vi "COD主界面（列队使用）.vi"() -> (8 "多列列表框":i32(listbox))   [LabVIEW 2016, in "斯坦道CODMn.lvlib"]
uses:
  <vilib>/Analysis/6fits.llb/Curve Fitting Criteria.ctl
  <vilib>/Utility/miscctls.llb/LVPointTypeDef.ctl
  <vilib>/Utility/config.llb/Read Key (I32).vi
  <vilib>/Utility/config.llb/Read Key (Double).vi
  <vilib>/Utility/config.llb/Read Key (Boolean).vi
  <vilib>/Utility/config.llb/Write Key (I32).vi
  <vilib>/Utility/config.llb/Read Key (String).vi
  <vilib>/Utility/config.llb/Write Key (Double).vi
  <vilib>/Utility/config.llb/Write Key (Boolean).vi
  <vilib>/Utility/config.llb/Write Key (String).vi
  <vilib>/Waveform/WDTFileIO.llb/Read Waveform from File.vi
  <vilib>/ptbypt/NI_PtbyPt.lvlib
  <vilib>/Utility/config.llb/NI_LVConfig.lvlib
  <vilib>/Analysis/NI_AALPro.lvlib
panel:
  in  "方程系数 2":cluster{"K":dbl, "b":dbl, "X^2":dbl} {"X^2" format="%#.6g"; "b" format="%#.6g"; "K" format="%#.6g"}
  out "r^2 2":dbl caption="r^2" format="%.8g"
  out "拟合公式 2":string
  in  "跨度值":dbl
  in  "公式切换阈值滴定数(0-9999)":u16
  out "公式系数":dbl[](array[numeric])
  in  "存校准信息":bool
  out "标液校准时间4":timestamp format="%<%Y/%m/%d %H:%M:%S>T"
  out "标液校准时间3":timestamp format="%<%Y/%m/%d %H:%M:%S>T"
  out "标液校准时间2":timestamp format="%<%Y/%m/%d %H:%M:%S>T"
  out "标液校准时间1":timestamp format="%<%Y/%m/%d %H:%M:%S>T"
  out "零点校准时间":timestamp format="%<%Y/%m/%d %H:%M:%S>T"
  in  "远程标样校准":enum16{"标液1", "标液2", "标液3", "标液4"}(ring)
  in  "远程校准量程":enum16{"低量程", "高量程"}(ring)
  in  "温度曲线":bool
  out "温度波形时间":timestamp
  in  "历史波形 2":bool
  out "时间-温度":u16[](array[numeric]) caption="数组"
  in  "关闭 4":bool
  out "时间温度曲线":u16[](graph)
  in  "加标回收量程：":enum32{"H", "L", "AUTO"}(ring)=enum."AUTO"
  in  "定时设置":cluster{"启动":bool, "控制命令":T1, "测量参数":T2}(xcontrol)
  out "氢氧化钠":dbl
  in  "序列号变更":bool
  out "模块版本号":string
  in  "更新程序":bool
  out "进样无液体告警":bool
  out "校准内容显示":string
  out "60分钟超时报警":bool
  in  "仪器参数":bool
  out "CODMn序列号":string
  out "CODMn软件版本：":string
  in  "标样核查量程选择":enum32{"H", "L", "AUTO"}(ring)=enum."AUTO"
  in  "标样浓度":dbl
  in  "零点核查量程选择":enum32{"H", "L", "AUTO"}(ring)=enum."AUTO"
  in  "零点核查浓度":dbl
  out "序列号":string
  in  "采水泵排液时间/s:":i32
  in  "采水泵润洗时间/s:":i32
  in  "采水泵沉淀时间/s:":i32
  in  "采水泵进样时间/s:":i32
  in  "常规版/认证版":enum16{"常规版-酸性", "常规版-碱性", "认证版", "浮台版"}(ring)
  in  "释放串口":bool
  in  "打开串口":bool
  in  "保存参数":dbl[](array[numeric])
  out "报警数字":i16
  out "CODMn工作状态":T3(ring)
  out "ORP-K":string
  out "ORP-B":string
  out "ORP-A":string
  out "x = y?":bool
  out "稀释倍数解释":string
  in  "跨度量程选择":enum32{"H", "L", "AUTO"}(ring)=enum."AUTO"
  in  "跨度液浓度":dbl
  in  "水样：":dbl
  in  "蒸馏水：":dbl
  in  "标液：":dbl
  in  "零点核查样：":dbl
  in  "加标回收样：":dbl
  in  "草酸钠":dbl
  in  "高锰酸钾":dbl
  in  "硫酸":dbl
  out "量程解释说明":string
  in  "高切低阈值:":dbl
  in  "低切高阈值:":dbl
  in  "水样量程选择:":enum16{"L", "H", "自动切换测一次", "自动切换测两次"}(ring)
  in  "氢氧化钠：":dbl
  in  "标准液浓度":dbl
  in  "温度":dbl
  in  "恒温时间":dbl
  in  "当前量程：":enum16{"L", "H"}(ring)
  in  "CODMn零点核查选择":enum16{"零点核查走纯水管", "零点核查走零漂管"}(ring)
  in  "锁定按钮":bool
  in  "低量程稀释倍数:":i8=1
  in  "高量程稀释倍数:":i8=2
  out "基本量程(显示)":string
  out "测量模式(显示)":string
  out "数据时间":string
  out "断电排液标记":bool
  out "COM":string
  in  "启用5":bool
  in  "校准5":bool
  in  "泵滴定数5":dbl
  in  "浓度5":dbl
  in  "启用4":bool
  in  "校准4":bool
  in  "泵滴定数4":dbl
  in  "浓度4":dbl
  out "波形时间":timestamp
  in  "历史波形":bool
  out "滴定数-ORP值":u16[](array[numeric]) caption="数组"
  in  "关闭 3":bool
  in  "滴定曲线":bool
  out "ORP滴定曲线":u16[](graph)
  out "空白测试标记":bool
  out "跨度核查标记":bool
  in  "量程选择":enum16{"低量程", "高量程"}(ring)
  in  "手动控制":bool
  in  "选用水样":enum16{"葡萄糖", "草酸钠"}(ring)
  in  "方程系数":cluster{"K":dbl, "b":dbl, "X^2":dbl} {"X^2" format="%#.6g"; "b" format="%#.6g"; "K" format="%#.6g"}
  out "XY图":cluster{"X Values":dbl[], "Y Values":dbl[]}[](graph)
  in  "模型":enum32{"线性", "多项式", "折线"}(ring)
  out "启动时间":timestamp format="%<%Y/%m/%d %H:%M:%S>T"
  in  "关闭 2":bool
  out "r^2":dbl format="%.8g"
  out "拟合公式":string
  in  "启用3":bool
  in  "启用2":bool
  in  "启用1":bool
  in  "校准3":bool
  in  "校准2":bool
  in  "校准1":bool
  in  "泵滴定数3":dbl
  in  "泵滴定数2":dbl
  in  "泵滴定数1":dbl
  in  "浓度3":dbl
  in  "浓度2":dbl
  in  "浓度1":dbl
  in  "写入":bool
  out "零点核查标记":bool
  out "排液故障":bool
  out "进水样超量程":bool
  out "标样核查标记":bool
  out "平行样测量":bool
  out "加标回收测量":bool
  out "质控样测量":bool
  out "待机":bool
  out "校标错误":bool
  out "校零错误":bool
  out "测量错误":bool
  out "草酸钠报警":bool
  out "高锰酸钾报警":bool
  out "加热故障":bool
  out "温控器故障":bool
  out "ORP故障":bool
  out "排液标记":bool
  out "故障标记":bool
  out "校标标记":bool
  out "校零标记":bool
  out "通讯状态":bool
  out "水样测量":bool
  in  "读取":bool
  in  "返回":bool
  in  "校准配置":bool
  in  "零点泵计量数 2":dbl
  in  "标度泵计量数 2":dbl
  out "标度滴定值":dbl
  out "零点滴定值":dbl
  in  "保存":bool
  in  "关闭":bool
  out "仪器时间":timestamp format="%<%Y/%m/%d %H:%M:%S>T"
  out "秒":u16
  out "分":u16
  out "COD浓度（mg/L)":dbl format="%.2g"
  out "进样管":dbl
  out "高锰酸钾":dbl
  out "草酸钠":dbl
  out "硫酸":dbl
  out "实时ORP":dbl
  out "温度℃":dbl
  out "加热":bool
  out "搅拌":bool
  out "进硫酸":bool
  out "进加标回收样":bool
  out "进零点核查样":bool
  out "进标液":bool
  out "进蒸馏水":bool
  out "进水样":bool
  out "进草酸钠":bool
  out "进高锰酸钾":bool
  in  "启动":bool
  in  "故障清除":bool
  in  "参数配置":bool
  in  "停止":bool
  in  "单步启动":bool
  out "系统时间":timestamp
  in  "时间校准":bool
  out "模式（受控）":u16
  # "测试时长："
  # "注：遇到加热故障和排液故障时仪器不能正常启动，\n必须排查故障并点击报警清除按钮方可运行。"
  # "mg/L"
  # "基本参数设置"
  # "校零校标结果"
  # "泵计量参数设置"
  # "校零结果："
  # "校零滴定值："
  # "高锰酸钾："
  # "加热恒温温度(℃):"
  # "草酸钠："
  # "校标结果："
  # "标度滴定值："
  # "恒温时间(分钟):"
  # "零点泵计量值："
  # "硫酸："
  # "标准液浓度(mg/L):"
  # "标度泵计量值："
  # "跨度核查浓度："
  # "跨度核查量程："
  # "零点核查浓度："
  # "标样浓度："
  # "零点核查量程："
  # "标样核查量程："
  # "跨度值:"
  # "校准配置界面"
  # "测量信号值"
  # "启用"
  # "校准时间"
  # "浓度"
  # "零点"
  # "标液1"
  # "标液2"
  # "标液3"
  # "标液4"
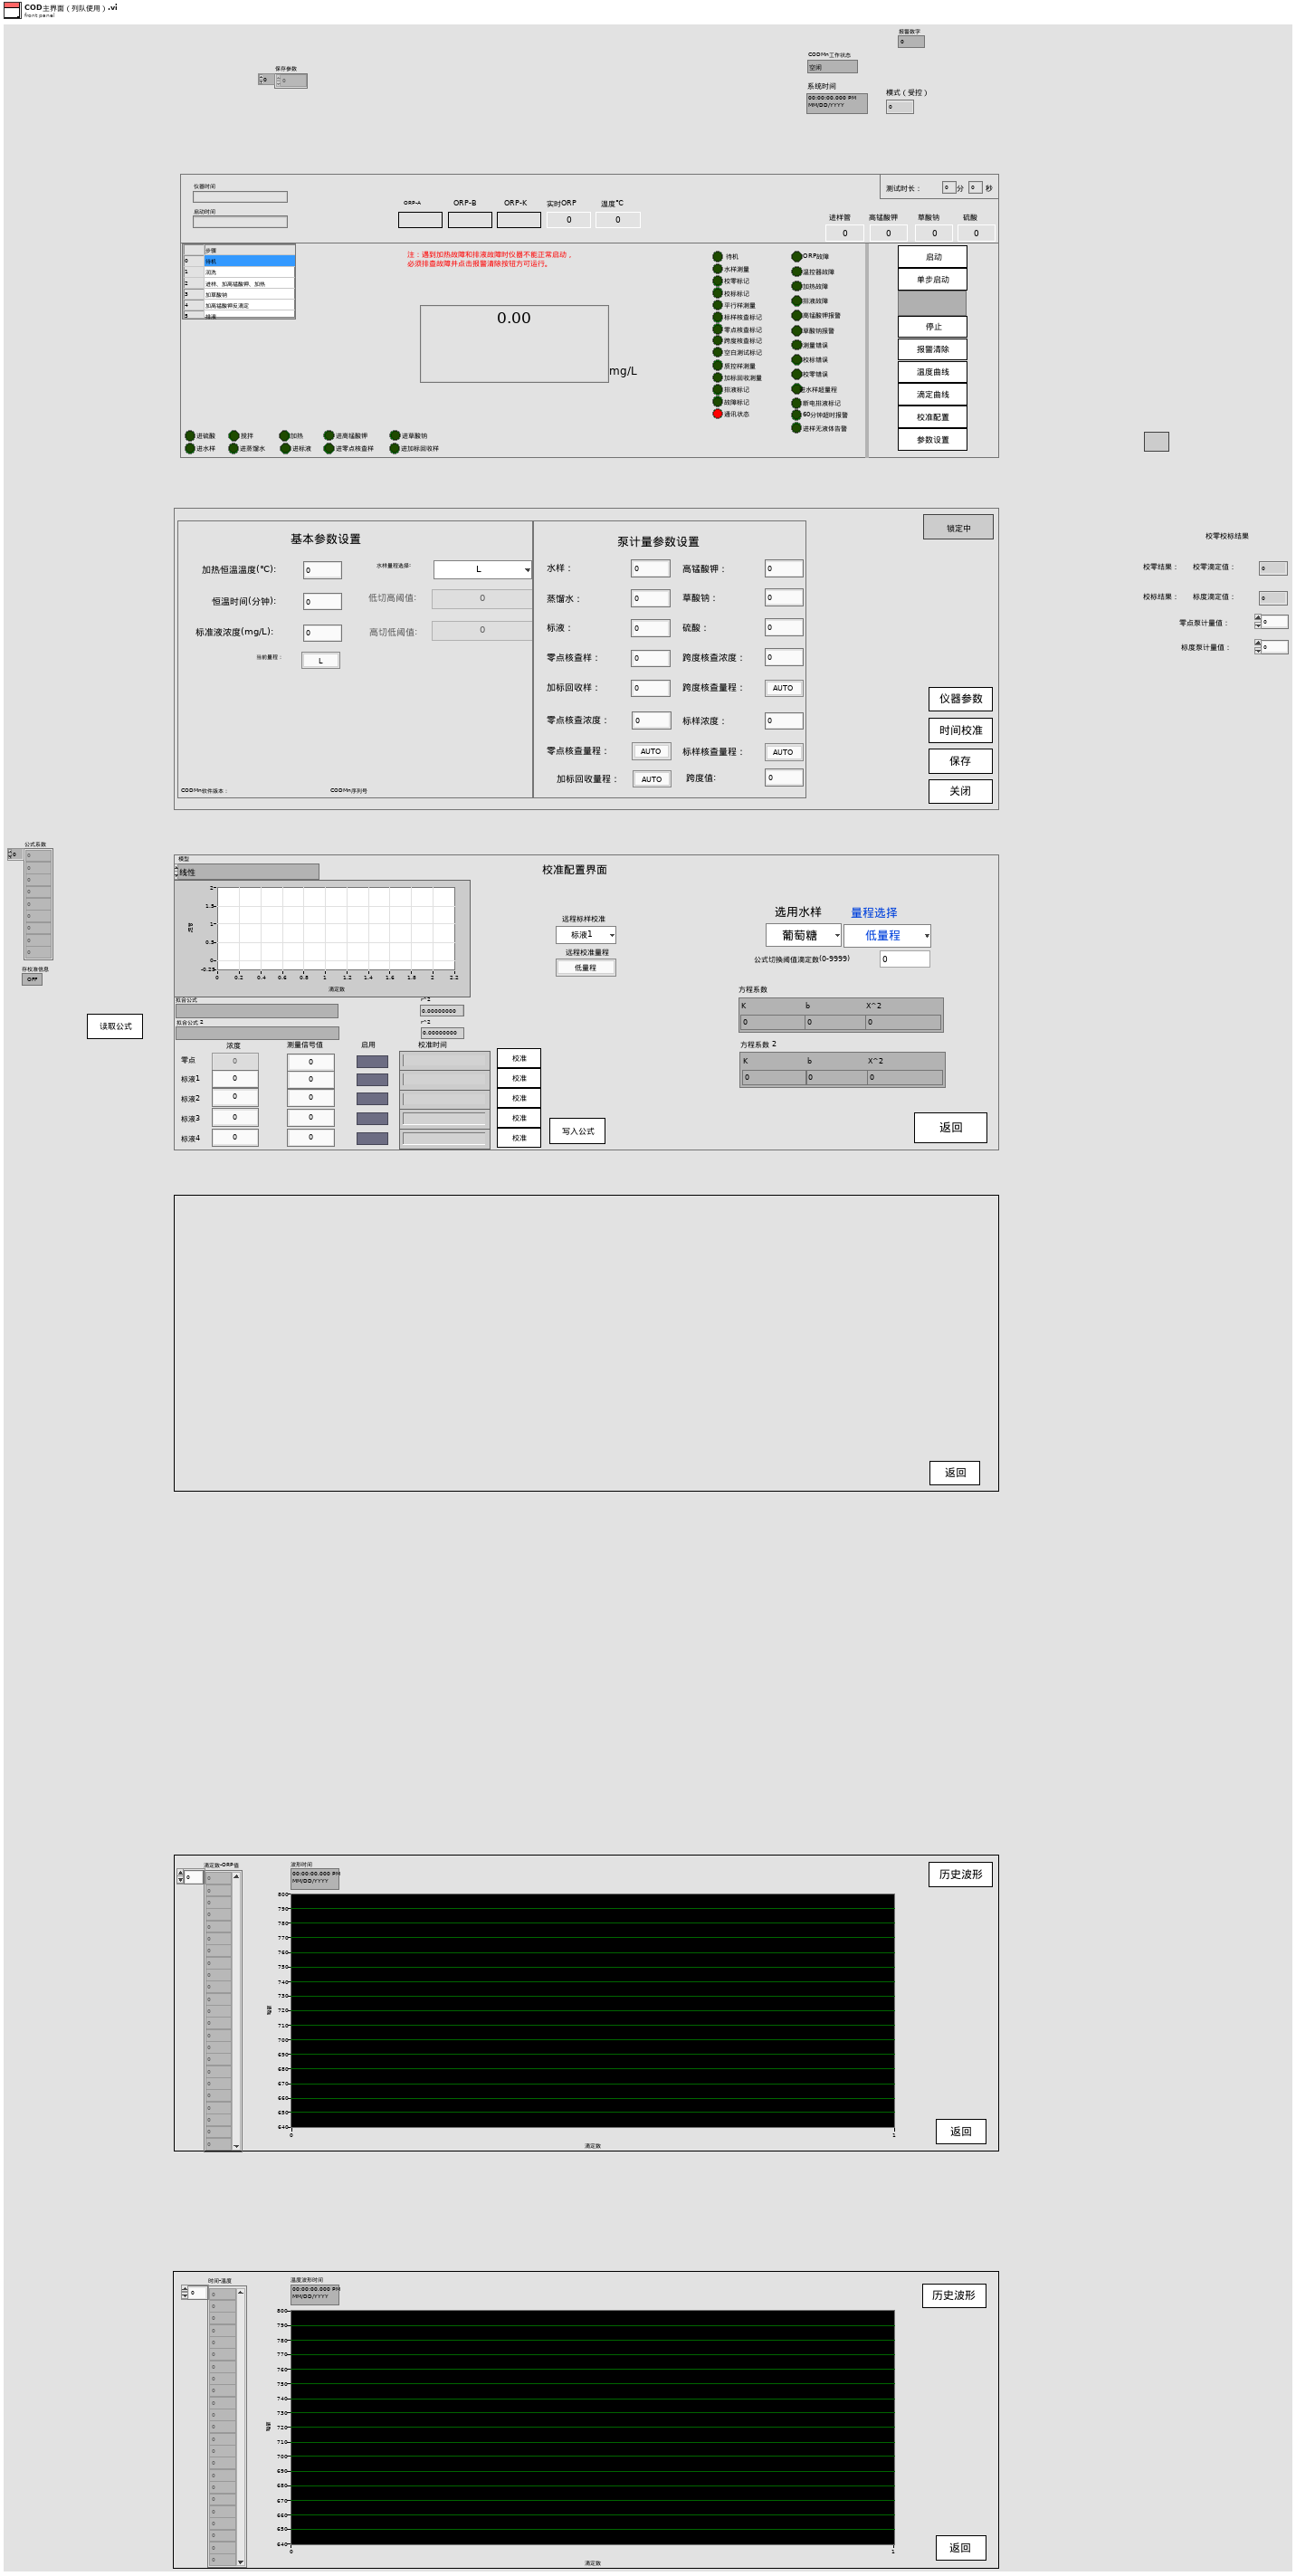
[diagram p1: front panel]
types:
  T1 = typedef "定时设置.xctl/国标控制命令.ctl" = enum16{"启动测量", "标样核查", "零点核查", "跨度核查", "空白测试", "平行样测试", "加标回收", "空白校准", "标样校准", "初始化（清洗）", "停止测试", "仪器重启", "校时", "模式设置", "测量间隔设置"}
  T2 = typedef "定时设置.xctl/测量参数.ctl" = u16
  T3 = enum16{"空闲", "水样测试", "标样核查", "零点核查", "跨度核查", "空白测试", "平行样测试", "质控样", "空白校准", "标样校准", "加标回收"}
  T4 = typedef "LVPointTypeDef.ctl" = cluster{"Horizontal":i16, "Vertical":i16}
  T5 = cluster{"Major":u16, "Minor":u16, "Fix":u16, "Build":u16}
  T6 = typedef "NI_LVConfig.lvlib/Config Data RefNum.ctl" = refnum<k1>
  T7 = cluster{"时间源选择":enum16{"系统时间源", "仪器时间源"}, "外部时间源":timestamp}
  T8 = enum32{"Bad", "Idle", "Run top level", "Running"}
  T9 = enum8{"Enabled", "Disabled", "Disabled and Grayed Out"}
  T10 = cluster{"时间":timestamp, "测量模式":string, "数据类型":string, "检测值":sgl, "单位":string, "数据标识":string, "因子编码":string, "标样参考值":sgl, "ORP-A":sgl, "ORP-B":sgl, "ORP-K":sgl, "COD滴定值":sgl, "高锰酸钾滴定数":sgl, "温度":sgl, "量程":sgl, "LastTime":timestamp, "序列号:":string, "跨度值":sgl}
  T11 = cluster{"因子编码":u32, "单位":u16, "标样参考值":sgl, "水样数据时间":timestamp, "水样实测值":sgl, "水样数据标识":string, "标样数据时间":timestamp, "标样实测值":sgl, "标样数据标识":string, "空白数据时间":timestamp, "空白实测值":sgl, "空白数据标识":string, "零点核查数据时间":timestamp, "零点核查实测值":sgl, "零点核查数据标识":string, "跨度核查数据时间":timestamp, "跨度核查实测值":sgl, "跨度核查数据标识":string, "加标回收数据时间":timestamp, "加标回收实测值":sgl, "加标回收数据标识":string, "平行样数据时间":timestamp, "平行样实测值":sgl, "平行样数据标识":string}
  T12 = cluster{"测量量程":dbl, "测量精度":dbl, "测量间隔":dbl, "消解温度":dbl, "消解时长":dbl, "空白校准时间":timestamp, "曲线截距":dbl, "曲线斜率":dbl, "测量检出限":dbl, "测量信号值":dbl, "线性相关系数":dbl, "二次多项式系数":dbl, "标样校准时间":timestamp, "稀释倍数":dbl, "三项式系数":dbl, "空白标定系数":dbl, "量程系数":dbl, "F0/ORPA":dbl, "F1/ORPB":dbl, "F2/ORPK":dbl, "F3":dbl, "F4":dbl, "F5":dbl, "F6":dbl, "F7":dbl, "X0/滴定数":dbl, "量程":dbl}
  T13 = cluster{"运行模式":enum16{"维护模式", "常规模式", "应急模式", "质控模式"}, "质控频次":enum16{"关闭", "每天", "星期一", "星期二", "星期三", "星期四", "星期五", "星期六", "星期日"}, "空白核查时间":u16, "跨度核查时间":u16, "24H周期设置":bool[]}
  T14 = cluster{"数组 2[0]":sgl, "数组 2[1]":sgl, "数组 2[2]":sgl, "数组 2[3]":sgl, "数组 2[4]":sgl, "数组 2[5]":sgl, "数组 2[6]":sgl, "数组 2[7]":sgl, "数组 2[8]":sgl, "数组 2[9]":sgl, "数组 2[10]":sgl, "数组 2[11]":sgl, "数组 2[12]":sgl, "数组 2[13]":sgl, "数组 2[14]":sgl, "数组 2[15]":sgl, "数组 2[16]":sgl, "数组 2[17]":sgl, "数组 2[18]":sgl, "数组 2[19]":sgl, "数组 2[20]":sgl, "数组 2[21]":sgl, "数组 2[22]":sgl, "数组 2[23]":sgl, "数组 2[24]":sgl, "数组 2[25]":sgl, "数组 2[26]":sgl, "数组 2[27]":sgl, "数组 2[28]":sgl, "数组 2[29]":sgl, "数组 2[30]":sgl, "数组 2[31]":sgl, "数组 2[32]":sgl, "数组 2[33]":sgl, "数组 2[34]":sgl, "数组 2[35]":sgl, "数组 2[36]":sgl, "数组 2[37]":sgl, "数组 2[38]":sgl, "数组 2[39]":sgl, "数组 2[40]":sgl, "数组 2[41]":sgl}
  T15 = typedef "NI_AALPro.lvlib/Curve Fitting Criteria.ctl" = u16
  T16 = cluster{"ORP故障":bool, "温控器故障":bool, "加热故障":bool, "高锰酸钾报警":bool, "草酸钠报警":bool, "测量错误":bool, "校零错误":bool, "校标错误":bool, " 进水样超量程":bool, "排液阀故障":bool, "60分钟超时报警":bool, "进样无液体报警":bool}
  T17 = cluster{"时间标识":timestamp, "参数":string, "日志信息":string, "流程参数":string}
  T18 = cluster{"确定":bool, "测量量程":dbl, "测量精度":dbl, "测量间隔":dbl, "消解温度":dbl, "消解时长":dbl, "空白校准时间":timestamp, "曲线截距":dbl, "曲线斜率":dbl, "测量检出限":dbl, "测量信号值":dbl, "线性相关系数":dbl, "二次多项式系数":dbl, "标样校准时间":timestamp, "稀释倍数":dbl, "三项式系数":dbl, "空白标定系数":dbl, "量程系数":dbl, "F0/ORPA":dbl, "F1/ORPB":dbl, "F2/ORPK":dbl, "F3":dbl, "F4":dbl, "F5":dbl, "F6":dbl, "F7":dbl, "X0/滴定数":dbl, "量程":dbl}
  T19 = cluster{"时间标识":timestamp, "设备":string, "日志信息":string, "流程参数":string}
  T20 = cluster{"[0]":string, "[1]":string, "[2]":string}
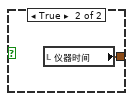
[diagram p3: hidden frame]
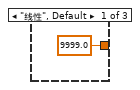
[diagram p9: hidden frame]
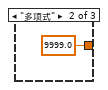
[diagram p10: hidden frame]
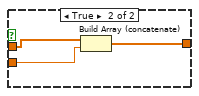
[diagram p11: hidden frame]
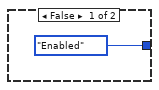
[diagram p12: hidden frame]
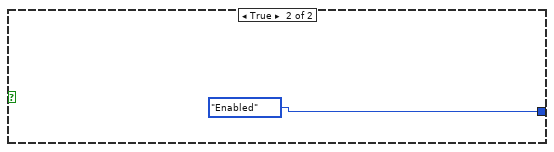
[diagram p13: hidden frame]
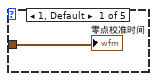
[diagram p18: hidden frame]
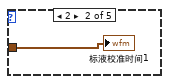
[diagram p19: hidden frame]
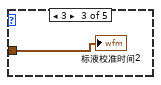
[diagram p20: hidden frame]
diagram:
  n1 = flat-sequence {
    tunnel: w3 -> [_]
    frame #0 {
      n2 = vi-ref "斯坦道CODMn.lvlib:待机状态数据存储写入和切换量程(子VI).vi"() -> (w64:refnum<vi>)
      n3 = vi-ref "斯坦道CODMn.lvlib:日志报警状态存储 (子VI).vi"() -> (w57:refnum<vi>)
      n4 = vi-ref "斯坦道CODMn.lvlib:高锰酸钾-ORP滴定曲线(子VI).vi"() -> (w44:refnum<vi>)
      n5 = property class="VI"(reference=w57, error in=errorcluster {"status"=FALSE, "code"=0, "source"=""} ("错误输出")) -> ("Name"=w56:string)  [unwired: 2 out]
      n6 = property class="VI"(reference=w44, error in=errorcluster {"status"=FALSE, "code"=0, "source"=""} ("错误输出")) -> ("Name"=w45:string)  [unwired: 2 out]
      n7 = property class="VI"(reference=w64, error in=errorcluster {"status"=FALSE, "code"=0, "source"=""} ("错误输出")) -> ("Name"=w63:string)  [unwired: 2 out]
      n8 = Open VI Reference(type specifier VI Refnum (for type only)=refnum<vi> refnum, vi path=w56, options=128 ("选项")) -> (vi reference=w40:refnum<vi>, error out=w54:errorcluster)  [unwired: 3 in]
      n9 = Open VI Reference(type specifier VI Refnum (for type only)=refnum<vi> refnum, vi path=w45, options=128 ("选项")) -> (vi reference=w43:refnum<vi>, error out=w47:errorcluster)  [unwired: 3 in]
      n10 = call-by-ref "?"(reference=w40, error in=w54) -> (reference out=w52:refnum<vi>, error out=w53:errorcluster)  [unwired: 12 in]
      n11 = call-by-ref "?"(reference=w43, error in=w47) -> (reference out=w49:refnum<vi>, error out=w48:errorcluster)  [unwired: 12 in]
      n12 = Open VI Reference(type specifier VI Refnum (for type only)=refnum<vi> refnum, vi path=w63, options=128 ("选项")) -> (vi reference=w38:refnum<vi>, error out=w61:errorcluster)  [unwired: 3 in]
      n13 = Close Reference(reference=w52, error in (no error)=w53) -> ()  [unwired: 1 out]
      n14 = call-by-ref "?"(reference=w38, error in=w61) -> (reference out=w59:refnum<vi>, error out=w60:errorcluster)  [unwired: 12 in]
      n15 = Close Reference(reference=w49, error in (no error)=w48) -> ()  [unwired: 1 out]
      n16 = Close Reference(reference=w59, error in (no error)=w60) -> ()  [unwired: 1 out]
      n17 = vi-ref "斯坦道CODMn.lvlib:时间-温度曲线(子VI).vi"() -> (w26:refnum<vi>)
      n18 = vi-ref "斯坦道CODMn.lvlib:关键参数交互.vi"() -> (w35:refnum<vi>)
      n19 = property class="VI"(reference=w35, error in=errorcluster {"status"=FALSE, "code"=0, "source"=""} ("错误输出")) -> ("Name"=w34:string)  [unwired: 2 out]
      n20 = property class="VI"(reference=w26, error in=errorcluster {"status"=FALSE, "code"=0, "source"=""} ("错误输出")) -> ("Name"=w25:string)  [unwired: 2 out]
      n21 = Open VI Reference(type specifier VI Refnum (for type only)=refnum<vi> refnum, vi path=w34, options=128 ("选项")) -> (vi reference=w36:refnum<vi>, error out=w32:errorcluster)  [unwired: 3 in]
      n22 = call-by-ref "?"(reference=w36, error in=w32, "量程选择"=enum16{"低量程", "高量程"}."低量程", "模型"=enum32{"线性", "多项式", "折线"}."线性") -> (reference out=w30:refnum<vi>, error out=w31:errorcluster)  [unwired: 10 in]
      n23 = Open VI Reference(type specifier VI Refnum (for type only)=refnum<vi> refnum, vi path=w25, options=128 ("选项")) -> (vi reference=w27:refnum<vi>, error out=w23:errorcluster)  [unwired: 3 in]
      n24 = call-by-ref "?"(reference=w27, error in=w23) -> (reference out=w21:refnum<vi>, error out=w22:errorcluster)  [unwired: 12 in]
      n25 = Close Reference(reference=w30, error in (no error)=w31) -> ()  [unwired: 1 out]
      n26 = Close Reference(reference=w21, error in (no error)=w22) -> ()  [unwired: 1 out]
    }
  }
  n27 = property on="定时设置" class="定时设置 (严格)"("引用参数"="CODMn") -> (error out=w1:errorcluster)  [unwired: 2 in, 1 out]
  n28 = flat-sequence {
    tunnel: [w68] -> w5
    tunnel: [errorcluster {"status"=FALSE, "code"=0, "source"=""} ("错误输出")] -> w3
    tunnel: [w70] -> w4
    frame #0 {
      w92 = "192.168.1.100" ("名称")
      n29 = global write "COD内部交互全局.vi" "量程切换次数"(u8 0 ("量程切换次数")) -> ()
      n30 = global write "COD内部交互全局.vi" "切换量程连续测两次"(FALSE ("切换量程连续测两次")) -> ()
      n31 = global read "COD内部交互全局.vi" "序列号:"() -> (w99:string)
      n32 = property on="窗格" class="Pane"("Origin"=T4 {"Horizontal"=0, "Vertical"=0} ("原点")) -> ()  [unwired: 2 in, 2 out]
      n33 = Empty String/Path?(string/path=w99) -> (empty?=w67:bool)
      n34 = case shown="真" w67 {
        tunnel: w99 -> [w113 _]
        tunnel: [w112 "data\\CODMnSet.ini" ("名称或相对路径")] -> w80
        frame False {
          # "与生产用上位机交互"
          n35 = Concatenate Strings("data\\" ("字符串"), "序列号" ("字符串"), w113, "Set.ini" ("名称或相对路径")) -> (w112:string)
        }
        frame True {
        }
      }
      n36 = String To IP(1:w92) -> (0:w85:u32)
      n37 = IP To String(2:w85) -> (0:w88:string)  [unwired: 1 in]
      n38 = Not Equal?(x=w92, y=w88) -> (x != y?=w93:bool)
      n39 = Concatenate Strings("\\\\" ("字符串"), w88) -> (w87:string)
      n40 = global write "CODMN外部API.vi" "ping"(w93) -> ()
      n41 = String To Path(string=w87) -> (path=w94:path)
      n42 = Build Path(base path=w94, name or relative path=w80) -> (appended path=w89:path)
      n43 = local write "量程选择"(enum16{"低量程", "高量程"}."低量程" ("量程选择")) -> ()
      n44 = local write "选用水样"(enum16{"葡萄糖", "草酸钠"}."葡萄糖" ("选用水样")) -> ()
      n45 = global write "COD内部交互全局.vi" "配置文件ini"(w80) -> ()
      n46 = case shown="真" w93 {
        tunnel: w89 -> [w103 w107]
        tunnel: [w103 w106] -> w90
        tunnel: [FALSE w105] -> w91
        frame False {
        }
        frame True {
          n47 = call <vilib>:"Check if File or Folder Exists.vi"("path"=w107) -> ("file or folder exists?"=w105:bool, "dup path"=w106:path)  [unwired: 8 in, 1 out]
        }
      }
      n48 = control-ref of="本VI"() -> (w79:refnum<vi>)
      n49 = case shown="假" w91 {
        tunnel: w90 -> [_ w111]
        tunnel: [w109 w111] -> w71
        tunnel: w80 -> [w108 _]
        frame False {
          # "本地文件地址"
          n50 = call <vilib>:"Application Directory.vi"() -> ("Application Directory"=w110:path)
          n51 = Build Path(base path=w110, name or relative path=w108) -> (appended path=w109:path)
        }
        frame True {
          # "网络共享地址"
        }
      }
      n52 = property class="VI"(reference=w79) -> ("Library.Version"=w78:T5)  [unwired: 1 in, 2 out]
      n53 = Unbundle By Name(w78) -> ("Major"=w76:u16, "Minor"=w75:u16, "Fix"=w74:u16, "Build"=w73:u16)
      n54 = Format Into String(format string="模块版本号：%d.%d.%d.%d" ("格式字符串"), w76, w75, w74, w73) -> (resulting string=→"模块版本号":string)  [unwired: 2 in, 1 out]
      n55 = global write "CODMN外部API.vi" "配置文件 path"(w71) -> ()
      n56 = call <vilib>:"Open Config Data.vi"("configuration file path"=w71) -> ("error out"=w81:errorcluster, "refnum"=w82:T6)  [unwired: 8 in, 1 out]
      n57 = vi-ref "斯坦道CODMn.lvlib:CODMn断电保存全局变量.vi"() -> (w95:refnum<vi>)
      n58 = call <userlib>:"Read Panel from INI__ogtk.vi"("error in (no error)"=w81, "VI ref"=w95, "refnum"=w82) -> ("error out"=w83:errorcluster, "refnum out"=w84:T6)  [unwired: 7 in]
      n59 = call <vilib>:"Close Config Data.vi"("error in (no error)"=w83, "refnum"=w84) -> ("error out"=w69:errorcluster)  [unwired: 8 in, 1 out]
      n60 = call <vilib>:"Clear Errors.vi"("error in (no error)"=w69) -> ("error out"=w66:errorcluster)  [unwired: 5 in, 1 out]
      n61 = Read from Text File(file (use dialog)=w71, error in=w66) -> (text=w70:string, error out=w68:errorcluster)  [unwired: 2 in, 2 out]
      "稀释倍数解释" <- "稀释倍数解释：\n稀释倍数选择1，表示不稀释\n默认低量程系数倍数1，高量程系数倍数2\n则低量程为0~8，高量程为0~16" ("稀释倍数解释")
    }
  }
  n62 = while {
    tunnel: w1 -> [_]
    stop <- FALSE stop-if-true
    n63 = Wait (ms)(milliseconds to wait=u32 500 ("等待时间（毫秒）")) -> ()  [unwired: 1 out]
    n64 = global read "COD测量模式全局.vi" "CODMn工作状态"() -> (w124:T3)
    n65 = local read "通讯状态"() -> (w118:bool)
    n66 = case shown="假" w118 {
      tunnel: [w134 w135] -> w122
      frame False {
        n67 = Get Date/Time In Seconds() -> (seconds since 1Jan1904=w134:timestamp)
      }
      frame True {
        n68 = local read "仪器时间"() -> (w135:timestamp)
      }
    }
    n69 = vi-ref "斯坦道CODMn.lvlib:CODMn测量流程.vi"() -> (w131:refnum<vi>)
    n70 = Bundle By Name(cluster=T7 {"时间源选择"=enum."系统时间源", "外部时间源"=timestamp(0 s since 1904-01-01)} ("时间源"), "时间源选择"=enum16{"系统时间源", "仪器时间源"}."仪器时间源", "外部时间源"=w122) -> (w120:T7)
    n71 = property class="VI"(reference=w131) -> ("Exec.State"=w129:T8, "Name"=w130:string)  [unwired: 1 in, 2 out]
    n72 = Not Equal?(x=w124, y=T3."空闲") -> (x != y?=w119:bool)
    n73 = property on="定时设置" class="定时设置 (严格)"("仪器状态"=w119, "时间源"=w120) -> ()  [unwired: 2 in, 2 out]
    n74 = Unbundle By Name("定时设置") -> ("启动"=w127:bool, "控制命令"=w128:T1)
    n75 = case shown="真" w127 {
      tunnel: w130 -> [_ w138]
      tunnel: w128 -> [_ w137]
      tunnel: w129 -> [_ w136]
      frame False {
      }
      frame True {
        n76 = case shown="\"Idle\"" w136 {
          tunnel: w138 -> [_ w142]
          tunnel: w137 -> [_ w139]
          frame "Bad", Default {
          }
          frame "Idle" {
            n77 = Open VI Reference(type specifier VI Refnum (for type only)=refnum<vi> refnum, vi path=w142, options=128 ("选项")) -> (vi reference=w143:refnum<vi>, error out=w144:errorcluster)  [unwired: 3 in]
            n78 = call-by-ref "开始异步调用"(reference=w143, error in=w144, "控制命令"=w139) -> (reference out=w145:refnum<vi>, error out=w146:errorcluster)  [unwired: 11 in]
            n79 = Close Reference(reference=w145, error in (no error)=w146) -> ()  [unwired: 1 out]
          }
        }
      }
    }
  }
  n80 = Obtain Queue(name (unnamed)="CODMn" ("名称（未命名）"), element data type=cluster{"命令":string} {"命令"="启用模块"} ("元素")) -> (queue out=w15:refnum<queue>, error out=w14:errorcluster)  [unwired: 3 in, 1 out]
  n81 = while {
    tunnel: [w153] -> _
    shift-right: [w151] -> _
    shift-left: w4 -> [w150]
    tunnel: w5 -> [_]
    stop <- FALSE stop-if-true
    n82 = global read "CODMN外部API.vi" "配置文件 path"() -> (w147:path)
    n83 = Wait (ms)(milliseconds to wait=u32 1000 ("等待时间（毫秒）")) -> ()  [unwired: 1 out]
    n84 = Read from Text File(file (use dialog)=w147) -> (text=w151:string, error out=w148:errorcluster)  [unwired: 3 in, 2 out]
    n85 = Not Equal?(x=w151, y=w150) -> (x != y?=w149:bool)
    n86 = case shown="真" w149 {
      tunnel: [w155 w162] -> w153
      tunnel: w147 -> [_ w156]
      tunnel: w148 -> [w155 _]
      frame False {
      }
      frame True {
        # "文件发生改变进行更新，远端和本地都更新"
        n87 = vi-ref "斯坦道CODMn.lvlib:CODMn断电保存全局变量.vi"() -> (w157:refnum<vi>)
        n88 = call <vilib>:"Open Config Data.vi"("configuration file path"=w156) -> ("error out"=w161:errorcluster, "refnum"=w160:T6)  [unwired: 8 in, 1 out]
        n89 = call <userlib>:"Read Panel from INI__ogtk.vi"("error in (no error)"=w161, "VI ref"=w157, "refnum"=w160) -> ("error out"=w159:errorcluster, "refnum out"=w158:T6)  [unwired: 7 in]
        n90 = call <vilib>:"Close Config Data.vi"("error in (no error)"=w159, "refnum"=w158) -> ("error out"=w162:errorcluster)  [unwired: 8 in, 1 out]
      }
    }
  }
  n91 = vi-ref "CODMn通讯.vi"() -> (w6:refnum<vi>)
  n92 = while {
    stop <- FALSE stop-if-true
    n93 = global read "COD内部交互全局.vi" "待机"() -> (w164:bool)
    n94 = Wait (ms)(milliseconds to wait=u32 1000 ("等待时间（毫秒）")) -> ()  [unwired: 1 out]
    n95 = case shown="假" w164 {
      tunnel: [w181 T9."Enabled" ("禁用")] -> w166
      tunnel: [w180 _] -> w165
      frame False {
        # "运行中"
        n96 = local read "校标标记"() -> (w179:bool)
        n97 = local read "校零标记"() -> (w178:bool)
        n98 = Or(x=w179, y=w178) -> (x .or. y?=w182:bool)
        n99 = case shown="真" w182 {
          tunnel: [T9."Enabled" ("禁用") T9."Disabled and Grayed Out" ("禁用")] -> w181
          tunnel: [_ TRUE] -> w180
          frame False {
          }
          frame True {
          }
        }
      }
      frame True {
      }
    }
    n100 = control-ref of="量程选择"() -> (w172:refnum<vi>)
    n101 = property on="校准内容显示" class="Str"("Visible"=w165) -> ()  [unwired: 2 in, 2 out]
    n102 = control-ref of="选用水样"() -> (w173:refnum<vi>)
    n103 = control-ref of="校准5"() -> (w167:refnum<vi>)
    n104 = control-ref of="校准4"() -> (w168:refnum<vi>)
    n105 = control-ref of="校准3"() -> (w169:refnum<vi>)
    n106 = control-ref of="校准2"() -> (w170:refnum<vi>)
    n107 = control-ref of="校准1"() -> (w171:refnum<vi>)
    n108 = Build Array(w167, w168, w169, w170, w171, w173, w172) -> (w174:refnum<vi>[])
    n109 = for {
      tunnel: w174 -> [w177] mode=indexing
      tunnel: w166 -> [w176]
      n110 = property class="Ctl"(reference=w177, "DisabledEnum"=w176) -> ()  [unwired: 1 in, 2 out]
    }
  }
  n111 = while {
    tunnel: w5 -> [_]
    stop <- FALSE stop-if-true
    # "赋值循环"
    n112 = flat-sequence {
      frame #0 {
        # "测量数据区"
        n113 = global read "COD内部交互全局.vi" "data"() -> (w326:T10)
        n114 = global read "COD测量模式全局.vi" "测量模式文字实时"() -> (w312:string)
        "测量模式(显示)" <- w312
        n115 = global read "CODMn断电保存全局变量.vi" "测量数据区"() -> (w321:T11)
        n116 = Unbundle By Name(w326) -> ("时间"=w325:timestamp, "检测值"=w324:sgl, "数据标识"=w323:string)
        n117 = case shown="\"水样测试\"" w312 {
          tunnel: w321 -> [w327 w332 w337 w342 w347 w352 w357 w362 w367 w372]
          tunnel: [w327 w331 w336 w338 w346 w351 w356 w361 w363 w371] -> w322
          tunnel: w325 -> [_ w330 w335 w341 w345 w350 w355 w360 w366 w370]
          tunnel: w324 -> [_ w329 w334 w340 w344 w349 w354 w359 w365 w369]
          tunnel: w323 -> [_ w328 w333 w339 w343 w348 w353 w358 w364 w368]
          frame "", Default {
          }
          frame "水样测试" {
            n118 = Bundle By Name(cluster=w332, "水样数据时间"=w330, "水样实测值"=w329, "水样数据标识"=w328) -> (w331:T11)
          }
          frame "标样核查" {
            n119 = Bundle By Name(cluster=w337, "标样数据时间"=w335, "标样实测值"=w334, "标样数据标识"=w333) -> (w336:T11)
          }
          frame "跨度核查" {
            n120 = Bundle By Name(cluster=w342, "跨度核查数据时间"=w341, "跨度核查实测值"=w340, "跨度核查数据标识"=w339) -> (w338:T11)
          }
          frame "零点核查" {
            n121 = Bundle By Name(cluster=w347, "零点核查数据时间"=w345, "零点核查实测值"=w344, "零点核查数据标识"=w343) -> (w346:T11)
          }
          frame "空白测试" {
            n122 = Bundle By Name(cluster=w352, "空白数据时间"=w350, "空白实测值"=w349, "空白数据标识"=w348) -> (w351:T11)
          }
          frame "加标回收" {
            n123 = Bundle By Name(cluster=w357, "加标回收数据时间"=w355, "加标回收实测值"=w354, "加标回收数据标识"=w353) -> (w356:T11)
          }
          frame "平行样" {
            n124 = Bundle By Name(cluster=w362, "平行样数据时间"=w360, "平行样实测值"=w359, "平行样数据标识"=w358) -> (w361:T11)
          }
          frame "校零" {
            n125 = Bundle By Name(cluster=w367, "空白数据时间"=w366, "空白实测值"=w365, "空白数据标识"=w364) -> (w363:T11)
          }
          frame "校标" {
            n126 = Bundle By Name(cluster=w372, "标样数据时间"=w370, "标样实测值"=w369, "标样数据标识"=w368) -> (w371:T11)
          }
        }
        n127 = Unbundle By Name(w321) -> ("水样实测值"=w318:sgl)
        n128 = feedback-in #1(w321) -> ()
        n129 = feedback #1(w321) -> (w320:T11)
        n130 = global read "CODMn断电保存全局变量.vi" "水样测试量程"() -> (w314:enum16{"L", "H"})
        n131 = Unbundle By Name(w320) -> ("水样实测值"=w319:sgl)
        n132 = feedback #2(w314) -> (w315:enum16{"L", "H"})
        n133 = feedback-in #2(w314) -> ()
        n134 = Not Equal?(x=w315, y=w314) -> (x != y?=w313:bool)
        n135 = Not Equal?(x=w318, y=w319) -> (x != y?=w317:bool)
        n136 = global write "CODMn断电保存全局变量.vi" "测量数据区"(w322) -> ()
        n137 = Or(x=w317, y=w313) -> (x .or. y?=w316:bool)
        n138 = case shown="真" w316 {
          frame False {
          }
          frame True {
            # "水样值发送改变存储本地"
            n139 = call "配置文件保存.vi"() -> ()  [unwired: 12 in]
          }
        }
      }
    }
    n140 = flat-sequence {
      frame #0 {
        # "局部变量给内部交互用全局变量"
        n141 = local read "COD浓度（mg/L)"() -> (w219:dbl)
        n142 = local read "CODMn工作状态"() -> (w222:T3)
        n143 = local read "多列列表框"() -> (w220:i32)
        n144 = local read "标准液浓度"() -> (w218:dbl)
        n145 = local read "温度℃"() -> (w213:dbl)
        n146 = local read "高锰酸钾报警"() -> (w216:bool)
        n147 = local read "断电排液标记"() -> (w215:bool)
        n148 = local read "实时ORP"() -> (w212:dbl)
        n149 = local read "故障标记"() -> (w221:bool)
        n150 = local read "高锰酸钾"() -> (w214:dbl)
        n151 = local read "待机"() -> (w217:bool)
        n152 = global write "COD内部交互全局.vi" "实时温度"(w213) -> ()
        n153 = global write "运行时序全局变量.vi" "多列列表框"(w220) -> ()
        n154 = global write "COD内部交互全局.vi" "故障标记"(w221) -> ()
        n155 = global write "COD内部交互全局.vi" "ORP显示"(w212) -> ()
        n156 = global write "COD浓度全局变量.vi" "标准液浓度"(w218) -> ()
        n157 = global write "COD内部交互全局.vi" "高锰酸钾"(w214) -> ()
        n158 = global write "COD内部交互全局.vi" "待机"(w217) -> ()
        n159 = global write "COD测量模式全局.vi" "CODMn工作状态"(w222) -> ()
        n160 = global write "COD内部交互全局.vi" "高锰酸钾报警"(w216) -> ()
        n161 = global write "COD内部交互全局.vi" "断电排液标记"(w215) -> ()
        n162 = global write "COD浓度全局变量.vi" "COD浓度（mg/L)"(w219) -> ()
      }
    }
    n163 = flat-sequence {
      frame #0 {
        # "断电保存全局给局部变量"
        n164 = global read "CODMn断电保存全局变量.vi" "高切低阈值:"() -> (w392:dbl)
        n165 = global read "CODMn断电保存全局变量.vi" "低切高阈值:"() -> (w391:dbl)
        n166 = global read "CODMn断电保存全局变量.vi" "跨度液浓度"() -> (w389:dbl)
        n167 = global read "COD内部交互全局.vi" "波形时间"() -> (→"波形时间":timestamp)
        n168 = global read "CODMn断电保存全局变量.vi" "启动时间"() -> (→"启动时间":timestamp)
        n169 = global read "CODMn断电保存全局变量.vi" "标样浓度"() -> (w387:dbl)
        n170 = global read "CODMn断电保存全局变量.vi" "CODMn跨度量程选择"() -> (w393:enum32{"H", "L", "AUTO"})
        n171 = global read "CODMn断电保存全局变量.vi" "标样核查量程选择"() -> (w384:enum32{"H", "L", "AUTO"})
        n172 = global read "CODMn断电保存全局变量.vi" "零点核查量程选择"() -> (w386:enum32{"H", "L", "AUTO"})
        n173 = global read "CODMn断电保存全局变量.vi" "加标回收量程选择"() -> (w379:enum32{"H", "L", "AUTO"})
        n174 = global read "COD内部交互全局.vi" "滴定数-ORP值"() -> (→"滴定数-ORP值":u16[])
        n175 = global read "CODMn断电保存全局变量.vi" "常规版/认证版"() -> (w388:enum16{"常规版-酸性", "常规版-碱性", "认证版", "浮台版"})
        n176 = global read "CODMn断电保存全局变量.vi" "自动切换量程:"() -> (w390:enum16{"L", "H", "自动切换测一次", "自动切换测两次"})
        n177 = global read "CODMn断电保存全局变量.vi" "零点核查浓度"() -> (w385:dbl)
        n178 = local write "高切低阈值:"(w392) -> ()
        n179 = global read "CODMn断电保存全局变量.vi" "跨度值"() -> (w373:dbl)
        n180 = local write "跨度液浓度"(w389) -> ()
        n181 = local write "低切高阈值:"(w391) -> ()
        n182 = global read "COD内部交互全局.vi" "ORP滴定曲线"() -> (→"ORP滴定曲线":u16[])
        n183 = local write "标样浓度"(w387) -> ()
        n184 = local write "标样核查量程选择"(w384) -> ()
        n185 = local write "水样量程选择:"(w390) -> ()
        n186 = local write "常规版/认证版"(w388) -> ()
        n187 = local write "零点核查浓度"(w385) -> ()
        n188 = local write "零点核查量程选择"(w386) -> ()
        n189 = local write "加标回收量程："(w379) -> ()
        n190 = local write "跨度量程选择"(w393) -> ()
        n191 = local write "跨度值"(w373) -> ()
        n192 = global read "CODMn断电保存全局变量.vi" "远程校准量程"() -> (w374:enum16{"低量程", "高量程"})
        n193 = global read "CODMn断电保存全局变量.vi" "远程标样校准"() -> (w375:enum16{"标液1", "标液2", "标液3", "标液4"})
        n194 = global read "COD内部交互全局.vi" "温度波形时间"() -> (→"温度波形时间":timestamp)
        n195 = global read "COD内部交互全局.vi" "时间温度曲线"() -> (→"时间温度曲线":u16[])
        n196 = global read "COD内部交互全局.vi" "时间-温度"() -> (→"时间-温度":u16[])
        n197 = local write "远程标样校准"(w375) -> ()
        n198 = local write "远程校准量程"(w374) -> ()
      }
    }
    n199 = flat-sequence {
      frame #0 {
        # "保存参数赋值"
        n200 = Multiply(x="温度", y=10.0) -> (x*y=w197:dbl)
        n201 = Multiply(x="标准液浓度", y=100.0) -> (x*y=w194:dbl)
        n202 = Build Array(w197, "恒温时间", w194, "氢氧化钠：", "当前量程：", "水样：", "蒸馏水：", "标液：", "零点核查样：", "加标回收样：", "高锰酸钾", "草酸钠", "硫酸", "零点泵计量数 2", "标度泵计量数 2", "高量程稀释倍数:", "低量程稀释倍数:", "CODMn零点核查选择") -> (w191:dbl[])
        n203 = local write "保存参数"(w191) -> ()
      }
    }
    n204 = flat-sequence {
      frame #0 {
        # "显示量程说明"
        n205 = global read "COD内部交互全局.vi" "通讯状态"() -> (→"通讯状态":bool)
        n206 = global read "CODMn断电保存全局变量.vi" "MB通信方式选择"() -> (w397:enum16{"串口", "TCP"})
        n207 = local read "低量程稀释倍数:"() -> (w410:i8)
        n208 = local read "高量程稀释倍数:"() -> (w400:i8)
        n209 = case shown="\"TCP\"" w397 {
          tunnel: [w413 w414] -> w401
          frame "串口", Default {
            n210 = global read "CODMn断电保存全局变量.vi" "VISA resource name"() -> (w413:refnum<visa-resource-name>)
          }
          frame "TCP" {
            n211 = global read "CODMn断电保存全局变量.vi" "IP"() -> (w414:string)
          }
        }
        "COM" <- w401
        n212 = Multiply(x=w410, y=i8 8) -> (x*y=w402:i8)
        n213 = Multiply(x=w400, y=i8 8) -> (x*y=w394:i8)
        n214 = Number To Decimal String(number=w402) -> (decimal integer string=w407:string)  [unwired: 1 in]
        n215 = Number To Decimal String(number=w394) -> (decimal integer string=w405:string)  [unwired: 1 in]
        n216 = global read "CODMn断电保存全局变量.vi" "CODMn仪器参数"() -> (w396:T12)
        n217 = Concatenate Strings("L低量程范围:0~" ("量程解释说明"), w407, "(mg/L)\n\nH高量程范围:" ("量程解释说明"), "0" ("字符串"), "~" ("量程解释说明"), w405, "(mg/L)" ("量程解释说明")) -> (→"量程解释说明":string)
        n218 = Bundle By Name(cluster=w396, "测量量程"=w394) -> (w395:T12)
        n219 = global write "CODMn断电保存全局变量.vi" "CODMn仪器参数"(w395) -> ()
      }
    }
    n220 = flat-sequence {
      frame #0 {
        # "参数赋值（只在读取参数时候改变一次）"
        n221 = global read "COD内部交互全局.vi" "读取浮台参数显示"() -> (w224:bool)
        n222 = global read "COD内部交互全局.vi" "读取浮台参数"() -> (w223:u16[])
        n223 = global read "COD内部交互全局.vi" "读取参数显示"() -> (w225:bool)
        n224 = global read "COD内部交互全局.vi" "读取参数"() -> (w226:u16[])
        n225 = case shown="真" w224 {
          tunnel: w223 -> [_ w232]
          frame False {
          }
          frame True {
            n226 = Index Array(array=w232) -> (element #1=w231:u16, element #2=w230:u16, element #3=w229:u16, element #4=w228:u16)  [unwired: 4 in]
            n227 = global write "COD内部交互全局.vi" "读取浮台参数显示"(FALSE ("读取参数显示")) -> ()
            n228 = local write "采水泵进样时间/s:"(w231) -> ()
            n229 = local write "采水泵润洗时间/s:"(w230) -> ()
            n230 = local write "采水泵沉淀时间/s:"(w229) -> ()
            n231 = local write "采水泵排液时间/s:"(w228) -> ()
          }
        }
        n232 = case shown="真" w225 {
          tunnel: w226 -> [_ w254]
          frame False {
          }
          frame True {
            n233 = Index Array(array=w254) -> (element #1=w263:u16, element #2=w233:u16, element #3=w259:u16, element #4=w237:u16, element #5=w262:u16, element #6=w261:u16, element #7=w273:u16, element #8=w272:u16, element #9=w271:u16, element #10=w270:u16, element #11=w269:u16, element #12=w268:u16, element #13=w267:u16, element #14=w266:u16, element #15=w265:u16, element #16=w257:u16, element #17=w256:u16, element #18=w255:u16, element #19=w252:u16, element #20=w251:u16, element #21=w250:u16, element #22=w249:u16, element #23=w248:u16, element #27=w244:u16, element #28=w243:u16, element #29=w242:u16, element #30=w241:u16, element #31=w240:u16)  [unwired: 31 in, 3 out]
            n234 = global write "COD内部交互全局.vi" "读取参数显示"(FALSE ("读取参数显示")) -> ()
            n235 = local write "水样："(w261) -> ()
            n236 = local write "标液："(w272) -> ()
            n237 = local write "硫酸"(w267) -> ()
            n238 = global read "CODMn断电保存全局变量.vi" "CODMn仪器参数"() -> (w236:T12)
            n239 = local write "零点核查样："(w271) -> ()
            n240 = local write "加标回收样："(w270) -> ()
            n241 = local write "当前量程："(w262) -> ()
            n242 = local write "蒸馏水："(w273) -> ()
            n243 = local write "恒温时间"(w233) -> ()
            n244 = local write "高锰酸钾"(w269) -> ()
            n245 = local write "草酸钠"(w268) -> ()
            n246 = local write "零点泵计量数 2"(w266) -> ()
            n247 = local write "标度泵计量数 2"(w265) -> ()
            n248 = local write "高量程稀释倍数:"(w257) -> ()
            n249 = local write "低量程稀释倍数:"(w256) -> ()
            n250 = local write "CODMn零点核查选择"(w255) -> ()
            n251 = Build Array(w252, w251, w250, w249, w248) -> (w247:u16[])
            n252 = Build Array(w244, w243, w242, w241, w240) -> (w239:u16[])
            n253 = Divide(x=w263, y=u16 10) -> (x/y=w234:dbl)
            n254 = Divide(x=w259, y=u16 100) -> (x/y=w258:dbl)
            n255 = local write "氢氧化钠："(w237) -> ()
            n256 = local write "温度"(w234) -> ()
            n257 = local write "标准液浓度"(w258) -> ()
            n258 = call "HexToString.vi"("数组"=w239) -> ("字符串"=w238:string)  [unwired: 10 in]
            "CODMn序列号" <- w238
            "序列号" <- w238
            n259 = call "FATEK_HexToString.vi"("数组"=w247) -> ("STRING"=w246:string[])  [unwired: 10 in]
            n260 = Bundle By Name(cluster=w236, "消解温度"=w234, "消解时长"=w233) -> (w235:T12)
            n261 = Index Array(array=w246) -> (element=→"CODMn软件版本：":string)  [unwired: 1 in]
            n262 = global write "CODMn断电保存全局变量.vi" "CODMn仪器参数"(w235) -> ()
            n263 = global write "COD内部交互全局.vi" "序列号:"(w238) -> ()
          }
        }
      }
    }
    n264 = flat-sequence {
      frame #0 {
        # "权限隐藏和显示功能"
        n265 = local read "x = y?"() -> (w420:bool)
        n266 = global read "CODMn断电保存全局变量.vi" "CODMn系统周期测试?"() -> (w417:bool)
        n267 = global read "CODMn断电保存全局变量.vi" "运行周期"() -> (w418:T13)
        n268 = property on="更新程序" class="Bool (严格)"("Visible"=w420) -> ()  [unwired: 2 in, 2 out]
        n269 = property on="释放串口" class="Bool"("Visible"=w420) -> ()  [unwired: 2 in, 2 out]
        n270 = property on="打开串口" class="Bool"("Visible"=w420) -> ()  [unwired: 2 in, 2 out]
        n271 = case shown="假" w417 {
          tunnel: w418 -> [_ w441]
          tunnel: [T9."Enabled" ("禁用") w439] -> w416
          frame False {
          }
          frame True {
            n272 = Unbundle By Name(w441) -> ("运行模式"=w440:enum16{"维护模式", "常规模式", "应急模式", "质控模式"})
            n273 = case shown="\"维护模式\", 默认" w440 {
              tunnel: [T9."Enabled" ("禁用") T9."Disabled and Grayed Out" ("禁用") T9."Disabled and Grayed Out" ("禁用") T9."Disabled and Grayed Out" ("禁用")] -> w439
              frame "维护模式", Default {
              }
              frame "常规模式" {
              }
              frame "应急模式" {
              }
              frame "质控模式" {
              }
            }
          }
        }
        n274 = property on="序列号变更" class="Bool"("Visible"=w420) -> ()  [unwired: 2 in, 2 out]
        n275 = property on="常规版/认证版" class="Enum (严格)"("Visible"=w420) -> ()  [unwired: 2 in, 2 out]
        n276 = property on="CODMn零点核查选择" class="Enum (严格)"("Visible"=w420) -> ()  [unwired: 2 in, 2 out]
        n277 = property on="低量程稀释倍数:" class="DigNum (严格)"("Visible"=w420) -> ()  [unwired: 2 in, 2 out]
        n278 = property on="稀释倍数解释" class="Str"("Visible"=w420) -> ()  [unwired: 2 in, 2 out]
        n279 = property on="高量程稀释倍数:" class="DigNum (严格)"("Visible"=w420) -> ()  [unwired: 2 in, 2 out]
        n280 = control-ref of="水样："() -> (w430:refnum<vi>)
        n281 = control-ref of="蒸馏水："() -> (w429:refnum<vi>)
        n282 = control-ref of="标液："() -> (w428:refnum<vi>)
        n283 = control-ref of="零点核查样："() -> (w427:refnum<vi>)
        n284 = control-ref of="加标回收样："() -> (w426:refnum<vi>)
        n285 = local read "水样量程选择:"() -> (w434:enum16{"L", "H", "自动切换测一次", "自动切换测两次"})
        n286 = control-ref of="量程解释说明"() -> (w424:refnum<vi>)
        n287 = control-ref of="氢氧化钠："() -> (w425:refnum<vi>)
        n288 = property on="定时设置" class="定时设置 (严格)"("DisabledEnum"=w416) -> ()  [unwired: 2 in, 2 out]
        n289 = local read "常规版/认证版"() -> (w432:enum16{"常规版-酸性", "常规版-碱性", "认证版", "浮台版"})
        n290 = Not Equal To 0?(x=w434) -> (x != 0?=w433:bool)
        n291 = control-ref of="进样管"() -> (w422:refnum<vi>)
        n292 = case shown="\"认证版\"" w432 {
          tunnel: [T9."Enabled" ("禁用") T9."Enabled" ("禁用") T9."Disabled and Grayed Out" ("禁用") T9."Enabled" ("禁用")] -> _
          tunnel: [i32[] [2] ("禁用项[]") i32[] [2] ("禁用项[]") i32[] [] ("禁用项[]") i32[] [2] ("禁用项[]")] -> _
          tunnel: [w449 w454 T9."Disabled and Grayed Out" ("禁用") w465] -> _
          tunnel: [w448 FALSE FALSE TRUE] -> w431
          tunnel: [w449 w454 T9."Disabled and Grayed Out" ("禁用") w465] -> w421
          tunnel: [w448 TRUE FALSE FALSE] -> w419
          frame "常规版-酸性", Default {
            w448 = FALSE
            w449 = T9."Enabled" ("禁用")
          }
          frame "常规版-碱性" {
            w454 = T9."Enabled" ("禁用")
          }
          frame "认证版" {
            w460 = u16 1 items=["水样测试"=1, "标样核查"=2, "零点核查"=3, "跨度核查"=4, "空白测试"=5, "平行样"=6, "加标回收"=7] ("测量模式(公式)")
            n293 = global write "CODMn断电保存全局变量.vi" "测量模式(公式)"(w460) -> ()
          }
          frame "浮台版" {
            w465 = T9."Enabled" ("禁用")
          }
        }
        n294 = Build Array(w430, w429, w428, w427, w426, w424, w425, w422) -> (w423:refnum<vi>[])
        n295 = Select(t=T9."Enabled" ("禁用"), s=w433, f=T9."Disabled and Grayed Out" ("禁用")) -> (s? t:f=w435:T9)
        n296 = for {
          tunnel: w423 -> [w447] mode=indexing
          tunnel: w421 -> [w446]
          n297 = property class="Ctl"(reference=w447, "DisabledEnum"=w446) -> ()  [unwired: 1 in, 2 out]
        }
        n298 = property on="低切高阈值:" class="DigNum (严格)"("DisabledEnum"=w435) -> ()  [unwired: 2 in, 2 out]
        n299 = property on="高切低阈值:" class="DigNum (严格)"("DisabledEnum"=w435) -> ()  [unwired: 2 in, 2 out]
        n300 = property on="采水泵润洗时间/s:" class="DigNum (严格)"("Visible"=w431) -> ()  [unwired: 2 in, 2 out]
        n301 = property on="采水泵沉淀时间/s:" class="DigNum (严格)"("Visible"=w431) -> ()  [unwired: 2 in, 2 out]
        n302 = property on="采水泵排液时间/s:" class="DigNum (严格)"("Visible"=w431) -> ()  [unwired: 2 in, 2 out]
        n303 = property on="采水泵进样时间/s:" class="DigNum (严格)"("Visible"=w431) -> ()  [unwired: 2 in, 2 out]
        n304 = property on="氢氧化钠：" class="DigNum (严格)"("Visible"=w419) -> ()  [unwired: 2 in, 2 out]
        n305 = property on="氢氧化钠" class="DigNum (严格)"("Visible"=w419) -> ()  [unwired: 2 in, 2 out]
        n306 = property on="公式切换阈值滴定数(0-9999)" class="DigNum (严格)"("Visible"=TRUE) -> ()  [unwired: 2 in, 2 out]
      }
    }
    n307 = flat-sequence {
      frame #0 {
        # "公式读取显示（只在读取公式的时候改变一次）"
        n308 = global read "COD内部交互全局.vi" "读取公式显示"() -> (w274:bool)
        n309 = case shown="真" w274 {
          frame False {
          }
          frame True {
            n310 = global write "COD内部交互全局.vi" "读取公式显示"(FALSE ("读取参数显示")) -> ()
            n311 = global read "COD内部交互全局.vi" "读取公式"() -> (w295:u16[])
            n312 = Array Subset(array=w295, index=10 ("索引"), length=84 ("长度")) -> (w283:u16[])
            n313 = Index Array(array=w283, index #1=24 ("索引")) -> (element #1=w281:u16, element #2=w280:u16)  [unwired: 1 in]
            n314 = call "浮点CDAB转换COD.vi"("数组"=w283) -> ("数组 2"=w292:sgl[])  [unwired: 10 in]
            n315 = Array To Cluster(array=w292) -> (cluster=w294:T14)
            n316 = local read "量程选择"() -> (w285:enum16{"低量程", "高量程"})
            n317 = case shown="\"高量程\"" w285 {
              tunnel: w294 -> [w303 w311]
              tunnel: [w302 w310] -> w288
              tunnel: [w301 w309] -> w287
              tunnel: [w300 w308] -> w286
              tunnel: w281 -> [w299 _]
              tunnel: w280 -> [_ w307]
              tunnel: [w298 w306] -> w277
              tunnel: [w297 w304] -> w276
              tunnel: [w296 w305] -> w275
              frame "低量程", Default {
                n318 = local write "公式切换阈值滴定数(0-9999)"(w299) -> ()
                n319 = Unbundle By Name(w303) -> ("数组 2[0]"=w302:sgl, "数组 2[1]"=w301:sgl, "数组 2[2]"=w300:sgl, "数组 2[3]"=w298:sgl, "数组 2[4]"=w297:sgl, "数组 2[5]"=w296:sgl)
              }
              frame "高量程" {
                n320 = local write "公式切换阈值滴定数(0-9999)"(w307) -> ()
                n321 = Unbundle By Name(w311) -> ("数组 2[6]"=w310:sgl, "数组 2[7]"=w309:sgl, "数组 2[8]"=w308:sgl, "数组 2[9]"=w306:sgl, "数组 2[10]"=w304:sgl, "数组 2[11]"=w305:sgl)
              }
            }
            n322 = Bundle By Name(cluster=cluster{"X":dbl, "b":dbl, "X^2":dbl} {"X"=0.0, "b"=0.0, "X^2"=0.0} ("方程系数"), "X"=w288, "b"=w287, "X^2"=w286) -> (w293:cluster{"X":dbl, "b":dbl, "X^2":dbl})
            n323 = Bundle By Name(cluster=cluster{"X":dbl, "b":dbl, "X^2":dbl} {"X"=0.0, "b"=0.0, "X^2"=0.0} ("方程系数"), "X"=w277, "b"=w276, "X^2"=w275) -> (w278:cluster{"X":dbl, "b":dbl, "X^2":dbl})
            n324 = local write "方程系数 2"(w278) -> ()
            n325 = local write "方程系数"(w293) -> ()
          }
        }
      }
    }
    n326 = Wait (ms)(milliseconds to wait=u32 1000 ("等待时间（毫秒）")) -> ()  [unwired: 1 out]
  }
  n327 = while {
    stop <- FALSE stop-if-true
    w503 = T15 0 items=["最小二乘", "最小绝对残差", "Bisquare"] ("method")
    # "计算线性、多项式公式、远程校准"
    n328 = local read "浓度1"() -> (w485:dbl)
    n329 = local read "浓度2"() -> (w504:dbl)
    n330 = local read "浓度3"() -> (w505:dbl)
    n331 = local read "浓度4"() -> (w499:dbl)
    n332 = local read "浓度5"() -> (w498:dbl)
    n333 = Build Array("泵滴定数1", "泵滴定数2", "泵滴定数3", "泵滴定数4", "泵滴定数5") -> (w469:dbl[])
    n334 = Build Array(w485, w504, w505, w499, w498) -> (w482:dbl[])
    n335 = Build Array("启用1", "启用2", "启用3", "启用4", "启用5") -> (w470:bool[])
    n336 = call "将启用的浓度作为新的浓度数组.vi"("启用布尔数组"=w470, "输入浓度数组"=w482) -> ("启用的浓度数组"=w484:dbl[])  [unwired: 13 in]
    n337 = global read "CODMN外部API.vi" "远程反控校准CODMn"() -> (w483:bool)
    n338 = call "CODMn线性公式.vi"("标液浓度"=w482, "监测浓度"=w469, "启用"=w470, "method"=w503, "模型"="模型", "精度"=6) -> ("Polynomial Coefficients 2"=w473:dbl[], "拟合方程"=w491:string, "r^2"=w472:dbl, "拟合方程 2"=w478:string, "r^2 2"=→"r^2 2":dbl, "XY图"=→"XY图":cluster{"X Values":dbl[], "Y Values":dbl[]}[], "Polynomial Coefficients"=w500:dbl[])  [unwired: 7 in]
    "拟合公式" <- w491
    "r^2" <- w472
    "拟合公式 2" <- w478
    n339 = global write "COD内部交互全局.vi" "启用的浓度数组"(w484) -> ()
    n340 = feedback #3(w478) -> (w479:string)
    n341 = feedback-in #3(w478) -> ()
    n342 = feedback #4(w491) -> (w492:string)
    n343 = feedback-in #4(w491) -> ()
    n344 = Not Equal?(x=w478, y=w479) -> (x != y?=w476:bool)
    n345 = call <vilib>:"Boolean Crossing PtByPt.vi"("direction"=enum16{"either", "false-true", "true-false"}."false-true", "input"=w483) -> ("crossing"=w481:bool)  [unwired: 1 in]
    n346 = Not Equal?(x=w491, y=w492) -> (x != y?=w477:bool)
    n347 = Or(x=w477, y=w476) -> (x .or. y?=w475:bool)
    n348 = case shown="真" w475 {
      tunnel: w500 -> [_ w524]
      tunnel: w473 -> [_ w520]
      tunnel: w472 -> [_ w516]
      tunnel: "模型" -> [_ w514]
      tunnel: w470 -> [_ w513]
      tunnel: w469 -> [_ w512]
      frame False {
      }
      frame True {
        # "当公式发生改变时赋值到右侧公式"
        n349 = case shown="\"折线\"" w514 {
          tunnel: [9999.0 ("泵滴定数5") 9999.0 ("泵滴定数5") w531] -> w515
          tunnel: w512 -> [_ _ w530]
          tunnel: w513 -> [_ _ w529]
          frame "线性", Default {
          }
          frame "多项式" {
          }
          frame "折线" {
            n350 = for {
              tunnel: w530 -> [w538] mode=indexing
              tunnel: w529 -> [w539] mode=indexing
              shift-right: [w537] -> w534
              shift-left: dbl[] [] -> [w536]
              n351 = case shown="假" w539 {
                tunnel: w538 -> [_ w543]
                tunnel: w536 -> [w540 w542]
                tunnel: [w540 w541] -> w537
                frame False {
                }
                frame True {
                  n352 = Build Array (concatenate)(w542, w543) -> (w541:dbl[])
                }
              }
            }
            n353 = Sort 1D Array(array=w534) -> (sorted array=w533:dbl[])
            n354 = Index Array(array=w533, index=1 ("索引")) -> (element=w531:dbl)
          }
        }
        n355 = Rotate 1D Array(1:w524, 2:-1 ("n")) -> (0:w525:dbl[])
        n356 = Rotate 1D Array(1:w520, 2:-1 ("n")) -> (0:w522:dbl[])
        n357 = global read "CODMn断电保存全局变量.vi" "CODMn仪器参数"() -> (w518:T12)
        n358 = Array To Cluster(array=w525) -> (cluster=w523:cluster{"[0]":dbl, "[1]":dbl, "[2]":dbl})
        n359 = Array To Cluster(array=w522) -> (cluster=w519:cluster{"[0]":dbl, "[1]":dbl, "[2]":dbl})
        n360 = Bundle By Name(cluster=w518, "线性相关系数"=w516) -> (w517:T12)
        n361 = global write "CODMn断电保存全局变量.vi" "CODMn仪器参数"(w517) -> ()
        n362 = local write "公式切换阈值滴定数(0-9999)"(w515) -> ()
        n363 = local write "方程系数"(w523) -> ()
        n364 = local write "方程系数 2"(w519) -> ()
      }
    }
    n365 = case shown="真" w481 {
      tunnel: w482 -> [_ _]
      frame False {
      }
      frame True {
        n366 = global read "CODMn断电保存全局变量.vi" "远程标样校准"() -> (w510:enum16{"标液1", "标液2", "标液3", "标液4"})
        n367 = local read "远程校准量程"() -> (w508:enum16{"低量程", "高量程"})
        n368 = Increment(x=w510) -> (x+1=w509:enum16{"标液1", "标液2", "标液3", "标液4"})
        n369 = property on="量程选择" class="Enum (严格)"("Val(Sgnl)"=w508) -> ()  [unwired: 2 in, 2 out]
        n370 = Increment(x=w509) -> (x+1=w511:enum16{"标液1", "标液2", "标液3", "标液4"})
        n371 = global write "COD内部交互全局.vi" "当前校准"(w511) -> ()
      }
    }
    n372 = Wait (ms)(milliseconds to wait=u32 1000 ("等待时间（毫秒）")) -> ()  [unwired: 1 out]
  }
  n373 = while {
    tunnel: w15 -> [w553]
    tunnel: w14 -> [w552]
    tunnel: w5 -> [_]
    stop <- FALSE stop-if-true
    # "主循环界面显示"
    n374 = flat-sequence {
      frame #0 {
        # "A，B，K"
        # "CODMn读取状态"
        n375 = global read "COD内部交互全局.vi" "ORP、时间"() -> (w688:u16[])
        n376 = To Word Integer(number=w688) -> (16bit integer=w709:i16[])
        n377 = Split 1D Array(array=w709, index=3 ("索引")) -> (first subarray=w690:i16[], second subarray=w708:i16[])
        n378 = Index Array(array=w690) -> (element #1=w694:i16, element #2=w693:i16, element #3=w692:i16)  [unwired: 3 in]
        n379 = Index Array(array=w708) -> (element #1=w703:i16, element #2=w707:i16, element #3=w706:i16, element #4=w705:i16)  [unwired: 4 in]
        n380 = To Single Precision Float(number=w705) -> (single precision float=w696:sgl)
        n381 = Build Array(w694, w693, w692) -> (w691:i16[])
        n382 = To Single Precision Float(number=w703) -> (single precision float=w702:sgl)
        n383 = To Single Precision Float(number=w707) -> (single precision float=w701:sgl)
        n384 = To Single Precision Float(number=w706) -> (single precision float=w697:sgl)
        n385 = call "HexToDate.vi"("数组"=w691) -> ("DATE"=w695:timestamp[])  [unwired: 10 in]
        n386 = Number To Decimal String(number=w701) -> (decimal integer string=→"ORP-A":string)  [unwired: 1 in]
        n387 = Number To Decimal String(number=w697) -> (decimal integer string=→"ORP-B":string)  [unwired: 1 in]
        n388 = Number To Decimal String(number=w696) -> (decimal integer string=→"ORP-K":string)  [unwired: 1 in]
        n389 = Divide(x=w702, y=sgl 100.0) -> (x/y=→"COD浓度（mg/L)":sgl)
        n390 = Index Array(array=w695) -> (element=w689:timestamp)  [unwired: 1 in]
        n391 = Format Date/Time String(seconds (now)=w689) -> (date/time string=→"数据时间":string)  [unwired: 2 in]
      }
    }
    n392 = flat-sequence {
      frame #0 {
        # "测量状态显示"
        n393 = global read "COD内部交互全局.vi" "测量状态"() -> (w602:u16[])
        n394 = To Word Integer(number=w602) -> (16bit integer=w612:i16[])
        n395 = Index Array(array=w612, index #1=0 ("索引"), index #4=3 ("索引"), index #14=13 ("索引"), index #15=14 ("索引"), index #21=20 ("索引"), index #32=31 ("索引")) -> (element #1=w616:i16, element #2=w615:i16, element #3=w614:i16, element #4=w598:i16, element #5=→"模式（受控）":i16, element #6=→"进样管":i16, element #7=→"高锰酸钾":i16, element #8=→"草酸钠":i16, element #9=→"硫酸":i16, element #10=w611:i16, element #11=w631:i16, element #12=w607:i16, element #13=→"报警数字":i16, element #14=w637:i16, element #15=w622:i16, element #16=→"多列列表框":i16, element #20=→"氢氧化钠":i16, element #21=w595:i16, element #33=→"分":i16, element #34=→"秒":i16)  [unwired: 28 in, 14 out]
        "CODMn工作状态" <- w598
        n396 = global write "COD内部交互全局.vi" "基本量程实时读取"(w595) -> ()
        n397 = Build Array(w616, w615, w614) -> (w617:i16[])
        n398 = To Single Precision Float(number=w611) -> (single precision float=→"实时ORP":sgl)
        n399 = Number To Decimal String(number=w595) -> (decimal integer string=→"基本量程(显示)":string)  [unwired: 1 in]
        n400 = Equal?(x=w607, y=u16 1) -> (x = y?=→"排液标记":bool)
        n401 = Equal?(x=w607, y=u16 2) -> (x = y?=→"断电排液标记":bool)
        n402 = Divide(x=w631, y=u16 10) -> (x/y=→"温度℃":dbl)
        n403 = Divide(x=w637, y=u16 1000) -> (x/y=→"零点滴定值":dbl)
        n404 = Divide(x=w622, y=u16 1000) -> (x/y=→"标度滴定值":dbl)
        n405 = Equal?(x=w598, y=T3."水样测试" ("CODMn工作状态")) -> (x = y?=w596:bool)
        n406 = call "HexToDate.vi"("数组"=w617) -> ("DATE"=w613:timestamp[])  [unwired: 10 in]
        n407 = case shown="真" w596 {
          tunnel: w595 -> [_ w640]
          frame False {
          }
          frame True {
            n408 = global write "CODMn断电保存全局变量.vi" "水样测试量程"(w640) -> ()
          }
        }
        n409 = Index Array(array=w613) -> (element=→"仪器时间":timestamp)  [unwired: 1 in]
      }
    }
    n410 = flat-sequence {
      frame #0 {
        # "报警状态显示"
        n411 = global read "COD内部交互全局.vi" "报警点位"() -> (w655:bool[])
        n412 = Index Array(array=w655, index #1=0 ("索引")) -> (element #1=w652:bool, element #2=w651:bool, element #3=w650:bool, element #4=w649:bool, element #5=w648:bool, element #6=w647:bool, element #7=w646:bool, element #8=w645:bool, element #9=w644:bool, element #11=w643:bool, element #13=w642:bool, element #14=w641:bool)  [unwired: 13 in, 2 out]
        "ORP故障" <- w652
        "温控器故障" <- w651
        "加热故障" <- w644
        "高锰酸钾报警" <- w646
        "草酸钠报警" <- w645
        "测量错误" <- w650
        "校零错误" <- w649
        "校标错误" <- w648
        "进水样超量程" <- w647
        "排液故障" <- w643
        "60分钟超时报警" <- w642
        "进样无液体告警" <- w641
        n413 = Compound Arithmetic op=OR ("复合运算")(w652, w651, w644, w646, w645, w650, w648, w649, w647, w643, w642) -> (→"故障标记":bool)
        n414 = Bundle By Name(cluster=T16 {"ORP故障"=FALSE, "温控器故障"=FALSE, "加热故障"=FALSE, "高锰酸钾报警"=FALSE, "草酸钠报警"=FALSE, "测量错误"=FALSE, "校零错误"=FALSE, "校标错误"=FALSE, " 进水样超量程"=FALSE, "排液阀故障"=FALSE, "60分钟超时报警"=FALSE, "进样无液体报警"=FALSE} ("报警簇"), "ORP故障"=w652, "温控器故障"=w651, "加热故障"=w644, "高锰酸钾报警"=w646, "草酸钠报警"=w645, "测量错误"=w650, "校零错误"=w649, "校标错误"=w648, "进水样超量程"=w647, "排液阀故障"=w643, "60分钟超时报警"=w642, "进样无液体报警"=w641) -> (w653:T16)
        n415 = global write "COD内部交互全局.vi" "报警簇"(w653) -> ()
      }
    }
    n416 = flat-sequence {
      frame #0 {
        # "CODMn读取状态"
        n417 = global read "COD内部交互全局.vi" "温度"() -> (w685:bool[])
        n418 = global read "COD内部交互全局.vi" "M输出点"() -> (w684:bool[])
        n419 = Index Array(array=w685) -> (element=→"加热":bool)  [unwired: 1 in]
        n420 = Index Array(array=w684) -> (element #1=→"搅拌":bool, element #4=→"进水样":bool, element #5=→"进蒸馏水":bool, element #6=→"进标液":bool, element #7=→"进零点核查样":bool, element #8=→"进加标回收样":bool, element #9=→"进高锰酸钾":bool, element #10=→"进草酸钠":bool, element #11=→"进硫酸":bool)  [unwired: 11 in, 2 out]
      }
    }
    n421 = flat-sequence {
      frame #0 {
        # "工作状态显示"
        n422 = local read "CODMn工作状态"() -> (w563:T3)
        n423 = case shown="\"标样校准\"" w563 {
          tunnel: [_ u16 0 ("y") u16 1 ("y") u16 2 ("y") u16 3 ("y") u16 4 ("y") u16 6 ("y") _ u16 7 ("y") u16 8 ("y") u16 5 ("y")] -> w562
          frame "空闲", Default {
          }
          frame "水样测试" {
          }
          frame "标样核查" {
          }
          frame "零点核查" {
          }
          frame "跨度核查" {
          }
          frame "空白测试" {
          }
          frame "平行样测试" {
          }
          frame "质控样" {
          }
          frame "空白校准" {
          }
          frame "标样校准" {
          }
          frame "加标回收" {
          }
        }
        n424 = Equal?(x=w563, y=u16 8) -> (x = y?=→"校零标记":bool)
        n425 = Equal?(x=w563, y=u16 4) -> (x = y?=→"跨度核查标记":bool)
        n426 = Equal?(x=w563, y=u16 0) -> (x = y?=→"待机":bool)
        n427 = Equal?(x=w563, y=u16 3) -> (x = y?=→"零点核查标记":bool)
        n428 = Equal?(x=w563, y=u16 7) -> (x = y?=→"质控样测量":bool)
        n429 = Equal?(x=w563, y=u16 1) -> (x = y?=→"水样测量":bool)
        n430 = Equal?(x=w563, y=u16 2) -> (x = y?=→"标样核查标记":bool)
        n431 = Equal?(x=w563, y=u16 6) -> (x = y?=→"平行样测量":bool)
        n432 = Equal?(x=w563, y=u16 9) -> (x = y?=→"校标标记":bool)
        n433 = Equal?(x=w563, y=u16 5) -> (x = y?=→"空白测试标记":bool)
        n434 = Equal?(x=w563, y=u16 10) -> (x = y?=→"加标回收测量":bool)
        n435 = global write "COD内部交互全局.vi" "测量模式数字"(w562) -> ()
      }
    }
    n436 = Get Date/Time In Seconds() -> (seconds since 1Jan1904=→"系统时间":timestamp)
    n437 = First Call?() -> (First Call?: T/F=w551:bool)
    n438 = Wait (ms)(milliseconds to wait=u32 1000 ("等待时间（毫秒）")) -> ()  [unwired: 1 out]
    n439 = case shown="真" w551 {
      tunnel: w553 -> [w659 w670]
      tunnel: w552 -> [w658 w669]
      tunnel: [w659 w661] -> w549
      tunnel: [w658 w660] -> w548
      frame False {
      }
      frame True {
        n440 = Bundle By Name(cluster=cluster{"命令":string} {"命令"=""} ("元素"), "命令"="CODMn读取参数" ("名称（未命名）")) -> (w673:cluster{"命令":string})
        n441 = Enqueue Element(queue=w670, element=w673, timeout in ms (-1)=1000 ("超时毫秒(-1)"), error in (no error)=w669) -> (queue out=w663:refnum<queue>, error out=w662:errorcluster)  [unwired: 1 out]
        n442 = Bundle By Name(cluster=cluster{"命令":string} {"命令"=""} ("元素"), "命令"="CODMn读取公式" ("名称（未命名）")) -> (w664:cluster{"命令":string})
        n443 = Enqueue Element(queue=w663, element=w664, timeout in ms (-1)=1000 ("超时毫秒(-1)"), error in (no error)=w662) -> (queue out=w661:refnum<queue>, error out=w660:errorcluster)  [unwired: 1 out]
      }
    }
    n444 = Get Queue Status(queue=w549, error in (no error)=w548) -> (queue out=w545:refnum<queue>, error out=w544:errorcluster, # elements in queue=w547:i32)  [unwired: 1 in, 5 out]
    n445 = Equal To 0?(x=w547) -> (x = 0?=w546:bool)
    n446 = case shown="真" w546 {
      tunnel: w545 -> [_ w557]
      tunnel: w544 -> [_ w556]
      frame False {
      }
      frame True {
        n447 = Bundle By Name(cluster=cluster{"命令":string} {"命令"=""} ("元素"), "命令"="CODMn读取" ("名称（未命名）")) -> (w559:cluster{"命令":string})
        n448 = Enqueue Element(queue=w557, element=w559, timeout in ms (-1)=1000 ("超时毫秒(-1)"), error in (no error)=w556) -> ()  [unwired: 3 out]
      }
    }
  }
  n449 = while {
    tunnel: w15 -> [w712]
    tunnel: w14 -> [w711]
    stop <- FALSE stop-if-true
    # "主线事件"
    n450 = event shown="[21] \"浓度1\", \"浓度2\", \"浓度3\", \"泵滴定数1\", \"泵滴定数2\", \"泵滴定数3\", \"启用1\", \"启用2\", \"启用3\", \"浓度4\", \"浓度5\", \"泵滴定数4\", \"泵滴定数5\", \"启用4\", \"启用5\", \"标液校准时间1\", \"标液校准时间2\", \"标液校准时间3\", \"标液校准时间4\", \"零点校准时间\": 值改变" {
      selector: _ -> [_ _ _ _ _ _ _ _ _ _ _ _ _ _ _ _ _ _ _ _ _ _ _ _ _ _ _ _ _ _ _]
      dyn-events: _ -> [_ _ _ _ _ _ _ _ _ _ _ _ _ _ _ _ _ _ _ _ _ _ _ _ _ _ _ _ _ _ _]
      timeout: _ -> [_ _ _ _ _ _ _ _ _ _ _ _ _ _ _ _ _ _ _ _ _ _ _ _ _ _ _ _ _ _ _]
      tunnel: w712 -> [_ _ _ _ _ w803 _ _ w836 w974 w1100 _ _ _ _ _ _ _ w1313 _ _ _ w1576 _ _ _ w1640 w1647 w1669 w1712 _]
      tunnel: w711 -> [_ _ _ _ _ w802 _ _ w835 w973 w1099 _ _ _ _ _ _ _ w1310 _ _ _ w1575 _ _ _ w1639 w1646 w1668 w1711 _]
      event "单步启动": Value Change {
        n451 = event-data() -> ()  [unwired: 1 in, 6 out]
        n452 = call "CODMn手动控制框.vi"() -> ()  [unwired: 12 in]
      }
      event "启动": Mouse Down {
        n453 = event-data() -> ()  [unwired: 1 in, 8 out]
        n454 = global read "COD内部交互全局.vi" "基本量程实时读取"() -> (w716:enum16{"L", "H", "AUTO"})
        n455 = call "启动测量模式选择对话框.vi"("量程选择"=w716) -> ("标样浓度输出"=w714:dbl, "量程选择输出"=w715:enum16{"L", "H", "AUTO"}, "启动选择输出"=w720:u16)  [unwired: 8 in]
        n456 = Not Equal?(x=w720, y=u16 8) -> (x != y?=w717:bool)
        n457 = Not Equal?(x=w720, y=u16 7) -> (x != y?=w718:bool)
        n458 = And(x=w718, y=w717) -> (x .and. y?=w722:bool)
        n459 = case shown="真" w722 {
          tunnel: w720 -> [_ w737]
          tunnel: w715 -> [_ w728]
          tunnel: w714 -> [_ w727]
          frame False {
            n460 = One Button Dialog(message="请到校准配置里面进行校准操作！" ("消息")) -> ()  [unwired: 1 in, 1 out]
          }
          frame True {
            n461 = Not Equal?(x=w737, y=u16 9) -> (x != y?=w732:bool)
            n462 = case shown="\"H\"" w728 {
              tunnel: [w738 w742 errorcluster {"status"=FALSE, "code"=0, "source"=""} ("error out")] -> w726
              frame "L", Default {
                n463 = call "CODMnMB_api.vi"("STEP"=enum16{"open", "read", "write", "close"}."write", "values"=u16[] [0], "starting address"=u16 4276) -> ("error out"=w738:errorcluster)  [unwired: 6 in, 2 out]
              }
              frame "H" {
                n464 = call "CODMnMB_api.vi"("STEP"=enum16{"open", "read", "write", "close"}."write", "values"=u16[] [1], "starting address"=u16 4276) -> ("error out"=w742:errorcluster)  [unwired: 6 in, 2 out]
              }
              frame "AUTO" {
              }
            }
            n465 = global write "CODMN外部API.vi" "手动启动CODMn"(w732) -> ()
            n466 = call "单步测试一键复位.vi"("Error in"=w726) -> ("error out"=w725:errorcluster)  [unwired: 10 in]
            n467 = call <vilib>:"Clear Errors.vi"("error in (no error)"=w725) -> ("error out"=w724:errorcluster)  [unwired: 5 in, 1 out]
            n468 = case shown="0" w737 {
              tunnel: [u16 4608 ("address") u16 4608 ("address") u16 4608 ("address") u16 4608 ("address") u16 4608 ("address") u16 4608 ("address") u16 4608 ("address") u16 4608 ("address") u16 4608 ("address") u16 4608 ("address")] -> w730
              tunnel: [u16 1 ("address") u16 2 ("address") u16 3 ("address") u16 4 ("address") u16 5 ("address") u16 7 ("address") u16 6 ("address") u16 8 ("address") u16 9 ("address") u16 0 ("address")] -> w734
              tunnel: w727 -> [_ w750 _ _ _ _ _ _ _ _]
              frame 0 {
              }
              frame 1 {
                n469 = property on="标样浓度" class="DigNum (严格)"("Val(Sgnl)"=w750) -> ()  [unwired: 2 in, 2 out]
              }
              frame 2 {
              }
              frame 3 {
              }
              frame 4 {
              }
              frame 5 {
              }
              frame 6 {
              }
              frame 7 {
              }
              frame 8 {
              }
              frame 9, Default {
              }
            }
            n470 = Insert Into Array(array=u16[] [] ("values"), index=0 ("索引"), new element=w734) -> (w729:u16[])
            n471 = call "CODMnMB_api.vi"("STEP"=enum16{"open", "read", "write", "close"}."write", "Error in"=w724, "values"=w729, "starting address"=w730) -> ()  [unwired: 5 in, 3 out]
          }
        }
      }
      event "停止": Value Change {
        n472 = event-data() -> ()  [unwired: 1 in, 6 out]
        n473 = Two Button Dialog(message="确认是否停止？" ("消息"), 1:"否" ("F按钮名称（“取消”）"), 2:"是" ("T按钮名称（“确定”）")) -> (T button?=w770:bool)
        n474 = case shown="真" w770 {
          frame False {
          }
          frame True {
            n475 = Obtain Notifier(name (unnamed)="CODMn" ("名称（未命名）"), notification data type=FALSE) -> (notifier out=w776:refnum<notifier>, error out=w774:errorcluster)  [unwired: 2 in, 1 out]
            n476 = Send Notification(notification=TRUE ("通知"), notifier=w776, error in (no error)=w774) -> (notifier out=w773:refnum<notifier>, error out=w772:errorcluster)
            n477 = Release Notifier(notifier=w773, error in (no error)=w772) -> ()  [unwired: 1 in, 3 out]
            n478 = call "CODMnMB_api.vi"("STEP"=enum16{"open", "read", "write", "close"}."write", "values"=u16[] [11], "starting address"=u16 4608) -> ()  [unwired: 6 in, 3 out]
          }
        }
      }
      event "手动控制": Value Change {
        n479 = event-data() -> ()  [unwired: 1 in, 6 out]
        n480 = call "数字密码键盘.vi"() -> ("NewNumber"=w782:sgl)  [unwired: 1 in]
        n481 = Equal?(x=w782, y=8.0) -> (x = y?=w783:bool)
        n482 = case shown="假" w783 {
          frame False {
            n483 = call "窗口弹出对话框(子VI).vi"("消息"="密码错误") -> ()  [unwired: 10 in, 1 out]
          }
          frame True {
          }
        }
      }
      event "锁定按钮": Mouse Down {
        n484 = event-data() -> ("CtlRef"=w788:refnum<vi>)  [unwired: 1 in, 7 out]
        n485 = property class="Bool (严格)"(reference=w788) -> ("Value"=w787:bool)  [unwired: 1 in, 2 out]
        n486 = case shown="真" w787 {
          selector: w787 -> [w789 _]
          tunnel: [w789 w793] -> w786
          frame False {
          }
          frame True {
            n487 = call "数字密码键盘.vi"() -> ("NewNumber"=w790:sgl)  [unwired: 1 in]
            n488 = Equal?(x=w790, y=23506.0) -> (x = y?=w794:bool)
            n489 = Equal?(x=w790, y=8.0) -> (x = y?=w791:bool)
            n490 = Or(x=w794, y=w791) -> (x .or. y?=w793:bool)
            n491 = case shown="假" w793 {
              selector: w793 -> [w797 _]
              frame False {
                n492 = local write "锁定按钮"(w797) -> ()
                n493 = One Button Dialog(message="密码错误!" ("消息")) -> ()  [unwired: 1 in, 1 out]
              }
              frame True {
                n494 = One Button Dialog(message="解锁成功!" ("消息")) -> ()  [unwired: 1 in, 1 out]
              }
            }
          }
        }
        "x = y?" <- w786
      }
      event "参数配置": Value Change {
        (unwired) u16 20 ("number of holding registers")
        (unwired) u16 4272 ("starting address")
        n495 = event-data() -> ()  [unwired: 1 in, 6 out]
        n496 = global read "CODMN外部API.vi" "ping"() -> (w801:bool)
        n497 = property on="窗格" class="Pane"("Origin"=T4 {"Horizontal"=0, "Vertical"=650} ("原点")) -> ()  [unwired: 2 in, 2 out]
        n498 = case shown="假" w801 {
          tunnel: [w813 w816] -> w800
          frame False {
            n499 = global read "COD内部交互全局.vi" "配置文件ini"() -> (w815:string)
            n500 = call <vilib>:"Application Directory.vi"() -> ("Application Directory"=w814:path)
            n501 = Build Path(base path=w814, name or relative path=w815) -> (appended path=w813:path)
          }
          frame True {
            n502 = global read "CODMN外部API.vi" "配置文件 path"() -> (w816:path)
          }
        }
        n503 = Bundle By Name(cluster=cluster{"命令":string} {"命令"=""} ("元素"), "命令"="CODMn读取参数" ("名称（未命名）")) -> (w804:cluster{"命令":string})
        n504 = call <vilib>:"Open Config Data.vi"("configuration file path"=w800) -> ("error out"=w810:errorcluster, "refnum"=w807:T6)  [unwired: 8 in, 1 out]
        n505 = Enqueue Element(queue=w803, element=w804, error in (no error)=w802) -> ()  [unwired: 1 in, 3 out]
        n506 = vi-ref "斯坦道CODMn.lvlib:CODMn断电保存全局变量.vi"() -> (w808:refnum<vi>)
        n507 = call <userlib>:"Read Panel from INI__ogtk.vi"("error in (no error)"=w810, "VI ref"=w808, "refnum"=w807) -> ("error out"=w811:errorcluster, "refnum out"=w809:T6)  [unwired: 7 in]
        n508 = call <vilib>:"Close Config Data.vi"("error in (no error)"=w811, "refnum"=w809) -> ("error out"=w799:errorcluster)  [unwired: 8 in, 1 out]
        n509 = call <vilib>:"Clear Errors.vi"("error in (no error)"=w799) -> ()  [unwired: 5 in, 2 out]
      }
      event "保存": Mouse Down {
        n510 = event-data() -> ()  [unwired: 1 in, 8 out]
        n511 = local read "通讯状态"() -> (w817:bool)
        n512 = Two Button Dialog(message="确定保存参数，保存参数将会替换原有参数！" ("消息")) -> (T button?=w819:bool)  [unwired: 2 in]
        n513 = case shown="真" w819 {
          tunnel: w817 -> [_ w820]
          frame False {
          }
          frame True {
            n514 = case shown="真" w820 {
              frame False {
                n515 = One Button Dialog(message="保存失败，当前无通讯！" ("消息")) -> ()  [unwired: 1 in, 1 out]
              }
              frame True {
                n516 = One Button Dialog(message="参数保存成功！" ("消息")) -> ()  [unwired: 1 in, 1 out]
                n517 = Build Array("采水泵进样时间/s:", "采水泵润洗时间/s:", "采水泵沉淀时间/s:", "采水泵排液时间/s:") -> (w823:i32[])
                n518 = call "CODMnMB_api.vi"("STEP"=enum16{"open", "read", "write", "close"}."write", "values"="保存参数", "starting address"=u16 4272) -> ("error out"=w829:errorcluster)  [unwired: 6 in, 2 out]
                n519 = call "CODMnMB_api.vi"("STEP"=enum16{"open", "read", "write", "close"}."write", "Error in"=w829, "values"=w823, "starting address"=u16 5596) -> ()  [unwired: 5 in, 3 out]
              }
            }
          }
        }
      }
      event "常规版/认证版": Value Change {
        n520 = event-data() -> ()  [unwired: 1 in, 6 out]
        n521 = flat-sequence {
          frame #0 {
            n522 = global write "CODMn断电保存全局变量.vi" "常规版/认证版"("常规版/认证版") -> ()
          }
          frame #1 {
            n523 = call "配置文件保存.vi"() -> ()  [unwired: 12 in]
          }
        }
      }
      event "校准配置": Value Change {
        w849 = "量程选择" ("section")
        n524 = event-data() -> ()  [unwired: 1 in, 6 out]
        n525 = global read "CODMN外部API.vi" "ping"() -> (w853:bool)
        n526 = property on="窗格" class="Pane"("Origin"=T4 {"Horizontal"=0, "Vertical"=1300} ("原点")) -> ()  [unwired: 2 in, 2 out]
        n527 = case shown="假" w853 {
          tunnel: [w931 w934] -> w852
          frame False {
            n528 = global read "COD内部交互全局.vi" "配置文件ini"() -> (w933:string)
            n529 = call <vilib>:"Application Directory.vi"() -> ("Application Directory"=w932:path)
            n530 = Build Path(base path=w932, name or relative path=w933) -> (appended path=w931:path)
          }
          frame True {
            n531 = global read "CODMN外部API.vi" "配置文件 path"() -> (w934:path)
          }
        }
        n532 = Bundle By Name(cluster=cluster{"命令":string} {"命令"=""} ("元素"), "命令"="CODMn读取公式" ("名称（未命名）")) -> (w837:cluster{"命令":string})
        n533 = Enqueue Element(queue=w836, element=w837, error in (no error)=w835) -> ()  [unwired: 1 in, 3 out]
        n534 = call <vilib>:"Open Config Data.vi"("configuration file path"=w852) -> ("error out"=w870:errorcluster, "refnum"=w871:T6)  [unwired: 8 in, 1 out]
        n535 = call-poly <vilib>:"Read Key.vi"("section"="CODMn模型选择" ("key"), "error in (no error)"=w870, "key"="线性和多项式", "refnum"=w871) -> ("error out"=w867:errorcluster, "value"=w869:i32, "refnum out"=w868:T6)  [unwired: 4 in, 1 out]
        n536 = local write "模型"(w869) -> ()
        n537 = call-poly <vilib>:"Read Key.vi"("section"="标线选择", "error in (no error)"=w867, "key"="选用水样", "refnum"=w868) -> ("error out"=w850:errorcluster, "value"=w854:i32, "refnum out"=w851:T6)  [unwired: 4 in, 1 out]
        n538 = local write "选用水样"(w854) -> ()
        n539 = case shown="0, 默认" w854 {
          tunnel: ["葡萄糖标线" ("section") "草酸钠标线" ("section")] -> w876
          frame 0, Default {
          }
          frame 1 {
          }
        }
        n540 = call-poly <vilib>:"Read Key.vi"("section"=w849, "error in (no error)"=w850, "key"=w849, "refnum"=w851) -> ("error out"=w847:errorcluster, "value"=w846:i32, "refnum out"=w848:T6)  [unwired: 4 in, 1 out]
        n541 = local write "量程选择"(w846) -> ()
        n542 = case shown="2" w846 {
          tunnel: ["低量程" "高量程" "0-2量程"] -> w875
          frame 0, Default {
          }
          frame 1 {
          }
          frame 2 {
          }
        }
        n543 = Concatenate Strings(w876, w875) -> (w874:string)
        n544 = call-poly <vilib>:"Read Key.vi"("section"=w874, "error in (no error)"=w847, "key"="浓度1", "refnum"=w848) -> ("error out"=w901:errorcluster, "value"=w899:dbl, "refnum out"=w900:T6)  [unwired: 4 in, 1 out]
        n545 = local write "浓度1"(w899) -> ()
        n546 = call-poly <vilib>:"Read Key.vi"("section"=w874, "error in (no error)"=w901, "key"="浓度2", "refnum"=w900) -> ("error out"=w915:errorcluster, "value"=w902:dbl, "refnum out"=w914:T6)  [unwired: 4 in, 1 out]
        n547 = local write "浓度2"(w902) -> ()
        n548 = call-poly <vilib>:"Read Key.vi"("section"=w874, "error in (no error)"=w915, "key"="浓度3", "refnum"=w914) -> ("error out"=w916:errorcluster, "value"=w904:dbl, "refnum out"=w913:T6)  [unwired: 4 in, 1 out]
        n549 = local write "浓度3"(w904) -> ()
        n550 = call-poly <vilib>:"Read Key.vi"("section"=w874, "error in (no error)"=w916, "key"="泵滴定数1", "refnum"=w913) -> ("error out"=w917:errorcluster, "value"=w906:dbl, "refnum out"=w912:T6)  [unwired: 4 in, 1 out]
        n551 = local write "泵滴定数1"(w906) -> ()
        n552 = call-poly <vilib>:"Read Key.vi"("section"=w874, "error in (no error)"=w917, "key"="泵滴定数2", "refnum"=w912) -> ("error out"=w911:errorcluster, "value"=w909:dbl, "refnum out"=w918:T6)  [unwired: 4 in, 1 out]
        n553 = local write "泵滴定数2"(w909) -> ()
        n554 = call-poly <vilib>:"Read Key.vi"("section"=w874, "error in (no error)"=w911, "key"="泵滴定数3", "refnum"=w918) -> ("error out"=w923:errorcluster, "value"=w922:dbl, "refnum out"=w919:T6)  [unwired: 4 in, 1 out]
        n555 = local write "泵滴定数3"(w922) -> ()
        n556 = call-poly <vilib>:"Read Key.vi"("section"=w874, "error in (no error)"=w923, "key"="浓度4", "refnum"=w919) -> ("error out"=w924:errorcluster, "value"=w860:dbl, "refnum out"=w920:T6)  [unwired: 4 in, 1 out]
        n557 = local write "浓度4"(w860) -> ()
        n558 = call-poly <vilib>:"Read Key.vi"("section"=w874, "error in (no error)"=w924, "key"="浓度5", "refnum"=w920) -> ("error out"=w865:errorcluster, "value"=w859:dbl, "refnum out"=w866:T6)  [unwired: 4 in, 1 out]
        n559 = local write "浓度5"(w859) -> ()
        n560 = call-poly <vilib>:"Read Key.vi"("section"=w874, "error in (no error)"=w865, "key"="泵滴定数4", "refnum"=w866) -> ("error out"=w925:errorcluster, "value"=w858:dbl, "refnum out"=w921:T6)  [unwired: 4 in, 1 out]
        n561 = local write "泵滴定数4"(w858) -> ()
        n562 = call-poly <vilib>:"Read Key.vi"("section"=w874, "error in (no error)"=w925, "key"="泵滴定数5", "refnum"=w921) -> ("error out"=w863:errorcluster, "value"=w857:dbl, "refnum out"=w864:T6)  [unwired: 4 in, 1 out]
        n563 = local write "泵滴定数5"(w857) -> ()
        n564 = call-poly <vilib>:"Read Key.vi"("section"=w874, "error in (no error)"=w863, "key"="当前选用的校准", "refnum"=w864) -> ("error out"=w895:errorcluster, "refnum out"=w896:T6)  [unwired: 4 in, 2 out]
        n565 = call-poly <vilib>:"Read Key.vi"("section"=w874, "error in (no error)"=w895, "key"="启用1", "refnum"=w896) -> ("error out"=w892:errorcluster, "value"=w881:bool, "refnum out"=w893:T6)  [unwired: 4 in, 1 out]
        n566 = local write "启用1"(w881) -> ()
        n567 = call-poly <vilib>:"Read Key.vi"("section"=w874, "error in (no error)"=w892, "key"="启用2", "refnum"=w893) -> ("error out"=w890:errorcluster, "value"=w880:bool, "refnum out"=w891:T6)  [unwired: 4 in, 1 out]
        n568 = local write "启用2"(w880) -> ()
        n569 = call-poly <vilib>:"Read Key.vi"("section"=w874, "error in (no error)"=w890, "key"="启用3", "refnum"=w891) -> ("error out"=w888:errorcluster, "value"=w879:bool, "refnum out"=w889:T6)  [unwired: 4 in, 1 out]
        n570 = local write "启用3"(w879) -> ()
        n571 = call-poly <vilib>:"Read Key.vi"("section"=w874, "error in (no error)"=w888, "key"="启用4", "refnum"=w889) -> ("error out"=w886:errorcluster, "value"=w856:bool, "refnum out"=w887:T6)  [unwired: 4 in, 1 out]
        n572 = local write "启用4"(w856) -> ()
        n573 = call-poly <vilib>:"Read Key.vi"("section"=w874, "error in (no error)"=w886, "key"="启用5", "refnum"=w887) -> ("error out"=w861:errorcluster, "value"=w855:bool, "refnum out"=w862:T6)  [unwired: 4 in, 1 out]
        n574 = local write "启用5"(w855) -> ()
        n575 = call <vilib>:"Close Config Data.vi"("error in (no error)"=w861, "refnum"=w862) -> ("error out"=w840:errorcluster, "file path"=w841:path)  [unwired: 8 in]
        n576 = Open/Create/Replace File(file path (use dialog)=w841, error in=w840) -> (refnum out=w843:refnum<file>, error out=w842:errorcluster)  [unwired: 4 in, 1 out]
        n577 = Flush File(refnum=w843, error in=w842) -> (refnum out=w844:refnum<file>, error out=w845:errorcluster)
        n578 = Close File(refnum=w844, error in=w845) -> ()  [unwired: 2 out]
      }
      event "选用水样": Value Change {
        (unwired) "浓度6" ("key")
        n579 = event-data() -> ()  [unwired: 1 in, 6 out]
        n580 = local read "量程选择"() -> (w1003:enum16{"低量程", "高量程"})
        n581 = property on="窗格" class="Pane"("Origin"=T4 {"Horizontal"=0, "Vertical"=1300} ("原点")) -> ()  [unwired: 2 in, 2 out]
        n582 = case shown="\"葡萄糖\", 默认" "选用水样" {
          tunnel: ["葡萄糖标线" ("section") "草酸钠标线" ("section")] -> w1005
          frame "葡萄糖", Default {
          }
          frame "草酸钠" {
          }
        }
        n583 = global read "CODMN外部API.vi" "ping"() -> (w992:bool)
        n584 = case shown="\"高量程\"" w1003 {
          tunnel: ["低量程" "高量程"] -> w1004
          frame "低量程", Default {
          }
          frame "高量程" {
          }
        }
        n585 = case shown="假" w992 {
          tunnel: [w1058 w1061] -> w991
          frame False {
            n586 = global read "COD内部交互全局.vi" "配置文件ini"() -> (w1060:string)
            n587 = call <vilib>:"Application Directory.vi"() -> ("Application Directory"=w1059:path)
            n588 = Build Path(base path=w1059, name or relative path=w1060) -> (appended path=w1058:path)
          }
          frame True {
            n589 = global read "CODMN外部API.vi" "配置文件 path"() -> (w1061:path)
          }
        }
        n590 = Concatenate Strings(w1005, w1004) -> (w958:string)
        n591 = call <vilib>:"Open Config Data.vi"("configuration file path"=w991) -> ("error out"=w987:errorcluster, "refnum"=w988:T6)  [unwired: 8 in, 1 out]
        n592 = Bundle By Name(cluster=cluster{"命令":string} {"命令"=""} ("元素"), "命令"="CODMn读取公式" ("名称（未命名）")) -> (w975:cluster{"命令":string})
        n593 = call-poly <vilib>:"Write Key.vi"("section"="标线选择", "error in (no error)"=w987, "value"="选用水样", "key"="选用水样", "refnum"=w988) -> ("error out"=w984:errorcluster, "refnum out"=w985:T6)  [unwired: 4 in, 1 out]
        n594 = call-poly <vilib>:"Read Key.vi"("section"=w958, "error in (no error)"=w984, "key"="浓度1", "refnum"=w985) -> ("error out"=w1028:errorcluster, "value"=w1026:dbl, "refnum out"=w1027:T6)  [unwired: 4 in, 1 out]
        n595 = Enqueue Element(queue=w974, element=w975, error in (no error)=w973) -> ()  [unwired: 1 in, 3 out]
        n596 = local write "浓度1"(w1026) -> ()
        n597 = call-poly <vilib>:"Read Key.vi"("section"=w958, "error in (no error)"=w1028, "key"="浓度2", "refnum"=w1027) -> ("error out"=w1042:errorcluster, "value"=w1029:dbl, "refnum out"=w1041:T6)  [unwired: 4 in, 1 out]
        n598 = local write "浓度2"(w1029) -> ()
        n599 = call-poly <vilib>:"Read Key.vi"("section"=w958, "error in (no error)"=w1042, "key"="浓度3", "refnum"=w1041) -> ("error out"=w1043:errorcluster, "value"=w1031:dbl, "refnum out"=w1040:T6)  [unwired: 4 in, 1 out]
        n600 = local write "浓度3"(w1031) -> ()
        n601 = call-poly <vilib>:"Read Key.vi"("section"=w958, "error in (no error)"=w1043, "key"="泵滴定数1", "refnum"=w1040) -> ("error out"=w1044:errorcluster, "value"=w1033:dbl, "refnum out"=w1039:T6)  [unwired: 4 in, 1 out]
        n602 = local write "泵滴定数1"(w1033) -> ()
        n603 = call-poly <vilib>:"Read Key.vi"("section"=w958, "error in (no error)"=w1044, "key"="泵滴定数2", "refnum"=w1039) -> ("error out"=w1038:errorcluster, "value"=w1036:dbl, "refnum out"=w1045:T6)  [unwired: 4 in, 1 out]
        n604 = local write "泵滴定数2"(w1036) -> ()
        n605 = call-poly <vilib>:"Read Key.vi"("section"=w958, "error in (no error)"=w1038, "key"="泵滴定数3", "refnum"=w1045) -> ("error out"=w1050:errorcluster, "value"=w1049:dbl, "refnum out"=w1046:T6)  [unwired: 4 in, 1 out]
        n606 = local write "泵滴定数3"(w1049) -> ()
        n607 = call-poly <vilib>:"Read Key.vi"("section"=w958, "error in (no error)"=w1050, "key"="浓度4", "refnum"=w1046) -> ("error out"=w1051:errorcluster, "value"=w998:dbl, "refnum out"=w1047:T6)  [unwired: 4 in, 1 out]
        n608 = local write "浓度4"(w998) -> ()
        n609 = call-poly <vilib>:"Read Key.vi"("section"=w958, "error in (no error)"=w1051, "key"="浓度5", "refnum"=w1047) -> ("error out"=w1001:errorcluster, "value"=w997:dbl, "refnum out"=w1002:T6)  [unwired: 4 in, 1 out]
        n610 = local write "浓度5"(w997) -> ()
        n611 = call-poly <vilib>:"Read Key.vi"("section"=w958, "error in (no error)"=w1001, "key"="泵滴定数4", "refnum"=w1002) -> ("error out"=w1052:errorcluster, "value"=w996:dbl, "refnum out"=w1048:T6)  [unwired: 4 in, 1 out]
        n612 = local write "泵滴定数4"(w996) -> ()
        n613 = call-poly <vilib>:"Read Key.vi"("section"=w958, "error in (no error)"=w1052, "key"="泵滴定数5", "refnum"=w1048) -> ("error out"=w999:errorcluster, "value"=w995:dbl, "refnum out"=w1000:T6)  [unwired: 4 in, 1 out]
        n614 = local write "泵滴定数5"(w995) -> ()
        n615 = call-poly <vilib>:"Read Key.vi"("section"=w958, "error in (no error)"=w999, "key"="当前选用的校准", "refnum"=w1000) -> ("error out"=w1022:errorcluster, "refnum out"=w1023:T6)  [unwired: 4 in, 2 out]
        n616 = call-poly <vilib>:"Read Key.vi"("section"=w958, "error in (no error)"=w1022, "key"="启用1", "refnum"=w1023) -> ("error out"=w1019:errorcluster, "value"=w1008:bool, "refnum out"=w1020:T6)  [unwired: 4 in, 1 out]
        n617 = local write "启用1"(w1008) -> ()
        n618 = call-poly <vilib>:"Read Key.vi"("section"=w958, "error in (no error)"=w1019, "key"="启用2", "refnum"=w1020) -> ("error out"=w1017:errorcluster, "value"=w1007:bool, "refnum out"=w1018:T6)  [unwired: 4 in, 1 out]
        n619 = local write "启用2"(w1007) -> ()
        n620 = call-poly <vilib>:"Read Key.vi"("section"=w958, "error in (no error)"=w1017, "key"="启用3", "refnum"=w1018) -> ("error out"=w1015:errorcluster, "value"=w1006:bool, "refnum out"=w1016:T6)  [unwired: 4 in, 1 out]
        n621 = local write "启用3"(w1006) -> ()
        n622 = call-poly <vilib>:"Read Key.vi"("section"=w958, "error in (no error)"=w1015, "key"="启用4", "refnum"=w1016) -> ("error out"=w1013:errorcluster, "value"=w994:bool, "refnum out"=w1014:T6)  [unwired: 4 in, 1 out]
        n623 = local write "启用4"(w994) -> ()
        n624 = call-poly <vilib>:"Read Key.vi"("section"=w958, "error in (no error)"=w1013, "key"="启用5", "refnum"=w1014) -> ("error out"=w955:errorcluster, "value"=w993:bool, "refnum out"=w959:T6)  [unwired: 4 in, 1 out]
        n625 = call-poly <vilib>:"Read Key.vi"("section"=w958, "error in (no error)"=w955, "key"="零点校准时间", "refnum"=w959) -> ("error out"=w971:errorcluster, "value"=w940:string, "refnum out"=w970:T6)  [unwired: 4 in, 1 out]
        n626 = Unflatten From String(type=timestamp(0 s since 1904-01-01), binary string=w940) -> (value=w941:timestamp)  [unwired: 3 in, 2 out]
        n627 = call-poly <vilib>:"Read Key.vi"("section"=w958, "error in (no error)"=w971, "key"="标液1校准时间", "refnum"=w970) -> ("error out"=w966:errorcluster, "value"=w943:string, "refnum out"=w963:T6)  [unwired: 4 in, 1 out]
        n628 = local write "零点校准时间"(w941) -> ()
        n629 = Unflatten From String(type=timestamp(0 s since 1904-01-01), binary string=w943) -> (value=w942:timestamp)  [unwired: 3 in, 2 out]
        n630 = call-poly <vilib>:"Read Key.vi"("section"=w958, "error in (no error)"=w966, "key"="标液2校准时间", "refnum"=w963) -> ("error out"=w967:errorcluster, "value"=w946:string, "refnum out"=w961:T6)  [unwired: 4 in, 1 out]
        n631 = local write "标液校准时间1"(w942) -> ()
        n632 = local write "启用5"(w993) -> ()
        n633 = Unflatten From String(type=timestamp(0 s since 1904-01-01), binary string=w946) -> (value=w945:timestamp)  [unwired: 3 in, 2 out]
        n634 = call-poly <vilib>:"Read Key.vi"("section"=w958, "error in (no error)"=w967, "key"="标液3校准时间", "refnum"=w961) -> ("error out"=w968:errorcluster, "value"=w949:string, "refnum out"=w969:T6)  [unwired: 4 in, 1 out]
        n635 = local write "标液校准时间2"(w945) -> ()
        n636 = Unflatten From String(type=timestamp(0 s since 1904-01-01), binary string=w949) -> (value=w948:timestamp)  [unwired: 3 in, 2 out]
        n637 = call-poly <vilib>:"Read Key.vi"("section"=w958, "error in (no error)"=w968, "key"="标液4校准时间", "refnum"=w969) -> ("error out"=w956:errorcluster, "value"=w952:string, "refnum out"=w957:T6)  [unwired: 4 in, 1 out]
        n638 = call <vilib>:"Close Config Data.vi"("error in (no error)"=w956, "refnum"=w957) -> ("error out"=w978:errorcluster, "file path"=w979:path)  [unwired: 8 in]
        n639 = Open/Create/Replace File(file path (use dialog)=w979, error in=w978) -> (refnum out=w981:refnum<file>, error out=w980:errorcluster)  [unwired: 4 in, 1 out]
        n640 = Flush File(refnum=w981, error in=w980) -> (refnum out=w982:refnum<file>, error out=w983:errorcluster)
        n641 = Close File(refnum=w982, error in=w983) -> ()  [unwired: 2 out]
        n642 = local write "标液校准时间3"(w948) -> ()
        n643 = Unflatten From String(type=timestamp(0 s since 1904-01-01), binary string=w952) -> (value=w951:timestamp)  [unwired: 3 in, 2 out]
        n644 = local write "标液校准时间4"(w951) -> ()
      }
      event "量程选择": Value Change {
        w1115 = "量程选择" ("section")
        n645 = event-data() -> ()  [unwired: 1 in, 6 out]
        n646 = local read "选用水样"() -> (w1130:enum16{"葡萄糖", "草酸钠"})
        n647 = property on="窗格" class="Pane"("Origin"=T4 {"Horizontal"=0, "Vertical"=1300} ("原点")) -> ()  [unwired: 2 in, 2 out]
        n648 = Bundle By Name(cluster=cluster{"命令":string} {"命令"=""} ("元素"), "命令"="CODMn读取公式" ("名称（未命名）")) -> (w1101:cluster{"命令":string})
        n649 = case shown="\"葡萄糖\", 默认" w1130 {
          tunnel: ["葡萄糖标线" ("section") "草酸钠标线" ("section")] -> w1129
          frame "葡萄糖", Default {
          }
          frame "草酸钠" {
          }
        }
        n650 = global read "CODMN外部API.vi" "ping"() -> (w1117:bool)
        n651 = case shown="\"高量程\"" "量程选择" {
          tunnel: ["低量程" "高量程"] -> w1128
          frame "低量程", Default {
          }
          frame "高量程" {
          }
        }
        n652 = Enqueue Element(queue=w1100, element=w1101, error in (no error)=w1099) -> ()  [unwired: 1 in, 3 out]
        n653 = case shown="假" w1117 {
          tunnel: [w1183 w1186] -> w1116
          frame False {
            n654 = global read "COD内部交互全局.vi" "配置文件ini"() -> (w1185:string)
            n655 = call <vilib>:"Application Directory.vi"() -> ("Application Directory"=w1184:path)
            n656 = Build Path(base path=w1184, name or relative path=w1185) -> (appended path=w1183:path)
          }
          frame True {
            n657 = global read "CODMN外部API.vi" "配置文件 path"() -> (w1186:path)
          }
        }
        n658 = Concatenate Strings(w1129, w1128) -> (w1066:string)
        n659 = call <vilib>:"Open Config Data.vi"("configuration file path"=w1116) -> ("error out"=w1114:errorcluster, "refnum"=w1113:T6)  [unwired: 8 in, 1 out]
        n660 = call-poly <vilib>:"Write Key.vi"("section"=w1115, "error in (no error)"=w1114, "value"="量程选择", "key"=w1115, "refnum"=w1113) -> ("error out"=w1110:errorcluster, "refnum out"=w1112:T6)  [unwired: 4 in, 1 out]
        n661 = call-poly <vilib>:"Read Key.vi"("section"=w1066, "error in (no error)"=w1110, "key"="浓度1", "refnum"=w1112) -> ("error out"=w1153:errorcluster, "value"=w1151:dbl, "refnum out"=w1152:T6)  [unwired: 4 in, 1 out]
        n662 = local write "浓度1"(w1151) -> ()
        n663 = call-poly <vilib>:"Read Key.vi"("section"=w1066, "error in (no error)"=w1153, "key"="浓度2", "refnum"=w1152) -> ("error out"=w1167:errorcluster, "value"=w1154:dbl, "refnum out"=w1166:T6)  [unwired: 4 in, 1 out]
        n664 = local write "浓度2"(w1154) -> ()
        n665 = call-poly <vilib>:"Read Key.vi"("section"=w1066, "error in (no error)"=w1167, "key"="浓度3", "refnum"=w1166) -> ("error out"=w1168:errorcluster, "value"=w1156:dbl, "refnum out"=w1165:T6)  [unwired: 4 in, 1 out]
        n666 = local write "浓度3"(w1156) -> ()
        n667 = call-poly <vilib>:"Read Key.vi"("section"=w1066, "error in (no error)"=w1168, "key"="泵滴定数1", "refnum"=w1165) -> ("error out"=w1169:errorcluster, "value"=w1158:dbl, "refnum out"=w1164:T6)  [unwired: 4 in, 1 out]
        n668 = local write "泵滴定数1"(w1158) -> ()
        n669 = call-poly <vilib>:"Read Key.vi"("section"=w1066, "error in (no error)"=w1169, "key"="泵滴定数2", "refnum"=w1164) -> ("error out"=w1163:errorcluster, "value"=w1161:dbl, "refnum out"=w1170:T6)  [unwired: 4 in, 1 out]
        n670 = local write "泵滴定数2"(w1161) -> ()
        n671 = call-poly <vilib>:"Read Key.vi"("section"=w1066, "error in (no error)"=w1163, "key"="泵滴定数3", "refnum"=w1170) -> ("error out"=w1175:errorcluster, "value"=w1174:dbl, "refnum out"=w1171:T6)  [unwired: 4 in, 1 out]
        n672 = local write "泵滴定数3"(w1174) -> ()
        n673 = call-poly <vilib>:"Read Key.vi"("section"=w1066, "error in (no error)"=w1175, "key"="浓度4", "refnum"=w1171) -> ("error out"=w1176:errorcluster, "value"=w1121:dbl, "refnum out"=w1172:T6)  [unwired: 4 in, 1 out]
        n674 = local write "浓度4"(w1121) -> ()
        n675 = call-poly <vilib>:"Read Key.vi"("section"=w1066, "error in (no error)"=w1176, "key"="浓度5", "refnum"=w1172) -> ("error out"=w1126:errorcluster, "value"=w1120:dbl, "refnum out"=w1127:T6)  [unwired: 4 in, 1 out]
        n676 = local write "浓度5"(w1120) -> ()
        n677 = call-poly <vilib>:"Read Key.vi"("section"=w1066, "error in (no error)"=w1126, "key"="泵滴定数4", "refnum"=w1127) -> ("error out"=w1177:errorcluster, "value"=w1119:dbl, "refnum out"=w1173:T6)  [unwired: 4 in, 1 out]
        n678 = local write "泵滴定数4"(w1119) -> ()
        n679 = call-poly <vilib>:"Read Key.vi"("section"=w1066, "error in (no error)"=w1177, "key"="泵滴定数5", "refnum"=w1173) -> ("error out"=w1124:errorcluster, "value"=w1118:dbl, "refnum out"=w1125:T6)  [unwired: 4 in, 1 out]
        n680 = local write "泵滴定数5"(w1118) -> ()
        n681 = call-poly <vilib>:"Read Key.vi"("section"=w1066, "error in (no error)"=w1124, "key"="当前选用的校准", "refnum"=w1125) -> ("error out"=w1147:errorcluster, "refnum out"=w1148:T6)  [unwired: 4 in, 2 out]
        n682 = call-poly <vilib>:"Read Key.vi"("section"=w1066, "error in (no error)"=w1147, "key"="启用1", "refnum"=w1148) -> ("error out"=w1144:errorcluster, "value"=w1133:bool, "refnum out"=w1145:T6)  [unwired: 4 in, 1 out]
        n683 = local write "启用1"(w1133) -> ()
        n684 = call-poly <vilib>:"Read Key.vi"("section"=w1066, "error in (no error)"=w1144, "key"="启用2", "refnum"=w1145) -> ("error out"=w1142:errorcluster, "value"=w1132:bool, "refnum out"=w1143:T6)  [unwired: 4 in, 1 out]
        n685 = local write "启用2"(w1132) -> ()
        n686 = call-poly <vilib>:"Read Key.vi"("section"=w1066, "error in (no error)"=w1142, "key"="启用3", "refnum"=w1143) -> ("error out"=w1140:errorcluster, "value"=w1131:bool, "refnum out"=w1141:T6)  [unwired: 4 in, 1 out]
        n687 = local write "启用3"(w1131) -> ()
        n688 = call-poly <vilib>:"Read Key.vi"("section"=w1066, "error in (no error)"=w1140, "key"="启用4", "refnum"=w1141) -> ("error out"=w1138:errorcluster, "value"=w1123:bool, "refnum out"=w1139:T6)  [unwired: 4 in, 1 out]
        n689 = local write "启用4"(w1123) -> ()
        n690 = call-poly <vilib>:"Read Key.vi"("section"=w1066, "error in (no error)"=w1138, "key"="启用5", "refnum"=w1139) -> ("error out"=w1068:errorcluster, "value"=w1122:bool, "refnum out"=w1067:T6)  [unwired: 4 in, 1 out]
        n691 = call-poly <vilib>:"Read Key.vi"("section"=w1066, "error in (no error)"=w1068, "key"="零点校准时间", "refnum"=w1067) -> ("error out"=w1097:errorcluster, "value"=w1071:string, "refnum out"=w1096:T6)  [unwired: 4 in, 1 out]
        n692 = Unflatten From String(type=timestamp(0 s since 1904-01-01), binary string=w1071) -> (value=w1072:timestamp)  [unwired: 3 in, 2 out]
        n693 = call-poly <vilib>:"Read Key.vi"("section"=w1066, "error in (no error)"=w1097, "key"="标液1校准时间", "refnum"=w1096) -> ("error out"=w1092:errorcluster, "value"=w1074:string, "refnum out"=w1089:T6)  [unwired: 4 in, 1 out]
        n694 = local write "零点校准时间"(w1072) -> ()
        n695 = Unflatten From String(type=timestamp(0 s since 1904-01-01), binary string=w1074) -> (value=w1073:timestamp)  [unwired: 3 in, 2 out]
        n696 = call-poly <vilib>:"Read Key.vi"("section"=w1066, "error in (no error)"=w1092, "key"="标液2校准时间", "refnum"=w1089) -> ("error out"=w1093:errorcluster, "value"=w1077:string, "refnum out"=w1087:T6)  [unwired: 4 in, 1 out]
        n697 = local write "标液校准时间1"(w1073) -> ()
        n698 = local write "启用5"(w1122) -> ()
        n699 = Unflatten From String(type=timestamp(0 s since 1904-01-01), binary string=w1077) -> (value=w1076:timestamp)  [unwired: 3 in, 2 out]
        n700 = call-poly <vilib>:"Read Key.vi"("section"=w1066, "error in (no error)"=w1093, "key"="标液3校准时间", "refnum"=w1087) -> ("error out"=w1094:errorcluster, "value"=w1080:string, "refnum out"=w1095:T6)  [unwired: 4 in, 1 out]
        n701 = local write "标液校准时间2"(w1076) -> ()
        n702 = Unflatten From String(type=timestamp(0 s since 1904-01-01), binary string=w1080) -> (value=w1079:timestamp)  [unwired: 3 in, 2 out]
        n703 = call-poly <vilib>:"Read Key.vi"("section"=w1066, "error in (no error)"=w1094, "key"="标液4校准时间", "refnum"=w1095) -> ("error out"=w1069:errorcluster, "value"=w1083:string, "refnum out"=w1070:T6)  [unwired: 4 in, 1 out]
        n704 = call <vilib>:"Close Config Data.vi"("error in (no error)"=w1069, "refnum"=w1070) -> ("error out"=w1104:errorcluster, "file path"=w1105:path)  [unwired: 8 in]
        n705 = Open/Create/Replace File(file path (use dialog)=w1105, error in=w1104) -> (refnum out=w1107:refnum<file>, error out=w1106:errorcluster)  [unwired: 4 in, 1 out]
        n706 = Flush File(refnum=w1107, error in=w1106) -> (refnum out=w1108:refnum<file>, error out=w1109:errorcluster)
        n707 = Close File(refnum=w1108, error in=w1109) -> ()  [unwired: 2 out]
        n708 = local write "标液校准时间3"(w1079) -> ()
        n709 = Unflatten From String(type=timestamp(0 s since 1904-01-01), binary string=w1083) -> (value=w1082:timestamp)  [unwired: 3 in, 2 out]
        n710 = local write "标液校准时间4"(w1082) -> ()
      }
      event "返回": Value Change {
        w1212 = "CODMn" ("section")
        n711 = event-data() -> ()  [unwired: 1 in, 6 out]
        n712 = property on="窗格" class="Pane"("Origin"=T4 {"Horizontal"=0, "Vertical"=0} ("原点")) -> ()  [unwired: 2 in, 2 out]
        n713 = global read "CODMN外部API.vi" "ping"() -> (w1198:bool)
        n714 = case shown="假" w1198 {
          tunnel: [w1263 w1266] -> w1197
          frame False {
            n715 = global read "COD内部交互全局.vi" "配置文件ini"() -> (w1265:string)
            n716 = call <vilib>:"Application Directory.vi"() -> ("Application Directory"=w1264:path)
            n717 = Build Path(base path=w1264, name or relative path=w1265) -> (appended path=w1263:path)
          }
          frame True {
            n718 = global read "CODMN外部API.vi" "配置文件 path"() -> (w1266:path)
          }
        }
        n719 = call <vilib>:"Open Config Data.vi"("configuration file path"=w1197) -> ("error out"=w1261:errorcluster, "refnum"=w1262:T6)  [unwired: 8 in, 1 out]
        n720 = local read "浓度1"() -> (w1259:dbl)
        n721 = call-poly <vilib>:"Write Key.vi"("section"=w1212, "error in (no error)"=w1261, "value"=w1259, "key"="浓度1", "refnum"=w1262) -> ("error out"=w1258:errorcluster, "refnum out"=w1257:T6)  [unwired: 4 in, 1 out]
        n722 = local read "浓度2"() -> (w1243:dbl)
        n723 = call-poly <vilib>:"Write Key.vi"("section"=w1212, "error in (no error)"=w1258, "value"=w1243, "key"="浓度2", "refnum"=w1257) -> ("error out"=w1256:errorcluster, "refnum out"=w1255:T6)  [unwired: 4 in, 1 out]
        n724 = local read "浓度3"() -> (w1239:dbl)
        n725 = local read "泵滴定数1"() -> (w1237:dbl)
        n726 = call-poly <vilib>:"Write Key.vi"("section"=w1212, "error in (no error)"=w1256, "value"=w1239, "key"="浓度3", "refnum"=w1255) -> ("error out"=w1254:errorcluster, "refnum out"=w1253:T6)  [unwired: 4 in, 1 out]
        n727 = local read "泵滴定数2"() -> (w1235:dbl)
        n728 = call-poly <vilib>:"Write Key.vi"("section"=w1212, "error in (no error)"=w1254, "value"=w1237, "key"="泵滴定数1", "refnum"=w1253) -> ("error out"=w1252:errorcluster, "refnum out"=w1251:T6)  [unwired: 4 in, 1 out]
        n729 = local read "泵滴定数3"() -> (w1233:dbl)
        n730 = call-poly <vilib>:"Write Key.vi"("section"=w1212, "error in (no error)"=w1252, "value"=w1235, "key"="泵滴定数2", "refnum"=w1251) -> ("error out"=w1250:errorcluster, "refnum out"=w1249:T6)  [unwired: 4 in, 1 out]
        n731 = call-poly <vilib>:"Write Key.vi"("section"=w1212, "error in (no error)"=w1250, "value"=w1233, "key"="泵滴定数3", "refnum"=w1249) -> ("error out"=w1248:errorcluster, "refnum out"=w1247:T6)  [unwired: 4 in, 1 out]
        n732 = local read "浓度4"() -> (w1200:dbl)
        n733 = call-poly <vilib>:"Write Key.vi"("section"=w1212, "error in (no error)"=w1248, "value"=w1200, "key"="浓度4", "refnum"=w1247) -> ("error out"=w1241:errorcluster, "refnum out"=w1242:T6)  [unwired: 4 in, 1 out]
        n734 = local read "浓度5"() -> (w1199:dbl)
        n735 = local read "泵滴定数4"() -> (w1201:dbl)
        n736 = call-poly <vilib>:"Write Key.vi"("section"=w1212, "error in (no error)"=w1241, "value"=w1199, "key"="浓度5", "refnum"=w1242) -> ("error out"=w1209:errorcluster, "refnum out"=w1210:T6)  [unwired: 4 in, 1 out]
        n737 = local read "泵滴定数5"() -> (w1202:dbl)
        n738 = call-poly <vilib>:"Write Key.vi"("section"=w1212, "error in (no error)"=w1209, "value"=w1201, "key"="泵滴定数4", "refnum"=w1210) -> ("error out"=w1246:errorcluster, "refnum out"=w1245:T6)  [unwired: 4 in, 1 out]
        n739 = call-poly <vilib>:"Write Key.vi"("section"=w1212, "error in (no error)"=w1246, "value"=w1202, "key"="泵滴定数5", "refnum"=w1245) -> ("error out"=w1207:errorcluster, "refnum out"=w1208:T6)  [unwired: 4 in, 1 out]
        n740 = local read "启用1"() -> (w1221:bool)
        n741 = call-poly <vilib>:"Write Key.vi"("section"=w1212, "error in (no error)"=w1207, "value"=w1221, "key"="启用1", "refnum"=w1208) -> ("error out"=w1217:errorcluster, "refnum out"=w1220:T6)  [unwired: 4 in, 1 out]
        n742 = local read "启用2"() -> (w1218:bool)
        n743 = call-poly <vilib>:"Write Key.vi"("section"=w1212, "error in (no error)"=w1217, "value"=w1218, "key"="启用2", "refnum"=w1220) -> ("error out"=w1228:errorcluster, "refnum out"=w1227:T6)  [unwired: 4 in, 1 out]
        n744 = local read "启用3"() -> (w1216:bool)
        n745 = call-poly <vilib>:"Write Key.vi"("section"=w1212, "error in (no error)"=w1228, "value"=w1216, "key"="启用3", "refnum"=w1227) -> ("error out"=w1226:errorcluster, "refnum out"=w1225:T6)  [unwired: 4 in, 1 out]
        n746 = local read "启用4"() -> (w1204:bool)
        n747 = call-poly <vilib>:"Write Key.vi"("section"=w1212, "error in (no error)"=w1226, "value"=w1204, "key"="启用4", "refnum"=w1225) -> ("error out"=w1224:errorcluster, "refnum out"=w1223:T6)  [unwired: 4 in, 1 out]
        n748 = local read "启用5"() -> (w1203:bool)
        n749 = call-poly <vilib>:"Write Key.vi"("section"=w1212, "error in (no error)"=w1224, "value"=w1203, "key"="启用5", "refnum"=w1223) -> ("error out"=w1205:errorcluster, "refnum out"=w1206:T6)  [unwired: 4 in, 1 out]
        n750 = call <vilib>:"Close Config Data.vi"("error in (no error)"=w1205, "refnum"=w1206) -> ("error out"=w1191:errorcluster, "file path"=w1192:path)  [unwired: 8 in]
        n751 = Open/Create/Replace File(file path (use dialog)=w1192, error in=w1191) -> (refnum out=w1194:refnum<file>, error out=w1193:errorcluster)  [unwired: 4 in, 1 out]
        n752 = Flush File(refnum=w1194, error in=w1193) -> (refnum out=w1195:refnum<file>, error out=w1196:errorcluster)
        n753 = Close File(refnum=w1195, error in=w1196) -> ()  [unwired: 2 out]
      }
      event "关闭", "关闭 2", "关闭 3", "关闭 4": Value Change {
        n754 = event-data() -> ()  [unwired: 1 in, 6 out]
        n755 = property on="窗格" class="Pane"("Origin"=T4 {"Horizontal"=0, "Vertical"=0} ("原点")) -> ()  [unwired: 2 in, 2 out]
      }
      event Application Instance Close {
        n756 = event-data() -> ()  [unwired: 1 in, 4 out]
      }
      event "时间校准": Value Change {
        n757 = event-data() -> ()  [unwired: 1 in, 6 out]
        n758 = Get Date/Time In Seconds() -> (seconds since 1Jan1904=w1276:timestamp)
        n759 = Build Array(w1276) -> (w1275:timestamp[])
        n760 = call "DateToHex.vi"("DATE"=w1275) -> ("数组"=w1273:u16[])  [unwired: 10 in]
        n761 = Insert Into Array(array=u16[] [1] ("values"), index=1 ("索引"), new element=w1273) -> (w1269:u16[])
        n762 = call "CODMnMB_api.vi"("STEP"=enum16{"open", "read", "write", "close"}."write", "values"=w1269, "starting address"=u16 4612) -> ("error out"=w1268:errorcluster)  [unwired: 6 in, 2 out]
        n763 = call <vilib>:"Clear Errors.vi"("error in (no error)"=w1268) -> ()  [unwired: 5 in, 2 out]
      }
      event "故障清除": Value Change {
        n764 = event-data() -> ()  [unwired: 1 in, 6 out]
        n765 = call "CODMnMB_api.vi"("STEP"=enum16{"open", "read", "write", "close"}."write", "values"=u16[] [1], "starting address"=u16 4611) -> ()  [unwired: 6 in, 3 out]
      }
      event "仪器参数": Value Change {
        n766 = event-data() -> ()  [unwired: 1 in, 6 out]
        n767 = global read "CODMn断电保存全局变量.vi" "CODMn仪器参数"() -> (w1280:T12)
        n768 = call "仪器参数设置.vi"("氨氮仪器参数"=w1280) -> ("仪器参数设置输出"=w1281:T18)  [unwired: 10 in]
        n769 = Unbundle By Name(w1281) -> ("确定"=w1282:bool)
        n770 = case shown="真" w1282 {
          tunnel: w1281 -> [_ w1284]
          tunnel: w1280 -> [_ w1283]
          frame False {
          }
          frame True {
            n771 = flat-sequence {
              tunnel: w1284 -> [w1301]
              tunnel: w1283 -> [w1300]
              frame #0 {
                n772 = Unbundle By Name(w1301) -> ("测量量程"=w1299:dbl, "测量精度"=w1298:dbl, "测量间隔"=w1297:dbl, "消解温度"=w1296:dbl, "消解时长"=w1295:dbl, "空白校准时间"=w1294:timestamp, "曲线截距"=w1293:dbl, "曲线斜率"=w1292:dbl, "测量检出限"=w1291:dbl, "测量信号值"=w1290:dbl, "线性相关系数"=w1289:dbl, "二次多项式系数"=w1288:dbl, "标样校准时间"=w1287:timestamp, "稀释倍数"=w1286:dbl)
                n773 = Bundle By Name(cluster=w1300, "测量量程"=w1299, "测量精度"=w1298, "测量间隔"=w1297, "消解温度"=w1296, "消解时长"=w1295, "空白校准时间"=w1294, "曲线截距"=w1293, "曲线斜率"=w1292, "测量检出限"=w1291, "测量信号值"=w1290, "线性相关系数"=w1289, "二次多项式系数"=w1288, "标样校准时间"=w1287, "稀释倍数"=w1286) -> (w1285:T12)
                n774 = global write "CODMn断电保存全局变量.vi" "CODMn仪器参数"(w1285) -> ()
              }
              frame #1 {
                n775 = call "配置文件保存.vi"() -> ()  [unwired: 12 in]
              }
            }
          }
        }
      }
      event "跨度量程选择", "跨度液浓度", "零点核查量程选择", "零点核查浓度", "标样浓度", "标样核查量程选择", "加标回收量程：", "跨度值": Value Change {
        n776 = event-data() -> ()  [unwired: 1 in, 6 out]
        n777 = flat-sequence {
          frame #0 {
            n778 = global write "CODMn断电保存全局变量.vi" "标样浓度"("标样浓度") -> ()
            n779 = global write "CODMn断电保存全局变量.vi" "零点核查浓度"("零点核查浓度") -> ()
            n780 = global write "CODMn断电保存全局变量.vi" "跨度液浓度"("跨度液浓度") -> ()
            n781 = global write "CODMn断电保存全局变量.vi" "CODMn跨度量程选择"("跨度量程选择") -> ()
            n782 = global write "CODMn断电保存全局变量.vi" "加标回收量程选择"("加标回收量程：") -> ()
            n783 = global write "CODMn断电保存全局变量.vi" "跨度值"("跨度值") -> ()
            n784 = global write "CODMn断电保存全局变量.vi" "标样核查量程选择"("标样核查量程选择") -> ()
            n785 = global write "CODMn断电保存全局变量.vi" "零点核查量程选择"("零点核查量程选择") -> ()
          }
          frame #1 {
            n786 = call "配置文件保存.vi"() -> ()  [unwired: 12 in]
          }
        }
      }
      event "校准1", "校准2", "校准3", "校准4", "校准5": Value Change {
        n787 = event-data() -> ()  [unwired: 1 in, 6 out]
        n788 = flat-sequence {
          tunnel: w1313 -> [w1322]
          tunnel: [w1322] -> w1315
          tunnel: w1310 -> [w1321]
          tunnel: [w1321] -> w1312
          tunnel: w1315 -> [w1357]
          tunnel: [w1357] -> w1314
          tunnel: w1312 -> [w1356]
          tunnel: [w1356] -> w1311
          tunnel: w1314 -> [w1384]
          tunnel: w1311 -> [w1383]
          frame #0 {
            n789 = Build Array("校准1", "校准2", "校准3", "校准4", "校准5") -> (w1325:bool[])
            n790 = for {
              tunnel: w1325 -> [w1339] mode=indexing
              tunnel: [w1331] -> w1316
              i -> [w1332]
              n791 = case shown="4" w1332 {
                tunnel: ["浓度1" "浓度2" "浓度3" "浓度4" "浓度5"] -> w1335
                frame 0, Default {
                }
                frame 1 {
                }
                frame 2 {
                }
                frame 3 {
                }
                frame 4 {
                }
              }
              n792 = Multiply(x=w1335, y=100.0) -> (x*y=w1333:dbl)
              n793 = Insert Into Array(array=u16[] [] ("values"), index=0 ("索引"), new element=w1333) -> (w1336:u16[])
              n794 = case shown="真" w1339 {
                tunnel: w1336 -> [_ w1348]
                tunnel: w1332 -> [_ w1350]
                tunnel: [_ w1345] -> w1331
                frame False {
                }
                frame True {
                  n795 = Increment(x=w1350) -> (x+1=w1346:i32)
                  n796 = global write "COD内部交互全局.vi" "当前校准"(w1346) -> ()
                  n797 = call "CODMnMB_api.vi"("STEP"=enum16{"open", "read", "write", "close"}."write", "values"=w1348, "starting address"=u16 4274) -> ("error out"=w1345:errorcluster)  [unwired: 6 in, 2 out]
                }
              }
            }
            n798 = local read "量程选择"() -> (w1318:enum16{"低量程", "高量程"})
            n799 = case shown="\"高量程\"" w1318 {
              tunnel: [u16[] [0] ("values") u16[] [1] ("values")] -> w1317
              frame "低量程", Default {
              }
              frame "高量程" {
              }
            }
            n800 = call "CODMnMB_api.vi"("STEP"=enum16{"open", "read", "write", "close"}."write", "Error in"=w1316, "values"=w1317, "starting address"=u16 4276) -> ()  [unwired: 5 in, 3 out]
          }
          frame #1 {
            n801 = global read "COD内部交互全局.vi" "当前校准"() -> (w1358:i32)
            n802 = case shown="5" w1358 {
              tunnel: [w1366 w1367 w1368 w1369 w1370] -> w1354
              frame 1, Default {
                n803 = local read "浓度1"() -> (w1366:dbl)
              }
              frame 2 {
                n804 = local read "浓度2"() -> (w1367:dbl)
              }
              frame 3 {
                n805 = local read "浓度3"() -> (w1368:dbl)
              }
              frame 4 {
                n806 = local read "浓度4"() -> (w1369:dbl)
              }
              frame 5 {
                n807 = local read "浓度5"() -> (w1370:dbl)
              }
            }
            n808 = Number To Decimal String(number=w1354) -> (decimal integer string=w1353:string)  [unwired: 1 in]
            n809 = Concatenate Strings("仪器校准中!\n当前校准浓度为:", w1353, "mg/L" ("字符串")) -> (w1351:string)
            n810 = Not Equal To 0?(x=w1354) -> (x != 0?=w1362:bool)
            n811 = global write "COD内部交互全局.vi" "校准内容显示"(w1351) -> ()
            n812 = case shown="真" w1362 {
              tunnel: [u16 8 ("address") u16 9 ("address")] -> w1365
              tunnel: ["校零" ("测量模式") "校标" ("测量模式")] -> _
              frame False {
              }
              frame True {
              }
            }
            n813 = Insert Into Array(array=u16[] [] ("values"), index=0 ("索引"), new element=w1365) -> (w1359:u16[])
            n814 = call "CODMnMB_api.vi"("STEP"=enum16{"open", "read", "write", "close"}."write", "values"=w1359, "starting address"=u16 4608 ("address")) -> ()  [unwired: 6 in, 3 out]
          }
          frame #2 {
            n815 = local read "选用水样"() -> (w1392:enum16{"葡萄糖", "草酸钠"})
            n816 = global read "CODMN外部API.vi" "ping"() -> (w1382:bool)
            n817 = case shown="假" w1382 {
              tunnel: [w1400 w1403] -> w1381
              frame False {
                n818 = global read "COD内部交互全局.vi" "配置文件ini"() -> (w1402:string)
                n819 = call <vilib>:"Application Directory.vi"() -> ("Application Directory"=w1401:path)
                n820 = Build Path(base path=w1401, name or relative path=w1402) -> (appended path=w1400:path)
              }
              frame True {
                n821 = global read "CODMN外部API.vi" "配置文件 path"() -> (w1403:path)
              }
            }
            n822 = local read "量程选择"() -> (w1391:enum16{"低量程", "高量程"})
            n823 = case shown="\"葡萄糖\", 默认" w1392 {
              tunnel: ["葡萄糖标线" ("section") "草酸钠标线" ("section")] -> w1393
              frame "葡萄糖", Default {
              }
              frame "草酸钠" {
              }
            }
            n824 = Bundle By Name(cluster=cluster{"命令":string} {"命令"=""} ("元素"), "命令"="CODMn读取参数" ("名称（未命名）")) -> (w1388:cluster{"命令":string})
            n825 = case shown="\"低量程\", 默认" w1391 {
              tunnel: ["低量程" "高量程"] -> w1394
              frame "低量程", Default {
              }
              frame "高量程" {
              }
            }
            n826 = global read "COD内部交互全局.vi" "当前校准"() -> (w1389:i32)
            n827 = Enqueue Element(queue=w1384, element=w1388, timeout in ms (-1)=1000 ("超时毫秒(-1)"), error in (no error)=w1383) -> ()  [unwired: 3 out]
            n828 = Concatenate Strings(w1393, w1394) -> (w1390:string)
            n829 = call <vilib>:"Open Config Data.vi"("configuration file path"=w1381) -> ("error out"=w1398:errorcluster, "refnum"=w1399:T6)  [unwired: 8 in, 1 out]
            n830 = call-poly <vilib>:"Write Key.vi"("section"=w1390, "error in (no error)"=w1398, "value"=w1389, "key"="当前选用的校准" ("section"), "refnum"=w1399) -> ("error out"=w1395:errorcluster, "refnum out"=w1396:T6)  [unwired: 4 in, 1 out]
            n831 = call <vilib>:"Close Config Data.vi"("error in (no error)"=w1395, "refnum"=w1396) -> ("error out"=w1375:errorcluster, "file path"=w1376:path)  [unwired: 8 in]
            n832 = Open/Create/Replace File(file path (use dialog)=w1376, error in=w1375) -> (refnum out=w1378:refnum<file>, error out=w1377:errorcluster)  [unwired: 4 in, 1 out]
            n833 = Flush File(refnum=w1378, error in=w1377) -> (refnum out=w1379:refnum<file>, error out=w1380:errorcluster)
            n834 = Close File(refnum=w1379, error in=w1380) -> ()  [unwired: 2 out]
          }
        }
      }
      event "水样量程选择:", "低切高阈值:", "高切低阈值:": Value Change {
        n835 = event-data() -> ()  [unwired: 1 in, 6 out]
        n836 = flat-sequence {
          frame #0 {
            n837 = global write "CODMn断电保存全局变量.vi" "高切低阈值:"("高切低阈值:") -> ()
            n838 = global write "CODMn断电保存全局变量.vi" "自动切换量程:"("水样量程选择:") -> ()
            n839 = global write "CODMn断电保存全局变量.vi" "低切高阈值:"("低切高阈值:") -> ()
          }
          frame #1 {
            n840 = call "配置文件保存.vi"() -> ()  [unwired: 12 in]
          }
        }
      }
      event "模型": Value Change {
        n841 = event-data() -> ()  [unwired: 1 in, 6 out]
        n842 = global read "CODMN外部API.vi" "ping"() -> (w1418:bool)
        n843 = case shown="假" w1418 {
          tunnel: [w1426 w1429] -> w1417
          frame False {
            n844 = global read "COD内部交互全局.vi" "配置文件ini"() -> (w1428:string)
            n845 = call <vilib>:"Application Directory.vi"() -> ("Application Directory"=w1427:path)
            n846 = Build Path(base path=w1427, name or relative path=w1428) -> (appended path=w1426:path)
          }
          frame True {
            n847 = global read "CODMN外部API.vi" "配置文件 path"() -> (w1429:path)
          }
        }
        n848 = call <vilib>:"Open Config Data.vi"("configuration file path"=w1417) -> ("error out"=w1424:errorcluster, "refnum"=w1425:T6)  [unwired: 8 in, 1 out]
        n849 = local read "模型"() -> (w1419:enum32{"线性", "多项式", "折线"})
        n850 = call-poly <vilib>:"Write Key.vi"("section"="CODMn模型选择" ("key"), "error in (no error)"=w1424, "value"=w1419, "key"="线性和多项式", "refnum"=w1425) -> ("error out"=w1420:errorcluster, "refnum out"=w1421:T6)  [unwired: 4 in, 1 out]
        n851 = call <vilib>:"Close Config Data.vi"("error in (no error)"=w1420, "refnum"=w1421) -> ("error out"=w1411:errorcluster, "file path"=w1412:path)  [unwired: 8 in]
        n852 = Open/Create/Replace File(file path (use dialog)=w1412, error in=w1411) -> (refnum out=w1414:refnum<file>, error out=w1413:errorcluster)  [unwired: 4 in, 1 out]
        n853 = Flush File(refnum=w1414, error in=w1413) -> (refnum out=w1415:refnum<file>, error out=w1416:errorcluster)
        n854 = Close File(refnum=w1415, error in=w1416) -> ()  [unwired: 2 out]
      }
      event "浓度1", "浓度2", "浓度3", "泵滴定数1", "泵滴定数2", "泵滴定数3", "启用1", "启用2", "启用3", "浓度4", "浓度5", "泵滴定数4", "泵滴定数5", "启用4", "启用5", "标液校准时间1", "标液校准时间2", "标液校准时间3", "标液校准时间4", "零点校准时间": Value Change {
        n855 = event-data() -> ()  [unwired: 1 in, 6 out]
        n856 = local read "选用水样"() -> (w1482:enum16{"葡萄糖", "草酸钠"})
        n857 = local read "量程选择"() -> (w1481:enum16{"低量程", "高量程"})
        n858 = case shown="\"葡萄糖\", 默认" w1482 {
          tunnel: ["葡萄糖标线" ("section") "草酸钠标线" ("section")] -> w1486
          frame "葡萄糖", Default {
          }
          frame "草酸钠" {
          }
        }
        n859 = case shown="\"高量程\"" w1481 {
          tunnel: ["低量程" "高量程"] -> w1480
          frame "低量程", Default {
          }
          frame "高量程" {
          }
        }
        n860 = global read "CODMN外部API.vi" "ping"() -> (w1467:bool)
        n861 = case shown="假" w1467 {
          tunnel: [w1564 w1567] -> w1466
          frame False {
            n862 = global read "COD内部交互全局.vi" "配置文件ini"() -> (w1566:string)
            n863 = call <vilib>:"Application Directory.vi"() -> ("Application Directory"=w1565:path)
            n864 = Build Path(base path=w1565, name or relative path=w1566) -> (appended path=w1564:path)
          }
          frame True {
            n865 = global read "CODMN外部API.vi" "配置文件 path"() -> (w1567:path)
          }
        }
        n866 = Concatenate Strings(w1486, w1480) -> (w1444:string)
        n867 = call <vilib>:"Open Config Data.vi"("configuration file path"=w1466) -> ("error out"=w1535:errorcluster, "refnum"=w1536:T6)  [unwired: 8 in, 1 out]
        n868 = local read "模型"() -> (w1431:enum32{"线性", "多项式", "折线"})
        n869 = case shown="\"折线\"" w1431 {
          tunnel: [9999.0 ("泵滴定数5") 9999.0 ("泵滴定数5") w1539] -> w1430
          frame "线性", Default {
          }
          frame "多项式" {
          }
          frame "折线" {
            n870 = local read "泵滴定数5"() -> (w1546:dbl)
            n871 = local read "泵滴定数3"() -> (w1548:dbl)
            n872 = local read "泵滴定数2"() -> (w1549:dbl)
            n873 = local read "泵滴定数4"() -> (w1547:dbl)
            n874 = local read "泵滴定数1"() -> (w1550:dbl)
            n875 = Build Array(w1550, w1549, w1548, w1547, w1546) -> (w1545:dbl[])
            n876 = local read "启用5"() -> (w1551:bool)
            n877 = local read "启用1"() -> (w1555:bool)
            n878 = local read "启用2"() -> (w1554:bool)
            n879 = local read "启用3"() -> (w1553:bool)
            n880 = local read "启用4"() -> (w1552:bool)
            n881 = Build Array(w1555, w1554, w1553, w1552, w1551) -> (w1544:bool[])
            n882 = for {
              tunnel: w1545 -> [w1558] mode=indexing
              tunnel: w1544 -> [w1559] mode=indexing
              shift-right: [w1557] -> w1542
              shift-left: dbl[] [] -> [w1556]
              n883 = case shown="假" w1559 {
                tunnel: w1558 -> [_ w1563]
                tunnel: w1556 -> [w1560 w1562]
                tunnel: [w1560 w1561] -> w1557
                frame False {
                }
                frame True {
                  n884 = Build Array (concatenate)(w1562, w1563) -> (w1561:dbl[])
                }
              }
            }
            n885 = Sort 1D Array(array=w1542) -> (sorted array=w1541:dbl[])
            n886 = Index Array(array=w1541, index=1 ("索引")) -> (element=w1539:dbl)
          }
        }
        n887 = local read "浓度1"() -> (w1533:dbl)
        n888 = call-poly <vilib>:"Write Key.vi"("section"=w1444, "error in (no error)"=w1535, "value"=w1533, "key"="浓度1", "refnum"=w1536) -> ("error out"=w1532:errorcluster, "refnum out"=w1531:T6)  [unwired: 4 in, 1 out]
        n889 = local read "浓度2"() -> (w1517:dbl)
        n890 = call-poly <vilib>:"Write Key.vi"("section"=w1444, "error in (no error)"=w1532, "value"=w1517, "key"="浓度2", "refnum"=w1531) -> ("error out"=w1530:errorcluster, "refnum out"=w1529:T6)  [unwired: 4 in, 1 out]
        n891 = local read "浓度3"() -> (w1513:dbl)
        n892 = local read "泵滴定数1"() -> (w1511:dbl)
        n893 = call-poly <vilib>:"Write Key.vi"("section"=w1444, "error in (no error)"=w1530, "value"=w1513, "key"="浓度3", "refnum"=w1529) -> ("error out"=w1528:errorcluster, "refnum out"=w1527:T6)  [unwired: 4 in, 1 out]
        n894 = local read "泵滴定数2"() -> (w1509:dbl)
        n895 = call-poly <vilib>:"Write Key.vi"("section"=w1444, "error in (no error)"=w1528, "value"=w1511, "key"="泵滴定数1", "refnum"=w1527) -> ("error out"=w1526:errorcluster, "refnum out"=w1525:T6)  [unwired: 4 in, 1 out]
        n896 = local read "泵滴定数3"() -> (w1507:dbl)
        n897 = call-poly <vilib>:"Write Key.vi"("section"=w1444, "error in (no error)"=w1526, "value"=w1509, "key"="泵滴定数2", "refnum"=w1525) -> ("error out"=w1524:errorcluster, "refnum out"=w1523:T6)  [unwired: 4 in, 1 out]
        n898 = call-poly <vilib>:"Write Key.vi"("section"=w1444, "error in (no error)"=w1524, "value"=w1507, "key"="泵滴定数3", "refnum"=w1523) -> ("error out"=w1522:errorcluster, "refnum out"=w1521:T6)  [unwired: 4 in, 1 out]
        n899 = local read "浓度4"() -> (w1479:dbl)
        n900 = local write "公式切换阈值滴定数(0-9999)"(w1430) -> ()
        n901 = call-poly <vilib>:"Write Key.vi"("section"=w1444, "error in (no error)"=w1522, "value"=w1479, "key"="浓度4", "refnum"=w1521) -> ("error out"=w1515:errorcluster, "refnum out"=w1516:T6)  [unwired: 4 in, 1 out]
        n902 = local read "浓度5"() -> (w1478:dbl)
        n903 = local read "泵滴定数4"() -> (w1475:dbl)
        n904 = call-poly <vilib>:"Write Key.vi"("section"=w1444, "error in (no error)"=w1515, "value"=w1478, "key"="浓度5", "refnum"=w1516) -> ("error out"=w1476:errorcluster, "refnum out"=w1477:T6)  [unwired: 4 in, 1 out]
        n905 = local read "泵滴定数5"() -> (w1474:dbl)
        n906 = call-poly <vilib>:"Write Key.vi"("section"=w1444, "error in (no error)"=w1476, "value"=w1475, "key"="泵滴定数4", "refnum"=w1477) -> ("error out"=w1520:errorcluster, "refnum out"=w1519:T6)  [unwired: 4 in, 1 out]
        n907 = local read "零点校准时间"() -> (w1441:timestamp)
        n908 = call-poly <vilib>:"Write Key.vi"("section"=w1444, "error in (no error)"=w1520, "value"=w1474, "key"="泵滴定数5", "refnum"=w1519) -> ("error out"=w1472:errorcluster, "refnum out"=w1473:T6)  [unwired: 4 in, 1 out]
        n909 = local read "启用1"() -> (w1495:bool)
        n910 = local read "标液校准时间1"() -> (w1439:timestamp)
        n911 = Flatten To String(anything=w1441) -> (data string=w1440:string)  [unwired: 3 in, 2 out]
        n912 = call-poly <vilib>:"Write Key.vi"("section"=w1444, "error in (no error)"=w1472, "value"=w1495, "key"="启用1", "refnum"=w1473) -> ("error out"=w1491:errorcluster, "refnum out"=w1494:T6)  [unwired: 4 in, 1 out]
        n913 = Flatten To String(anything=w1439) -> (data string=w1438:string)  [unwired: 3 in, 2 out]
        n914 = local read "启用2"() -> (w1492:bool)
        n915 = local read "标液校准时间2"() -> (w1436:timestamp)
        n916 = call-poly <vilib>:"Write Key.vi"("section"=w1444, "error in (no error)"=w1491, "value"=w1492, "key"="启用2", "refnum"=w1494) -> ("error out"=w1502:errorcluster, "refnum out"=w1501:T6)  [unwired: 4 in, 1 out]
        n917 = Flatten To String(anything=w1436) -> (data string=w1437:string)  [unwired: 3 in, 2 out]
        n918 = local read "启用3"() -> (w1490:bool)
        n919 = local read "标液校准时间3"() -> (w1433:timestamp)
        n920 = call-poly <vilib>:"Write Key.vi"("section"=w1444, "error in (no error)"=w1502, "value"=w1490, "key"="启用3", "refnum"=w1501) -> ("error out"=w1500:errorcluster, "refnum out"=w1499:T6)  [unwired: 4 in, 1 out]
        n921 = local read "启用4"() -> (w1468:bool)
        n922 = Flatten To String(anything=w1433) -> (data string=w1432:string)  [unwired: 3 in, 2 out]
        n923 = call-poly <vilib>:"Write Key.vi"("section"=w1444, "error in (no error)"=w1500, "value"=w1468, "key"="启用4", "refnum"=w1499) -> ("error out"=w1498:errorcluster, "refnum out"=w1497:T6)  [unwired: 4 in, 1 out]
        n924 = local read "标液校准时间4"() -> (w1435:timestamp)
        n925 = local read "启用5"() -> (w1469:bool)
        n926 = Flatten To String(anything=w1435) -> (data string=w1434:string)  [unwired: 3 in, 2 out]
        n927 = local read "选用水样"() -> (w1485:enum16{"葡萄糖", "草酸钠"})
        n928 = call-poly <vilib>:"Write Key.vi"("section"=w1444, "error in (no error)"=w1498, "value"=w1469, "key"="启用5", "refnum"=w1497) -> ("error out"=w1470:errorcluster, "refnum out"=w1471:T6)  [unwired: 4 in, 1 out]
        n929 = call-poly <vilib>:"Write Key.vi"("section"="标线选择", "error in (no error)"=w1470, "value"=w1485, "key"="选用水样", "refnum"=w1471) -> ("error out"=w1450:errorcluster, "refnum out"=w1451:T6)  [unwired: 4 in, 1 out]
        n930 = call-poly <vilib>:"Write Key.vi"("section"=w1444, "error in (no error)"=w1450, "value"=w1440, "key"="零点校准时间", "refnum"=w1451) -> ("error out"=w1458:errorcluster, "refnum out"=w1457:T6)  [unwired: 4 in, 1 out]
        n931 = call-poly <vilib>:"Write Key.vi"("section"=w1444, "error in (no error)"=w1458, "value"=w1438, "key"="标液1校准时间", "refnum"=w1457) -> ("error out"=w1453:errorcluster, "refnum out"=w1446:T6)  [unwired: 4 in, 1 out]
        n932 = call-poly <vilib>:"Write Key.vi"("section"=w1444, "error in (no error)"=w1453, "value"=w1437, "key"="标液2校准时间", "refnum"=w1446) -> ("error out"=w1454:errorcluster, "refnum out"=w1443:T6)  [unwired: 4 in, 1 out]
        n933 = call-poly <vilib>:"Write Key.vi"("section"=w1444, "error in (no error)"=w1454, "value"=w1432, "key"="标液3校准时间", "refnum"=w1443) -> ("error out"=w1455:errorcluster, "refnum out"=w1456:T6)  [unwired: 4 in, 1 out]
        n934 = call-poly <vilib>:"Write Key.vi"("section"=w1444, "error in (no error)"=w1455, "value"=w1434, "key"="标液4校准时间", "refnum"=w1456) -> ("error out"=w1448:errorcluster, "refnum out"=w1449:T6)  [unwired: 4 in, 1 out]
        n935 = call <vilib>:"Close Config Data.vi"("error in (no error)"=w1448, "refnum"=w1449) -> ("error out"=w1460:errorcluster, "file path"=w1461:path)  [unwired: 8 in]
        n936 = Open/Create/Replace File(file path (use dialog)=w1461, error in=w1460) -> (refnum out=w1463:refnum<file>, error out=w1462:errorcluster)  [unwired: 4 in, 1 out]
        n937 = Flush File(refnum=w1463, error in=w1462) -> (refnum out=w1464:refnum<file>, error out=w1465:errorcluster)
        n938 = Close File(refnum=w1464, error in=w1465) -> ()  [unwired: 2 out]
      }
      event "读取": Value Change {
        (unwired) u16 94 ("number of holding registers")
        (unwired) u16 4616 ("starting address")
        n939 = event-data() -> ()  [unwired: 1 in, 6 out]
        n940 = Bundle By Name(cluster=cluster{"命令":string} {"命令"=""} ("元素"), "命令"="CODMn读取公式" ("名称（未命名）")) -> (w1572:cluster{"命令":string})
        n941 = Enqueue Element(queue=w1576, element=w1572, error in (no error)=w1575) -> ()  [unwired: 1 in, 3 out]
      }
      event "写入": Mouse Down {
        n942 = event-data() -> ()  [unwired: 1 in, 8 out]
        n943 = Two Button Dialog(message="即将将左侧拟合公式写入仪器当前量程\n请选择是否写入？" ("消息"), 2:"确定" ("T按钮名称（“确定”）")) -> (T button?=w1577:bool)  [unwired: 1 in]
        n944 = case shown="真" w1577 {
          frame True {
            n945 = local read "量程选择"() -> (w1583:enum16{"低量程", "高量程"})
            n946 = local read "公式切换阈值滴定数(0-9999)"() -> (w1582:u16)
            n947 = Cluster To Array(cluster="方程系数") -> (array=w1586:dbl[])
            "公式系数" <- w1586
            n948 = local read "模型"() -> (w1584:enum32{"线性", "多项式", "折线"})
            n949 = call "公式写入.vi"("公式 2"="方程系数 2", "公式切换阈值滴定数(0-9999)"=w1582, "公式"="方程系数", "量程选择"=w1583, "模型"=w1584) -> ("error out"=w1585:errorcluster)  [unwired: 6 in]
            n950 = Index Array(array=w1586) -> (element #1=w1589:dbl, element #2=w1587:dbl, element #3=w1588:dbl)  [unwired: 3 in]
            n951 = case shown="无错误" w1585 {
              tunnel: ["写入成功！" "写入失败！"] -> w1590
              tunnel: w1587 -> [w1594 _]
              tunnel: w1589 -> [w1595 _]
              tunnel: w1588 -> [w1596 _]
              tunnel: w1583 -> [_ _]
              frame No Error {
                n952 = Number To Fractional String(number=w1594) -> (F-format string=w1598:string)  [unwired: 3 in]
                n953 = Number To Fractional String(number=w1595) -> (F-format string=w1599:string)  [unwired: 3 in]
                n954 = Number To Fractional String(number=w1596) -> (F-format string=w1597:string)  [unwired: 3 in]
                n955 = property on="模型" class="Enum (严格)"() -> ("RingText.Text"=w1591:string)  [unwired: 2 in, 2 out]
                n956 = property on="量程选择" class="Enum (严格)"() -> ("RingText.Text"=w1607:string)  [unwired: 2 in, 2 out]
                n957 = Concatenate Strings("变更后:" ("table输入"), "K:" ("字符串"), w1599, "B:" ("字符串"), w1598, "X^2:" ("字符串"), w1597) -> (w1600:string)
                n958 = Concatenate Strings(w1591, w1607, "公式改变" ("日志信息")) -> (w1601:string)
                n959 = local write "存校准信息"(TRUE ("存校准信息")) -> ()
                n960 = Get Date/Time In Seconds() -> (seconds since 1Jan1904=w1610:timestamp)
                n961 = Bundle(cluster=T17 {"时间标识"=timestamp(0 s since 1904-01-01), "参数"="", "日志信息"="", "流程参数"=""} ("data in"), "时间标识"=w1610, "参数"="CODMn" ("table输入"), "日志信息"=w1601, "流程参数"=w1600) -> (w1593:T17)
                n962 = call "流程日志字段定义.vi"("table输入"="操作日志", "data in"=w1593) -> ("table输出"=w1613:string, "columns"=w1614:string[], "data out"=w1615:T19)  [unwired: 7 in]
                n963 = call "插入数据.vi"("data"=w1615, "columns"=w1614, "database"="database3.mdb", "table"=w1613) -> ()  [unwired: 7 in, 1 out]
              }
              frame Error {
              }
            }
            n964 = One Button Dialog(message=w1590) -> ()  [unwired: 1 in, 1 out]
          }
          frame False {
          }
        }
      }
      event "滴定曲线", "温度曲线": Value Change {
        n965 = event-data() -> ("CtlRef"=w1619:refnum<vi>)  [unwired: 1 in, 5 out]
        n966 = property class="Bool"(reference=w1619) -> ("Label.Text"=w1618:string)  [unwired: 1 in, 2 out]
        n967 = case shown="\"温度曲线\", 默认" w1618 {
          tunnel: [T4 {"Horizontal"=0, "Vertical"=4000} ("原点") T4 {"Horizontal"=0, "Vertical"=3200} ("原点")] -> w1620
          frame "温度曲线", Default {
          }
          frame "滴定曲线" {
          }
        }
        n968 = property on="窗格" class="Pane"("Origin"=w1620) -> ()  [unwired: 2 in, 2 out]
      }
      event "历史波形", "历史波形 2": Value Change {
        n969 = event-data() -> ("CtlRef"=w1624:refnum<vi>)  [unwired: 1 in, 5 out]
        n970 = property class="Bool (严格)"(reference=w1624) -> ("Label.Text"=w1623:string)  [unwired: 1 in, 2 out]
        n971 = case shown="\"历史波形2\"" w1623 {
          frame "历史波形2" {
            n972 = call-poly <vilib>:"Read Waveforms from File.vi"() -> ("error out"=w1625:errorcluster, "first waveform in record"=w1626:waveform(dbl))  [unwired: 6 in, 2 out]
            n973 = case shown="无错误" w1625 {
              tunnel: w1626 -> [w1629 _]
              frame No Error {
                n974 = Unbundle By Name(w1629) -> ("t0"=w1627:timestamp, "Y"=w1628:dbl[])  [unwired: 2 out]
                n975 = global write "COD内部交互全局.vi" "温度波形时间"(w1627) -> ()
                n976 = global write "COD内部交互全局.vi" "时间温度曲线"(w1628) -> ()
                n977 = global write "COD内部交互全局.vi" "时间-温度"(w1628) -> ()
              }
              frame Error {
                n978 = One Button Dialog(message="打开失败" ("消息")) -> ()  [unwired: 1 in, 1 out]
              }
            }
          }
          frame "历史波形", Default {
            n979 = call-poly <vilib>:"Read Waveforms from File.vi"() -> ("error out"=w1631:errorcluster, "first waveform in record"=w1632:waveform(dbl))  [unwired: 6 in, 2 out]
            n980 = case shown="无错误" w1631 {
              tunnel: w1632 -> [w1635 _]
              frame No Error {
                n981 = Unbundle By Name(w1635) -> ("t0"=w1633:timestamp, "Y"=w1634:dbl[])  [unwired: 2 out]
                n982 = global write "COD内部交互全局.vi" "波形时间"(w1633) -> ()
                n983 = global write "COD内部交互全局.vi" "ORP滴定曲线"(w1634) -> ()
                n984 = global write "COD内部交互全局.vi" "滴定数-ORP值"(w1634) -> ()
              }
              frame Error {
                n985 = One Button Dialog(message="打开失败" ("消息")) -> ()  [unwired: 1 in, 1 out]
              }
            }
          }
        }
      }
      event "释放串口": Value Change {
        n986 = event-data() -> ()  [unwired: 1 in, 6 out]
        n987 = Two Button Dialog(message="确认是否释放串口，释放串口将导致通信失败！" ("消息")) -> (T button?=w1637:bool)  [unwired: 2 in]
        n988 = case shown="真" w1637 {
          tunnel: w1640 -> [_ w1642]
          tunnel: w1639 -> [_ w1641]
          frame False {
          }
          frame True {
            n989 = Bundle By Name(cluster=cluster{"命令":string} {"命令"=""} ("元素"), "命令"="停用模块" ("名称（未命名）")) -> (w1643:cluster{"命令":string})
            n990 = Enqueue Element(queue=w1642, element=w1643, error in (no error)=w1641) -> ()  [unwired: 1 in, 3 out]
          }
        }
      }
      event "打开串口": Value Change {
        n991 = event-data() -> ()  [unwired: 1 in, 6 out]
        n992 = flat-sequence {
          tunnel: w1647 -> [w1655]
          tunnel: w1646 -> [w1654]
          frame #0 {
            n993 = global read "CODMn断电保存全局变量.vi" "VISA resource name"() -> (w1658:refnum<visa-resource-name>)
            n994 = global read "CODMn断电保存全局变量.vi" "MB通信方式选择"() -> (w1651:enum16{"串口", "TCP"})
            n995 = global read "CODMn断电保存全局变量.vi" "PORT"() -> (w1649:string)
            n996 = global read "CODMn断电保存全局变量.vi" "IP"() -> (w1650:string)
            n997 = call "串口配置.vi"("PORT"=w1649, "IP"=w1650, "MB通信方式选择"=w1651, "请选择串口:"=w1658) -> ("PORT 2"=w1652:string, "IP 2"=w1653:string, "确认 2"=w1656:bool, "VISA资源名称 2"=w1657:refnum<visa-resource-name>, "MB通信方式选择 2"=w1648:enum16{"串口", "TCP"})  [unwired: 3 in]
            n998 = case shown="真" w1656 {
              tunnel: w1657 -> [_ w1667]
              tunnel: w1655 -> [_ w1663]
              tunnel: w1654 -> [_ w1662]
              tunnel: w1653 -> [_ w1661]
              tunnel: w1652 -> [_ w1660]
              tunnel: w1648 -> [_ w1659]
              frame False {
              }
              frame True {
                n999 = global write "CODMn断电保存全局变量.vi" "IP"(w1661) -> ()
                n1000 = global write "CODMn断电保存全局变量.vi" "PORT"(w1660) -> ()
                n1001 = global write "CODMn断电保存全局变量.vi" "VISA resource name"(w1667) -> ()
                n1002 = global write "CODMn断电保存全局变量.vi" "MB通信方式选择"(w1659) -> ()
                n1003 = Bundle By Name(cluster=cluster{"命令":string} {"命令"=""} ("元素"), "命令"="启用模块" ("名称（未命名）")) -> (w1664:cluster{"命令":string})
                n1004 = Enqueue Element(queue=w1663, element=w1664, error in (no error)=w1662) -> ()  [unwired: 1 in, 3 out]
              }
            }
          }
          frame #1 {
            n1005 = call "配置文件保存.vi"() -> ()  [unwired: 12 in]
          }
        }
      }
      event "更新程序": Value Change {
        n1006 = event-data() -> ("CtlRef"=w1670:refnum<vi>, "NewVal"=w1671:bool)  [unwired: 1 in, 4 out]
        n1007 = case shown="真" w1671 {
          tunnel: w1670 -> [_ w1680]
          tunnel: w1669 -> [w1673 w1679]
          tunnel: w1668 -> [w1672 w1678]
          frame False {
            n1008 = Bundle By Name(cluster=cluster{"命令":string} {"命令"=""} ("元素"), "命令"="启用模块" ("名称（未命名）")) -> (w1674:cluster{"命令":string})
            n1009 = Enqueue Element(queue=w1673, element=w1674, error in (no error)=w1672) -> ()  [unwired: 1 in, 3 out]
          }
          frame True {
            n1010 = Two Button Dialog(message="警告，非专业人士请勿进行此操作！！！\n请确认是否继续？" ("消息")) -> (T button?=w1682:bool)  [unwired: 2 in]
            n1011 = case shown="真" w1682 {
              tunnel: w1680 -> [w1698 _]
              tunnel: w1679 -> [_ w1706]
              tunnel: w1678 -> [_ w1705]
              tunnel: [errorcluster {"status"=TRUE, "code"=0, "source"=""} ("error out") w1699] -> w1677
              frame False {
                n1012 = property class="Bool (严格)"(reference=w1698, "Value"=FALSE ("释放串口")) -> ()  [unwired: 1 in, 2 out]
              }
              frame True {
                n1013 = Bundle By Name(cluster=cluster{"命令":string} {"命令"=""} ("元素"), "命令"="CODMn程序更新" ("名称（未命名）")) -> (w1709:cluster{"命令":string})
                n1014 = Enqueue Element(queue=w1706, element=w1709, error in (no error)=w1705) -> (queue out=w1704:refnum<queue>, error out=w1703:errorcluster)  [unwired: 1 in, 1 out]
                n1015 = Bundle By Name(cluster=cluster{"命令":string} {"命令"=""} ("元素"), "命令"="停用模块" ("名称（未命名）")) -> (w1700:cluster{"命令":string})
                n1016 = Enqueue Element(queue=w1704, element=w1700, error in (no error)=w1703) -> (error out=w1699:errorcluster)  [unwired: 1 in, 2 out]
              }
            }
            n1017 = case shown="无错误" w1677 {
              frame No Error {
                n1018 = call "文件对话框"("start path"=path "D:/SRC") -> ("selected path"=w1685:path, "cancelled"=w1683:bool)  [unwired: 11 in, 2 out]
                n1019 = case shown="假" w1683 {
                  tunnel: w1685 -> [w1690 _]
                  frame False {
                    n1020 = Path To String(path=w1690) -> (string=w1687:string)
                    n1021 = Format Into String(format string="  - \"%s\"" ("格式字符串"), initial string="\"C:\\Program Files\\Fatek\\WinProladder\\WProlad.exe\"" ("command line"), w1687) -> (resulting string=w1688:string)  [unwired: 1 in, 1 out]
                    n1022 = call <vilib>:"System Exec.vi"("command line"=w1688) -> ("error out"=w1691:errorcluster)  [unwired: 7 in, 3 out]
                    n1023 = case shown="错误" w1691 {
                      tunnel: w1687 -> [_ w1694]
                      frame No Error {
                      }
                      frame Error {
                        n1024 = Format Into String(format string="  - \"%s\"" ("格式字符串"), initial string="\"C:\\Program Files (x86)\\Fatek\\WinProladder\\WProlad.exe\"" ("command line"), w1694) -> (resulting string=w1692:string)  [unwired: 1 in, 1 out]
                        n1025 = call <vilib>:"System Exec.vi"("command line"=w1692) -> ()  [unwired: 7 in, 4 out]
                      }
                    }
                  }
                  frame True {
                  }
                }
              }
              frame Error {
              }
            }
          }
        }
      }
      event "序列号变更": Value Change {
        n1026 = event-data() -> ()  [unwired: 1 in, 6 out]
        n1027 = local read "CODMn序列号"() -> (w1713:string)
        n1028 = call "序列号写入.vi"("序列号:"=w1713) -> ("确认 2"=w1710:bool, "序列号输出"=w1714:string)  [unwired: 9 in]
        n1029 = case shown="真" w1710 {
          tunnel: w1714 -> [_ w1720]
          tunnel: w1712 -> [_ w1716]
          tunnel: w1711 -> [_ w1715]
          frame False {
          }
          frame True {
            n1030 = global write "COD内部交互全局.vi" "序列号:"(w1720) -> ()
            n1031 = Bundle By Name(cluster=cluster{"命令":string} {"命令"=""} ("元素"), "命令"="CODMn序列号写入" ("名称（未命名）")) -> (w1717:cluster{"命令":string})
            n1032 = Enqueue Element(queue=w1716, element=w1717, error in (no error)=w1715) -> ()  [unwired: 1 in, 3 out]
          }
        }
      }
      event Timeout {
        n1033 = event-data() -> ()  [unwired: 1 in, 3 out]
      }
    }
  }
  n1034 = while {
    stop <- FALSE stop-if-true
    # "数字键盘输入"
    n1035 = event shown="[29] \"公式切换阈值滴定数(0-9999)\": 鼠标按下" {
      selector: _ -> [_ _ _ _ _ _ _ _ _ _ _ _ _ _ _ _ _ _ _ _ _ _ _ _ _ _ _ _ _ _ _]
      dyn-events: _ -> [_ _ _ _ _ _ _ _ _ _ _ _ _ _ _ _ _ _ _ _ _ _ _ _ _ _ _ _ _ _ _]
      timeout: _ -> [_ _ _ _ _ _ _ _ _ _ _ _ _ _ _ _ _ _ _ _ _ _ _ _ _ _ _ _ _ _ _]
      event Timeout {
        n1036 = event-data() -> ()  [unwired: 1 in, 3 out]
      }
      event "温度": Mouse Down {
        n1037 = event-data() -> ()  [unwired: 1 in, 8 out]
        n1038 = local read "温度"() -> (w1723:dbl)
        n1039 = call "数字键盘.vi"("OldNumber"=w1723) -> ("NewNumber"=w1722:sgl)
        n1040 = local write "温度"(w1722) -> ()
      }
      event "恒温时间": Mouse Down {
        n1041 = event-data() -> ()  [unwired: 1 in, 8 out]
        n1042 = local read "恒温时间"() -> (w1724:dbl)
        n1043 = call "数字键盘.vi"("OldNumber"=w1724) -> ("NewNumber"=w1725:sgl)
        n1044 = local write "恒温时间"(w1725) -> ()
      }
      event "标准液浓度": Mouse Down {
        n1045 = event-data() -> ()  [unwired: 1 in, 8 out]
        n1046 = local read "标准液浓度"() -> (w1727:dbl)
        n1047 = call "数字键盘.vi"("OldNumber"=w1727) -> ("NewNumber"=w1726:sgl)
        n1048 = local write "标准液浓度"(w1726) -> ()
      }
      event "氢氧化钠：": Mouse Down {
        n1049 = event-data() -> ()  [unwired: 1 in, 8 out]
        n1050 = local read "氢氧化钠："() -> (w1728:dbl)
        n1051 = call "数字键盘.vi"("OldNumber"=w1728) -> ("NewNumber"=w1729:sgl)
        n1052 = local write "氢氧化钠："(w1729) -> ()
      }
      event "水样：": Mouse Down {
        n1053 = event-data() -> ()  [unwired: 1 in, 8 out]
        n1054 = local read "水样："() -> (w1730:dbl)
        n1055 = call "数字键盘.vi"("OldNumber"=w1730) -> ("NewNumber"=w1731:sgl)
        n1056 = local write "水样："(w1731) -> ()
      }
      event "蒸馏水：": Mouse Down {
        n1057 = event-data() -> ()  [unwired: 1 in, 8 out]
        n1058 = local read "蒸馏水："() -> (w1732:dbl)
        n1059 = call "数字键盘.vi"("OldNumber"=w1732) -> ("NewNumber"=w1733:sgl)
        n1060 = local write "蒸馏水："(w1733) -> ()
      }
      event "标液：": Mouse Down {
        n1061 = event-data() -> ()  [unwired: 1 in, 8 out]
        n1062 = local read "标液："() -> (w1734:dbl)
        n1063 = call "数字键盘.vi"("OldNumber"=w1734) -> ("NewNumber"=w1735:sgl)
        n1064 = local write "标液："(w1735) -> ()
      }
      event "零点核查样：": Mouse Down {
        n1065 = event-data() -> ()  [unwired: 1 in, 8 out]
        n1066 = local read "零点核查样："() -> (w1736:dbl)
        n1067 = call "数字键盘.vi"("OldNumber"=w1736) -> ("NewNumber"=w1737:sgl)
        n1068 = local write "零点核查样："(w1737) -> ()
      }
      event "加标回收样：": Mouse Down {
        n1069 = event-data() -> ()  [unwired: 1 in, 8 out]
        n1070 = local read "加标回收样："() -> (w1738:dbl)
        n1071 = call "数字键盘.vi"("OldNumber"=w1738) -> ("NewNumber"=w1739:sgl)
        n1072 = local write "加标回收样："(w1739) -> ()
      }
      event "草酸钠": Mouse Down {
        n1073 = event-data() -> ()  [unwired: 1 in, 8 out]
        n1074 = local read "草酸钠"() -> (w1740:dbl)
        n1075 = call "数字键盘.vi"("OldNumber"=w1740) -> ("NewNumber"=w1741:sgl)
        n1076 = local write "草酸钠"(w1741) -> ()
      }
      event "高锰酸钾": Mouse Down {
        n1077 = event-data() -> ()  [unwired: 1 in, 8 out]
        n1078 = local read "高锰酸钾"() -> (w1742:dbl)
        n1079 = call "数字键盘.vi"("OldNumber"=w1742) -> ("NewNumber"=w1743:sgl)
        n1080 = local write "高锰酸钾"(w1743) -> ()
      }
      event "硫酸": Mouse Down {
        n1081 = event-data() -> ()  [unwired: 1 in, 8 out]
        n1082 = local read "硫酸"() -> (w1744:dbl)
        n1083 = call "数字键盘.vi"("OldNumber"=w1744) -> ("NewNumber"=w1745:sgl)
        n1084 = local write "硫酸"(w1745) -> ()
      }
      event "零点泵计量数 2": Mouse Down {
        n1085 = event-data() -> ()  [unwired: 1 in, 8 out]
        n1086 = local read "零点泵计量数 2"() -> (w1746:dbl)
        n1087 = call "数字键盘.vi"("OldNumber"=w1746) -> ("NewNumber"=w1747:sgl)
        n1088 = local write "零点泵计量数 2"(w1747) -> ()
      }
      event "标度泵计量数 2": Mouse Down {
        n1089 = event-data() -> ()  [unwired: 1 in, 8 out]
        n1090 = local read "标度泵计量数 2"() -> (w1748:dbl)
        n1091 = call "数字键盘.vi"("OldNumber"=w1748) -> ("NewNumber"=w1749:sgl)
        n1092 = local write "标度泵计量数 2"(w1749) -> ()
      }
      event "高量程稀释倍数:": Mouse Down {
        n1093 = event-data() -> ()  [unwired: 1 in, 8 out]
        n1094 = local read "高量程稀释倍数:"() -> (w1751:i8)
        n1095 = call "数字键盘.vi"("OldNumber"=w1751) -> ("NewNumber"=w1750:sgl)
        n1096 = local write "高量程稀释倍数:"(w1750) -> ()
      }
      event "低量程稀释倍数:": Mouse Down {
        n1097 = event-data() -> ()  [unwired: 1 in, 8 out]
        n1098 = local read "低量程稀释倍数:"() -> (w1753:i8)
        n1099 = call "数字键盘.vi"("OldNumber"=w1753) -> ("NewNumber"=w1752:sgl)
        n1100 = local write "低量程稀释倍数:"(w1752) -> ()
      }
      event "浓度1": Mouse Down {
        n1101 = event-data() -> ()  [unwired: 1 in, 8 out]
        n1102 = local read "浓度1"() -> (w1755:dbl)
        n1103 = call "数字键盘.vi"("OldNumber"=w1755) -> ("NewNumber"=w1754:sgl)
        n1104 = property on="浓度1" class="DigNum (严格)"("Val(Sgnl)"=w1754) -> ()  [unwired: 2 in, 2 out]
      }
      event "浓度2": Mouse Down {
        n1105 = event-data() -> ()  [unwired: 1 in, 8 out]
        n1106 = local read "浓度2"() -> (w1757:dbl)
        n1107 = call "数字键盘.vi"("OldNumber"=w1757) -> ("NewNumber"=w1756:sgl)
        n1108 = property on="浓度2" class="DigNum (严格)"("Val(Sgnl)"=w1756) -> ()  [unwired: 2 in, 2 out]
      }
      event "浓度3": Mouse Down {
        n1109 = event-data() -> ()  [unwired: 1 in, 8 out]
        n1110 = local read "浓度3"() -> (w1759:dbl)
        n1111 = call "数字键盘.vi"("OldNumber"=w1759) -> ("NewNumber"=w1758:sgl)
        n1112 = property on="浓度3" class="DigNum (严格)"("Val(Sgnl)"=w1758) -> ()  [unwired: 2 in, 2 out]
      }
      event "浓度4": Mouse Down {
        n1113 = event-data() -> ()  [unwired: 1 in, 8 out]
        n1114 = local read "浓度4"() -> (w1761:dbl)
        n1115 = call "数字键盘.vi"("OldNumber"=w1761) -> ("NewNumber"=w1760:sgl)
        n1116 = property on="浓度4" class="DigNum (严格)"("Val(Sgnl)"=w1760) -> ()  [unwired: 2 in, 2 out]
      }
      event "浓度5": Mouse Down {
        n1117 = event-data() -> ()  [unwired: 1 in, 8 out]
        n1118 = local read "浓度5"() -> (w1763:dbl)
        n1119 = call "数字键盘.vi"("OldNumber"=w1763) -> ("NewNumber"=w1762:sgl)
        n1120 = property on="浓度5" class="DigNum (严格)"("Val(Sgnl)"=w1762) -> ()  [unwired: 2 in, 2 out]
      }
      event "跨度液浓度", "零点核查浓度", "标样浓度": Mouse Down {
        n1121 = event-data() -> ("CtlRef"=w1767:refnum<vi>)  [unwired: 1 in, 7 out]
        n1122 = property class="DigNum (严格)"(reference=w1767) -> (reference out=w1764:refnum<vi>, "Value"=w1766:dbl)  [unwired: 1 in, 1 out]
        n1123 = call "数字键盘.vi"("OldNumber"=w1766) -> ("NewNumber"=w1765:sgl)
        n1124 = property class="DigNum (严格)"(reference=w1764, "Val(Sgnl)"=w1765) -> ()  [unwired: 1 in, 2 out]
      }
      event "泵滴定数1": Mouse Down {
        n1125 = event-data() -> ()  [unwired: 1 in, 8 out]
        n1126 = local read "泵滴定数1"() -> (w1769:dbl)
        n1127 = call "数字键盘.vi"("OldNumber"=w1769) -> ("NewNumber"=w1768:sgl)
        n1128 = property on="泵滴定数1" class="DigNum (严格)"("Val(Sgnl)"=w1768) -> ()  [unwired: 2 in, 2 out]
      }
      event "泵滴定数2": Mouse Down {
        n1129 = event-data() -> ()  [unwired: 1 in, 8 out]
        n1130 = local read "泵滴定数2"() -> (w1771:dbl)
        n1131 = call "数字键盘.vi"("OldNumber"=w1771) -> ("NewNumber"=w1770:sgl)
        n1132 = property on="泵滴定数2" class="DigNum (严格)"("Val(Sgnl)"=w1770) -> ()  [unwired: 2 in, 2 out]
      }
      event "泵滴定数3": Mouse Down {
        n1133 = event-data() -> ()  [unwired: 1 in, 8 out]
        n1134 = local read "泵滴定数3"() -> (w1773:dbl)
        n1135 = call "数字键盘.vi"("OldNumber"=w1773) -> ("NewNumber"=w1772:sgl)
        n1136 = property on="泵滴定数3" class="DigNum (严格)"("Val(Sgnl)"=w1772) -> ()  [unwired: 2 in, 2 out]
      }
      event "泵滴定数4": Mouse Down {
        n1137 = event-data() -> ()  [unwired: 1 in, 8 out]
        n1138 = local read "泵滴定数4"() -> (w1775:dbl)
        n1139 = call "数字键盘.vi"("OldNumber"=w1775) -> ("NewNumber"=w1774:sgl)
        n1140 = property on="泵滴定数4" class="DigNum (严格)"("Val(Sgnl)"=w1774) -> ()  [unwired: 2 in, 2 out]
      }
      event "泵滴定数5": Mouse Down {
        n1141 = event-data() -> ()  [unwired: 1 in, 8 out]
        n1142 = local read "泵滴定数5"() -> (w1777:dbl)
        n1143 = call "数字键盘.vi"("OldNumber"=w1777) -> ("NewNumber"=w1776:sgl)
        n1144 = property on="泵滴定数5" class="DigNum (严格)"("Val(Sgnl)"=w1776) -> ()  [unwired: 2 in, 2 out]
      }
      event "低切高阈值:", "高切低阈值:": Mouse Down {
        n1145 = event-data() -> ("CtlRef"=w1781:refnum<vi>)  [unwired: 1 in, 7 out]
        n1146 = property class="DigNum (严格)"(reference=w1781) -> (reference out=w1780:refnum<vi>, "Value"=w1779:dbl)  [unwired: 1 in, 1 out]
        n1147 = call "数字键盘.vi"("OldNumber"=w1779) -> ("NewNumber"=w1778:sgl)
        n1148 = property class="DigNum (严格)"(reference=w1780, "Val(Sgnl)"=w1778) -> ()  [unwired: 1 in, 2 out]
      }
      event "公式切换阈值滴定数(0-9999)": Mouse Down {
        n1149 = event-data() -> ("CtlRef"=w1782:refnum<vi>)  [unwired: 1 in, 7 out]
        n1150 = property class="DigNum (严格)"(reference=w1782) -> (reference out=w1785:refnum<vi>, "Value"=w1784:u16)  [unwired: 1 in, 1 out]
        n1151 = call "数字键盘.vi"("OldNumber"=w1784) -> ("NewNumber"=w1783:sgl)
        n1152 = property class="DigNum (严格)"(reference=w1785, "Value"=w1783) -> ()  [unwired: 1 in, 2 out]
      }
      event "远程校准量程", "远程标样校准": Value Change {
        n1153 = event-data() -> ()  [unwired: 1 in, 6 out]
        n1154 = flat-sequence {
          frame #0 {
            n1155 = global write "CODMn断电保存全局变量.vi" "远程校准量程"("远程校准量程") -> ()
            n1156 = global write "CODMn断电保存全局变量.vi" "远程标样校准"("远程标样校准") -> ()
          }
          frame #1 {
            n1157 = call "配置文件保存.vi"() -> ()  [unwired: 12 in]
          }
        }
      }
    }
  }
  n1158 = while {
    stop <- FALSE stop-if-true
    # "滚动显示"
    n1159 = global read "COD内部交互全局.vi" "待机"() -> (w1788:bool)
    n1160 = case shown="假" w1788 {
      frame False {
        # "运行中"
        n1161 = global read "COD内部交互全局.vi" "校准内容显示"() -> (w1791:string)
        n1162 = while {
          shift-right: [w1793] -> _
          shift-left: w1791 -> [w1798]
          stop <- w1792 stop-if-true
          (unwired) "仪器校准中!\n当前校准浓度为:3mg/L" ("校准内容显示")
          n1163 = Wait (ms)(milliseconds to wait=u32 500 ("等待时间（毫秒）")) -> ()  [unwired: 1 out]
          n1164 = Spreadsheet String To Array(delimiter (Tab)="\n" ("分隔符(Tab)"), format string="" ("格式字符串"), spreadsheet string=w1798, array type (2D Dbl)=string[] []) -> (array=w1801:string[])
          n1165 = for {
            tunnel: w1801 -> [w1809] mode=indexing
            tunnel: [w1807] -> _ mode=indexing
            shift-right: [w1805] -> w1796
            shift-left: "" ("格式字符串") -> [w1806]
            n1166 = call "字符串移位显示.vi"("字符框大小"=36, "字符串输入"=w1809) -> ("移位后字符串"=w1807:string)  [unwired: 8 in, 1 out]
            n1167 = Concatenate Strings(w1806, w1807, "\n" ("分隔符(Tab)")) -> (w1805:string)
          }
          n1168 = String Length(string=w1796) -> (length=w1795:i32)
          n1169 = Decrement(x=w1795) -> (x-1=w1794:i32)
          n1170 = String Subset(string=w1796, length (rest)=w1794) -> (substring=w1793:string)  [unwired: 1 in]
          "校准内容显示" <- w1793
          n1171 = global read "COD内部交互全局.vi" "待机"() -> (w1792:bool)
        }
      }
      frame True {
      }
    }
    n1172 = Wait (ms)(milliseconds to wait=u32 1000 ("等待时间（毫秒）")) -> ()  [unwired: 1 out]
  }
  n1173 = property class="VI"(reference=w6, error in=w3) -> ("Name"=w7:string)  [unwired: 2 out]
  n1174 = while {
    stop <- FALSE stop-if-true
    # "相差60秒自动校时"
    n1175 = global read "运行时序全局变量.vi" "多列列表框"() -> (w1811:i32)
    n1176 = local read "仪器时间"() -> (w1818:timestamp)
    n1177 = local read "系统时间"() -> (w1819:timestamp)
    n1178 = Wait (ms)(milliseconds to wait=u32 1000 ("等待时间（毫秒）")) -> ()  [unwired: 1 out]
    n1179 = Build Array(w1818) -> (w1817:timestamp[])
    n1180 = Build Array(w1819) -> (w1836:timestamp[])
    n1181 = Equal?(x=w1811, y=u16 5) -> (x = y?=w1813:bool)
    n1182 = call <vilib>:"Boolean Crossing PtByPt.vi"("direction"=enum16{"either", "false-true", "true-false"}."false-true", "input"=w1813) -> ("crossing"=w1810:bool)  [unwired: 1 in]
    n1183 = call "DateToHex.vi"("DATE"=w1817) -> ("数组"=w1830:u16[])  [unwired: 10 in]
    n1184 = call "DateToHex.vi"("DATE"=w1836) -> ("数组"=w1835:u16[])  [unwired: 10 in]
    n1185 = case shown="真" w1810 {
      frame False {
      }
      frame True {
        # "校准结束后自动更新曲线泵滴定数"
        n1186 = global read "COD测量模式全局.vi" "测量模式文字实时"() -> (w1837:string)
        n1187 = global read "COD测量模式全局.vi" "测量模式文字实时"() -> (w1842:string)
        n1188 = global read "CODMN外部API.vi" "远程反控校准CODMn"() -> (w1841:bool)
        n1189 = global read "COD内部交互全局.vi" "高锰酸钾"() -> (w1845:dbl)
        n1190 = Equal?(x=w1837, y="校零") -> (x = y?=w1838:bool)
        n1191 = Equal?(x=w1842, y="校标") -> (x = y?=w1844:bool)
        n1192 = Or(x=w1838, y=w1844) -> (x .or. y?=w1840:bool)
        n1193 = case shown="真" w1840 {
          tunnel: w1845 -> [_ w1850]
          tunnel: w1837 -> [_ w1849]
          frame False {
          }
          frame True {
            w1858 = "量程选择" ("section")
            n1194 = global read "COD内部交互全局.vi" "数据存储时间戳"() -> (w1847:timestamp)
            n1195 = global read "CODMN外部API.vi" "ping"() -> (w1869:bool)
            n1196 = case shown="\"校零\"" w1849 {
              tunnel: ["标样校准时间：" "空白校准时间："] -> _
              frame "校标", Default {
              }
              frame "校零" {
              }
            }
            n1197 = case shown="假" w1869 {
              tunnel: [w1878 w1881] -> w1870
              frame False {
                n1198 = global read "COD内部交互全局.vi" "配置文件ini"() -> (w1880:string)
                n1199 = call <vilib>:"Application Directory.vi"() -> ("Application Directory"=w1879:path)
                n1200 = Build Path(base path=w1879, name or relative path=w1880) -> (appended path=w1878:path)
              }
              frame True {
                n1201 = global read "CODMN外部API.vi" "配置文件 path"() -> (w1881:path)
              }
            }
            n1202 = Format Date/Time String(time format string (%c)="%Y/%m/%d %H:%M:%S" ("时间格式字符串(%c)"), seconds (now)=w1847) -> ()  [unwired: 1 in, 1 out]
            n1203 = call <vilib>:"Open Config Data.vi"("configuration file path"=w1870) -> ("error out"=w1857:errorcluster, "refnum"=w1856:T6)  [unwired: 8 in, 1 out]
            n1204 = call-poly <vilib>:"Read Key.vi"("section"="标线选择", "error in (no error)"=w1857, "key"="选用水样", "refnum"=w1856) -> ("error out"=w1859:errorcluster, "value"=w1852:i32, "refnum out"=w1860:T6)  [unwired: 4 in, 1 out]
            n1205 = local write "选用水样"(w1852) -> ()
            n1206 = call-poly <vilib>:"Read Key.vi"("section"=w1858, "error in (no error)"=w1859, "key"=w1858, "refnum"=w1860) -> ("error out"=w1853:errorcluster, "value"=w1855:i32, "refnum out"=w1854:T6)  [unwired: 4 in, 1 out]
            n1207 = case shown="1" w1852 {
              tunnel: ["葡萄糖标线" ("section") "草酸钠标线" ("section")] -> w1867
              frame 0, Default {
              }
              frame 1 {
              }
            }
            n1208 = local write "量程选择"(w1855) -> ()
            n1209 = case shown="2" w1855 {
              tunnel: ["低量程" "高量程" "0-2量程"] -> w1866
              frame 0, Default {
              }
              frame 1 {
              }
              frame 2 {
              }
            }
            n1210 = Concatenate Strings(w1867, w1866) -> (w1868:string)
            n1211 = call-poly <vilib>:"Read Key.vi"("section"=w1868, "error in (no error)"=w1853, "key"="当前选用的校准" ("section"), "refnum"=w1854) -> ("error out"=w1865:errorcluster, "value"=w1848:i32, "refnum out"=w1864:T6)  [unwired: 4 in, 1 out]
            n1212 = case shown="5" w1848 {
              tunnel: w1847 -> [w1871 w1872 w1873 w1874 w1875]
              frame 1, Default {
                "零点校准时间" <- w1871
              }
              frame 2 {
                "标液校准时间1" <- w1872
              }
              frame 3 {
                "标液校准时间2" <- w1873
              }
              frame 4 {
                "标液校准时间3" <- w1874
              }
              frame 5 {
                "标液校准时间4" <- w1875
              }
            }
            n1213 = call <vilib>:"Close Config Data.vi"("error in (no error)"=w1865, "refnum"=w1864) -> ()  [unwired: 8 in, 2 out]
            n1214 = global write "COD内部交互全局.vi" "当前校准"(w1848) -> ()
            n1215 = case shown="5" w1848 {
              tunnel: w1850 -> [w1887 w1888 w1889 w1890 w1891]
              frame 1, Default {
                n1216 = property on="泵滴定数1" class="DigNum (严格)"("Val(Sgnl)"=w1887) -> ()  [unwired: 2 in, 2 out]
              }
              frame 2 {
                n1217 = property on="泵滴定数2" class="DigNum (严格)"("Val(Sgnl)"=w1888) -> ()  [unwired: 2 in, 2 out]
              }
              frame 3 {
                n1218 = property on="泵滴定数3" class="DigNum (严格)"("Val(Sgnl)"=w1889) -> ()  [unwired: 2 in, 2 out]
              }
              frame 4 {
                n1219 = property on="泵滴定数4" class="DigNum (严格)"("Val(Sgnl)"=w1890) -> ()  [unwired: 2 in, 2 out]
              }
              frame 5 {
                n1220 = property on="泵滴定数5" class="DigNum (严格)"("Val(Sgnl)"=w1891) -> ()  [unwired: 2 in, 2 out]
              }
            }
          }
        }
        n1221 = case shown="真" w1841 {
          frame False {
          }
          frame True {
            # "校准完自动写入公式"
            n1222 = global write "CODMN外部API.vi" "远程反控校准CODMn"(FALSE ("远程反控校准CODMn")) -> ()
          }
        }
      }
    }
    n1223 = Index Array(array=w1830, index=2 ("索引")) -> (element=w1832:u16)
    n1224 = Index Array(array=w1835, index=2 ("索引")) -> (element=w1833:u16)
    n1225 = Split Number(x=w1832) -> (hi(x)=w1826:u8)  [unwired: 1 out]
    n1226 = Split Number(x=w1833) -> (hi(x)=w1829:u8)  [unwired: 1 out]
    n1227 = To Byte Integer(number=w1826) -> (8bit integer=w1825:i8)
    n1228 = To Byte Integer(number=w1829) -> (8bit integer=w1828:i8)
    n1229 = Subtract(x=w1825, y=w1828) -> (x-y=w1827:i8)
    n1230 = Absolute Value(x=w1827) -> (abs(x)=w1824:i8)
    n1231 = local read "通讯状态"() -> (w1821:bool)
    n1232 = Greater Or Equal?(x=w1824, y=i8 5) -> (x >= y?=w1822:bool)
    n1233 = And(x=w1822, y=w1821) -> (x .and. y?=w1820:bool)
    n1234 = case shown="真" w1820 {
      frame False {
      }
      frame True {
        # "相差60秒时间自动校准"
        n1235 = flat-sequence {
          frame #0 {
            n1236 = property on="时间校准" class="Bool (严格)"("Val(Sgnl)"=TRUE ("值(信号)")) -> ()  [unwired: 2 in, 2 out]
          }
          frame #1 {
            n1237 = Wait (ms)(milliseconds to wait=u32 500 ("等待时间（毫秒）")) -> ()  [unwired: 1 out]
          }
          frame #2 {
            n1238 = property on="时间校准" class="Bool (严格)"("Val(Sgnl)"=FALSE ("值(信号)")) -> ()  [unwired: 2 in, 2 out]
          }
        }
      }
    }
  }
  n1239 = Open VI Reference(type specifier VI Refnum (for type only)=refnum<vi> refnum, vi path=w7, options=128 ("选项")) -> (vi reference=w9:refnum<vi>, error out=w11:errorcluster)  [unwired: 3 in]
  n1240 = call-by-ref "?"(reference=w9, error in=w11) -> (reference out=w13:refnum<vi>, error out=w12:errorcluster)  [unwired: 12 in]
  n1241 = Close Reference(reference=w13, error in (no error)=w12) -> ()  [unwired: 1 out]
  n1242 = while {
    stop <- FALSE stop-if-true
    n1243 = Wait (ms)(milliseconds to wait=u32 1000 ("等待时间（毫秒）")) -> ()  [unwired: 1 out]
    n1244 = case shown="真" "存校准信息" {
      frame False {
      }
      frame True {
        n1245 = local read "公式系数"() -> (w1900:dbl[])
        n1246 = local read "泵滴定数2"() -> (w1922:dbl)
        n1247 = local read "泵滴定数4"() -> (w1920:dbl)
        n1248 = local read "泵滴定数3"() -> (w1921:dbl)
        n1249 = local read "泵滴定数5"() -> (w1919:dbl)
        n1250 = local read "泵滴定数1"() -> (w1923:dbl)
        n1251 = local read "浓度1"() -> (w1929:dbl)
        n1252 = local read "浓度2"() -> (w1925:dbl)
        n1253 = local read "浓度3"() -> (w1926:dbl)
        n1254 = local read "浓度4"() -> (w1927:dbl)
        n1255 = local read "浓度5"() -> (w1928:dbl)
        n1256 = local read "标液校准时间1"() -> (w1908:timestamp)
        n1257 = local read "标液校准时间2"() -> (w1907:timestamp)
        n1258 = local read "标液校准时间3"() -> (w1906:timestamp)
        n1259 = local read "零点校准时间"() -> (w1909:timestamp)
        n1260 = local read "标液校准时间4"() -> (w1905:timestamp)
        n1261 = Build Array(w1923, w1922, w1921, w1920, w1919) -> (w1918:dbl[])
        n1262 = Build Array(w1929, w1925, w1926, w1927, w1928) -> (w1924:dbl[])
        n1263 = local write "存校准信息"(FALSE ("存校准信息")) -> ()
        n1264 = for {
          tunnel: w1900 -> [w1932] mode=indexing
          tunnel: [w1931] -> w1899 mode=indexing
          n1265 = Number To Fractional String(number=w1932, precision (6)=i16 6 ("宽度(-)")) -> (F-format string=w1931:string)  [unwired: 2 in]
        }
        n1266 = for {
          tunnel: w1924 -> [w1941] mode=indexing
          tunnel: w1918 -> [w1938] mode=indexing
          tunnel: [w1937] -> w1912 mode=indexing
          tunnel: [w1936] -> w1911 mode=indexing
          n1267 = Number To Decimal String(number=w1941, width (-)=i16 0 ("宽度(-)")) -> (decimal integer string=w1937:string)
          n1268 = Number To Decimal String(number=w1938, width (-)=i16 0 ("宽度(-)")) -> (decimal integer string=w1936:string)
        }
        n1269 = Build Array(w1909, w1908, w1907, w1906, w1905) -> (w1904:timestamp[])
        n1270 = local read "启用3"() -> (w1915:bool)
        n1271 = local read "启用5"() -> (w1913:bool)
        n1272 = local read "启用4"() -> (w1914:bool)
        n1273 = local read "启用2"() -> (w1916:bool)
        n1274 = local read "启用1"() -> (w1917:bool)
        n1275 = for {
          tunnel: w1904 -> [w1934] mode=indexing
          tunnel: [w1933] -> w1903 mode=indexing
          n1276 = Format Date/Time String(time format string (%c)="%Y/%m/%d %H:%M:%S" ("时间格式字符串(%c)"), seconds (now)=w1934) -> (date/time string=w1933:string)  [unwired: 1 in]
        }
        n1277 = Build Array(w1917, w1916, w1915, w1914, w1913) -> (w1910:bool[])
        n1278 = local read "量程选择"() -> (w1902:enum16{"低量程", "高量程"})
        n1279 = Array To Cluster(array=w1899) -> (cluster=w1898:T20)
        n1280 = call "生成校准信息.vi"("量程选择"=w1902, "公式系数"=w1898, "启用"=w1910, "校准时间"=w1903, "信号值"=w1911, "校准浓度"=w1912) -> ()  [unwired: 6 in]
      }
    }
  }
